vi "test_232_gnss.vi"() -> ()   [LabVIEW 2019]
uses:
  <vilib>/Instr/_visa.llb/VISA Configure Serial Port (Instr).vi
panel:
  out "latlong":cluster{"Lat":dbl, "Long":dbl}={"Lat"=127.14783036166666, "Long"=37.29147324166667} {"Lat" format="%.7f"; "Long" format="%.7f"}
  in  "tap":enum32{"config", "UI"}(tab)=enum."UI"
  in  "Port":refnum<visa-resource-name>="COM12"
  in  "baud rate":u32=115200 caption="rate"
  in  "data_w":string
  in  "write":bool
  in  "nmea sel":string="GNGGA"
  out "r buff":u32(graph)
  out "routh graph":cluster{"X":dbl, "Y":dbl}[](graph)=[{"X"=4629878.132195578, "Y"=6161955.791057685}, {"X"=4629878.449464146, "Y"=6161955.734831677}, {"X"=4629877.77406477, "Y"=6161955.64957599}, {"X"=-40080279.86596836, "Y"=-3607498.0192663614}, {"X"=4629879.260162596, "Y"=6161954.625048347}, {"X"=4629880.920363989, "Y"=6161953.906712205}, {"X"=4629882.6815418545, "Y"=6161954.279362187}, {"X"=4629885.113767498, "Y"=6161953.904911475}, {"X"=4629886.581793828, "Y"=6161953.689067744}, {"X"=4629888.648471416, "Y"=6161953.257648317}, {"X"=4629891.837990867, "Y"=6161952.403940227}, {"X"=4629892.308056162, "Y"=6161952.405785335}, {"X"=4629894.122102588, "Y"=6161951.952031529}, {"X"=4629897.047669123, "Y"=6161951.048930969}, {"X"=4629898.708113114, "Y"=6161950.608671173}, {"X"=4629900.550342631, "Y"=6161950.051971145}, {"X"=4629901.189738788, "Y"=6161949.965742772}, {"X"=4629902.101991517, "Y"=6161949.777960734}, {"X"=4629902.580381478, "Y"=6161949.687860983}, {"X"=4629904.337754514, "Y"=6161949.082264796}, {"X"=4629904.099145318, "Y"=6161949.2176907025}, {"X"=4629903.910121916, "Y"=6161949.322896625}, {"X"=4629904.728262869, "Y"=6161949.059576349}, {"X"=4629904.71638631, "Y"=6161949.095744023}, {"X"=4629903.057750786, "Y"=6161949.729303071}, {"X"=4629902.125000439, "Y"=6161950.056897599}, {"X"=4629901.877677887, "Y"=6161950.102282455}, {"X"=4629900.508252705, "Y"=6161950.654569676}, {"X"=4629899.9351718, "Y"=6161950.885176793}, {"X"=4629899.610600269, "Y"=6161951.011790283}, {"X"=4629898.414496481, "Y"=6161951.466995624}, {"X"=4629896.293106944, "Y"=6161952.299401729}, {"X"=4629894.940021647, "Y"=6161952.8599878205}, {"X"=4629893.374231298, "Y"=6161953.508735974}, {"X"=4629893.123720632, "Y"=6161953.679981945}, {"X"=4629891.816966376, "Y"=6161954.268541237}, {"X"=4629890.690365486, "Y"=6161954.77363618}, {"X"=4629889.518692982, "Y"=6161955.283432873}, {"X"=4629888.208123607, "Y"=6161955.87549565}, {"X"=4629886.6607548045, "Y"=6161956.478138071}, {"X"=4629884.424110745, "Y"=6161957.362093169}, {"X"=4629882.142841088, "Y"=6161958.178207771}, {"X"=4629880.10961531, "Y"=6161958.942958145}, {"X"=4629876.763268662, "Y"=6161960.222086402}, {"X"=4629875.049360155, "Y"=6161960.899303025}, {"X"=4629873.687762832, "Y"=6161961.454930634}, {"X"=4629871.788337784, "Y"=6161962.206068063}, {"X"=4629870.044529555, "Y"=6161962.864822832}, {"X"=4629867.847281659, "Y"=6161963.742002078}, {"X"=4629865.492343957, "Y"=6161964.648225941}, {"X"=4629863.853090226, "Y"=6161965.295558696}, {"X"=4629861.3459862, "Y"=6161966.254256366}, {"X"=4629859.936836349, "Y"=6161966.800689901}, {"X"=4629858.328618521, "Y"=6161967.411058061}, {"X"=4629857.052957142, "Y"=6161967.939720747}, {"X"=4629855.018113156, "Y"=6161968.737436315}, {"X"=4629853.567006, "Y"=6161969.314834981}, {"X"=4629852.811182082, "Y"=6161969.652750687}, {"X"=4629851.080375776, "Y"=6161970.33359649}, {"X"=4629849.302975364, "Y"=6161971.033939988}, {"X"=4629848.341258848, "Y"=6161971.414416122}, {"X"=4629847.05970336, "Y"=6161971.875314868}, {"X"=4629846.649667655, "Y"=6161972.050812745}, {"X"=4629845.742444542, "Y"=6161972.455482167}, {"X"=4629845.578141564, "Y"=6161972.556344009}, {"X"=4629845.343604999, "Y"=6161972.640616184}, {"X"=4629845.508885839, "Y"=6161972.50974696}, {"X"=4629845.933671053, "Y"=6161972.328983656}, {"X"=4629845.530368419, "Y"=6161972.485337485}, {"X"=4629845.479778372, "Y"=6161972.462731004}, {"X"=4629846.166837049, "Y"=6161972.1791017605}, {"X"=4629846.048558273, "Y"=6161972.174229832}, {"X"=4629846.390936594, "Y"=6161971.926570153}, {"X"=4629846.633775287, "Y"=6161971.801120852}, {"X"=4629846.453803427, "Y"=6161971.832019079}, {"X"=4629844.512919658, "Y"=6161972.565709774}, {"X"=4629843.713003393, "Y"=6161972.948996301}, {"X"=4629843.653811086, "Y"=6161972.91246725}, {"X"=4629843.375546568, "Y"=6161972.984217936}, {"X"=4629843.0636667805, "Y"=6161973.04240005}, {"X"=4629843.054895364, "Y"=6161973.014415348}, {"X"=4629842.666514361, "Y"=6161973.120696423}, {"X"=4629843.73905505, "Y"=6161972.628860625}, {"X"=4629844.410944811, "Y"=6161972.32521103}, {"X"=4629844.012114671, "Y"=6161972.416223608}, {"X"=4629845.253777034, "Y"=6161971.90422041}, {"X"=4629845.69336483, "Y"=6161971.703197987}, {"X"=4629846.419108165, "Y"=6161971.383700272}, {"X"=4629848.116545459, "Y"=6161970.716197785}, {"X"=4629848.289710002, "Y"=6161970.546360681}, {"X"=4629847.875889777, "Y"=6161970.564789061}, {"X"=4629848.5350280665, "Y"=6161970.175535598}, {"X"=4629848.471711944, "Y"=6161970.095168157}, {"X"=4629849.06439489, "Y"=6161969.810969084}, {"X"=4629849.841077642, "Y"=6161969.404897415}, {"X"=4629851.02643786, "Y"=6161968.89924651}, {"X"=4629851.683390104, "Y"=6161968.59438242}, {"X"=4629850.83990258, "Y"=6161968.794499699}, {"X"=4629851.007873055, "Y"=6161968.668487317}, {"X"=4629851.2084394125, "Y"=6161968.518731365}, {"X"=4629852.986614741, "Y"=6161967.769917846}, {"X"=4629854.014793199, "Y"=6161967.362993518}, {"X"=4629853.999855399, "Y"=6161967.318597856}, {"X"=4629855.717647278, "Y"=6161966.583931683}, {"X"=4629855.455590642, "Y"=6161966.634754253}, {"X"=4629854.855712144, "Y"=6161966.790501498}, {"X"=4629857.67515408, "Y"=6161965.669880756}, {"X"=4629857.107967277, "Y"=6161965.838523826}, {"X"=4629856.293048317, "Y"=6161966.090185709}]
  out "error out":errorcluster={"status"=FALSE, "code"=1073676294, "source"="test_232_gnss.vi 안에 VISA 읽기"} caption="에러 출력"
  out "버퍼 읽기":string
  out "val":bool
  in  "data-const":bool=TRUE
  out "문자열":string="$GNRMC,065633.00,A,3717.4853459,N,12708.8775848,E,1.804,110.01,190421,,,A,V*09\r\n$GNVTG,110.01,T,,M,1.804,N,3.340,K,A*2B\r\n$GNGGA,065633.00,3717.4853459,N,12708.8775848,E,1,05,3.98,176.567,M,18.960,M,,*47\r\n$GNGSA,A,3,14,28,30,07,,,,,,,,,8.28,3.98,7.26,1*09\r\n$GNGSA,A,3,88,,,,,,,,,,,,8.28,3.98,7.26,2*01\r\n$GNGSA,A,3,,,,,,,,,,,,,8.28,3.98,7.26,3*00\r\n$GNGSA,A,3,,,,,,,,,,,,,8.28,3.98,7.26,4*07\r\n$GPGSV,2,1,06,07,18,203,14,14,55,312,32,19,08,276,12,28,46,315,29,1*6B\r\n$GPGSV,2,2,06,30,33,243,36,41,27,238,30,1*6B\r\n$GPGSV,1,1,02,14,55,312,15,30,33,243,24,6*60\r\n$GPGSV,1,1,01,08,30,078,,0*50\r\n$GLGSV,1,1,04,78,65,279,31,81,26,262,35,88,61,326,33,,,,38,1*48\r\n$GLGSV,1,1,02,65,10,116,20,78,65,279,28,3*74\r\n$GLGSV,1,1,04,71,06,028,,72,16,073,,77,38,182,,87,40,030,,0*79\r\n$GAGSV,1,1,00,0*74\r\n$GBGSV,1,1,00,0*77\r\n$GNGLL,3717.4853459,N,12708.8775848,E,065633.00,A,A*77\r\n$GNRMC,065634.00,A,3717.4853546,N,12708.8776952,E,1.769,108.08,190421,,,A,V*0C\r\n$GNVTG,108.08,T,,M,1.769,N,3.276,K,A*2B\r\n$GNGGA,065634.00,3717.4853546,N,12708.8776952,E,1,05,3.98,176.044,M,18.960,M,,*42\r\n$GNGSA,A,3,14,28,30,07,,,,,,,,,8.28,3.98,7.26,1*09\r\n$GNGSA,A,3,88,,,,,,,,,,,,8.28,3.98,7.26,2*01\r\n$GNGSA,A,3,,,,,,,,,,,,,8.28,3.98,7.26,3*00\r\n$GNGSA,A,3,,,,,,,,,,,,,8.28,3.98,7.26,4*07\r\n$GPGSV,2,1,06,07,18,203,13,14,55,312,33,19,08,276,08,28,46,315,29,1*66\r\n$GPGSV,2,2,06,30,33,243,36,41,27,238,30,1*6B\r\n$GPGSV,1,1,02,14,55,312,15,30,33,243,24,6*60\r\n$GPGSV,1,1,01,08,30,078,,0*50\r\n$GLGSV,1,1,04,78,65,279,30,81,26,262,35,88,61,326,33,,,,36,1*47\r\n$GLGSV,1,1,02,65,10,116,18,78,65,279,27,3*70\r\n$GLGSV,1,1,04,71,06,028,,72,16,073,,77,38,182,,87,40,030,,0*79\r\n$GAGSV,1,1,00,0*74\r\n$GBGSV,1,1,00,0*77\r\n$GNGLL,3717.4853546,N,12708.8776952,E,065634.00,A,A*76\r\n$GNRMC,065635.00,A,3717.4852198,N,12708.8774654,E,1.118,,190421,,,A,V*1F\r\n$GNVTG,,T,,M,1.118,N,2.071,K,A*30\r\n$GNGGA,065635.00,3717.4852198,N,12708.8774654,E,1,06,3.35,177.168,M,18.960,M,,*44\r\n$GNGSA,A,3,14,28,30,07,,,,,,,,,6.98,3.35,6.12,1*0D\r\n$GNGSA,A,3,88,81,,,,,,,,,,,6.98,3.35,6.12,2*0C\r\n$GNGSA,A,3,,,,,,,,,,,,,6.98,3.35,6.12,3*04\r\n$GNGSA,A,3,,,,,,,,,,,,,6.98,3.35,6.12,4*03\r\n$GPGSV,2,1,06,07,18,203,11,14,55,312,32,19,08,276,10,28,46,315,29,1*6C\r\n$GPGSV,2,2,06,30,33,243,35,41,27,238,30,1*68\r\n$GPGSV,1,1,02,14,55,312,15,30,33,243,25,6*61\r\n$GPGSV,1,1,01,08,30,078,,0*50\r\n$GLGSV,1,1,04,78,65,279,29,81,26,262,33,88,61,326,32,,,,35,1*4B\r\n$GLGSV,1,1,02,65,10,116,18,78,65,279,27,3*70\r\n$GLGSV,1,1,04,71,06,028,,72,16,073,,77,38,182,,87,40,030,,0*79\r\n$GAGSV,1,1,00,0*74\r\n$GBGSV,1,1,00,0*77\r\n$GNGLL,3717.4852198,N,12708.8774654,E,065635.00,A,A*7A\r\n$GNRMC,065636.00,V,,,,,,,190421,,,N,V*16\r\n$GNVTG,,,,,,,,,N*2E\r\n$GNGGA,065636.00,,,,,0,05,15.13,,,,,,*7B\r\n$GNGSA,A,1,14,28,30,,,,,,,,,,25.70,15.13,20.78,1*34\r\n$GNGSA,A,1,88,81,,,,,,,,,,,25.70,15.13,20.78,2*32\r\n$GNGSA,A,1,,,,,,,,,,,,,25.70,15.13,20.78,3*3A\r\n$GNGSA,A,1,,,,,,,,,,,,,25.70,15.13,20.78,4*3D\r\n$GPGSV,2,1,06,07,18,203,09,14,55,312,33,19,08,276,13,28,46,315,30,1*6F\r\n$GPGSV,2,2,06,30,33,243,36,41,27,238,30,1*6B\r\n$GPGSV,1,1,02,14,55,312,14,30,33,243,25,6*60\r\n$GPGSV,1,1,01,08,30,078,,0*50\r\n$GLGSV,1,1,04,78,65,279,29,81,26,263,33,88,61,326,31,,,,35,1*49\r\n$GLGSV,1,1,02,65,10,116,18,78,65,279,28,3*7F\r\n$GLGSV,1,1,04,71,06,028,,72,16,073,,77,38,182,,87,40,030,,0*79\r\n$GAGSV,1,1,00,0*74\r\n$GBGSV,1,1,00,0*77\r\n$GNGLL,,,,,065636.00,V,N*54\r\n$GNRMC,065637.00,A,3717.4848287,N,12708.8780019,E,1.079,,190421,,,A,V*19\r\n$GNVTG,,T,,M,1.079,N,1.998,K,A*3B\r\n$GNGGA,065637.00,3717.4848287,N,12708.8780019,E,1,06,3.35,178.648,M,18.960,M,,*4E\r\n$GNGSA,A,3,14,28,30,07,,,,,,,,,6.98,3.35,6.13,1*0C\r\n$GNGSA,A,3,88,81,,,,,,,,,,,6.98,3.35,6.13,2*0D\r\n$GNGSA,A,3,,,,,,,,,,,,,6.98,3.35,6.13,3*05\r\n$GNGSA,A,3,,,,,,,,,,,,,6.98,3.35,6.13,4*02\r\n$GPGSV,2,1,06,07,18,203,10,14,55,312,33,19,08,276,12,28,46,315,30,1*66\r\n$GPGSV,2,2,06,30,33,243,35,41,27,238,30,1*68\r\n$GPGSV,1,1,02,14,55,312,14,30,33,243,25,6*60\r\n$GPGSV,1,1,01,08,30,078,,0*50\r\n$GLGSV,1,1,04,78,65,279,28,81,26,263,32,88,61,326,31,,,,34,1*48\r\n$GLGSV,1,1,02,65,10,116,19,78,65,279,28,3*7E\r\n$GLGSV,1,1,04,71,06,028,,72,16,073,,77,37,182,,87,40,030,,0*76\r\n$GAGSV,1,1,00,0*74\r\n$GBGSV,1,1,00,0*77\r\n$GNGLL,3717.4848287,N,12708.8780019,E,065637.00,A,A*7A\r\n$GNRMC,065638.00,A,3717.4846336,N,12708.8785904,E,1.071,,190421,,,A,V*1B\r\n$GNVTG,,T,,M,1.071,N,1.983,K,A*39\r\n$GNGGA,065638.00,3717.4846336,N,12708.8785904,E,1,05,3.45,179.021,M,18.960,M,,*48\r\n$GNGSA,A,3,14,28,30,07,,,,,,,,,7.40,3.45,6.55,1*0D\r\n$GNGSA,A,3,81,,,,,,,,,,,,7.40,3.45,6.55,2*0C\r\n$GNGSA,A,3,,,,,,,,,,,,,7.40,3.45,6.55,3*04\r\n$GNGSA,A,3,,,,,,,,,,,,,7.40,3.45,6.55,4*03\r\n$GPGSV,2,1,06,07,18,203,11,14,55,312,33,19,08,276,11,28,46,315,30,1*64\r\n$GPGSV,2,2,06,30,33,243,36,41,27,238,30,1*6B\r\n$GPGSV,1,1,02,14,55,312,16,30,33,243,24,6*63\r\n$GPGSV,1,1,01,08,30,078,,0*50\r\n$GLGSV,1,1,02,81,26,263,32,,,,34,1*46\r\n$GLGSV,1,1,03,65,10,116,19,78,65,278,28,88,61,326,19,3*46\r\n$GLGSV,1,1,04,71,06,028,,72,16,073,,77,37,182,,87,40,030,,0*76\r\n$GAGSV,1,1,00,0*74\r\n$GBGSV,1,1,00,0*77\r\n$GNGLL,3717.4846336,N,12708.8785904,E,065638.00,A,A*70\r\n$GNRMC,065639.00,A,3717.4850704,N,12708.8791858,E,1.002,100.47,190421,,,A,V*0D\r\n$GNVTG,100.47,T,,M,1.002,N,1.855,K,A*2B\r\n$GNGGA,065639.00,3717.4850704,N,12708.8791858,E,1,06,2.35,176.270,M,18.960,M,,*4A\r\n$GNGSA,A,3,14,28,30,07,,,,,,,,,3.41,2.35,2.46,1*08\r\n$GNGSA,A,3,79,81,,,,,,,,,,,3.41,2.35,2.46,2*07\r\n$GNGSA,A,3,,,,,,,,,,,,,3.41,2.35,2.46,3*01\r\n$GNGSA,A,3,,,,,,,,,,,,,3.41,2.35,2.46,4*06\r\n$GPGSV,2,1,06,07,18,203,12,14,55,312,33,19,08,276,10,28,46,315,29,1*6E\r\n$GPGSV,2,2,06,30,33,243,35,41,27,238,30,1*68\r\n$GPGSV,1,1,02,14,55,312,17,30,33,243,24,6*62\r\n$GPGSV,1,1,01,08,30,078,,0*50\r\n$GLGSV,1,1,02,79,,,34,81,26,263,33,1*49\r\n$GLGSV,1,1,03,65,10,116,19,78,65,278,28,88,61,326,18,3*47\r\n$GLGSV,1,1,04,71,06,028,,72,16,073,,77,37,182,,87,40,030,,0*76\r\n$GAGSV,1,1,00,0*74\r\n$GBGSV,1,1,00,0*77\r\n$GNGLL,3717.4850704,N,12708.8791858,E,065639.00,A,A*7E\r\n$GNRMC,065640.00,A,3717.4851692,N,12708.8800307,E,1.093,103.53,190421,,,A,V*04\r\n$GNVTG,103.53,T,,M,1.093,N,2.024,K,A*28\r\n$GNGGA,065640.00,3717.4851692,N,12708.8800307,E,1,06,2.35,175.043,M,18.960,M,,*4C\r\n$GNGSA,A,3,14,28,30,07,,,,,,,,,3.41,2.35,2.46,1*08\r\n$GNGSA,A,3,79,81,,,,,,,,,,,3.41,2.35,2.46,2*07\r\n$GNGSA,A,3,,,,,,,,,,,,,3.41,2.35,2.46,3*01\r\n$GNGSA,A,3,,,,,,,,,,,,,3.41,2.35,2.46,4*06\r\n$GPGSV,2,1,06,07,18,203,13,14,55,312,33,19,08,276,11,28,46,315,30,1*66\r\n$GPGSV,2,2,06,30,33,243,36,41,27,238,30,1*6B\r\n$GPGSV,1,1,02,14,55,312,17,30,33,243,24,6*62\r\n$GPGSV,1,1,01,08,30,078,,0*50\r\n$GLGSV,1,1,02,79,22,328,35,81,26,263,34,1*76\r\n$GLGSV,1,1,04,65,10,116,19,78,65,278,27,79,22,328,27,88,61,326,19,3*7C\r\n$GLGSV,1,1,04,71,06,028,,72,16,073,,77,37,182,,87,40,030,,0*76\r\n$GAGSV,1,1,00,0*74\r\n$GBGSV,1,1,00,0*77\r\n$GNGLL,3717.4851692,N,12708.8800307,E,065640.00,A,A*79\r\n$GNRMC,065641.00,A,3717.4852346,N,12708.8805404,E,0.968,104.12,190421,,,A,V*05\r\n$GNVTG,104.12,T,,M,0.968,N,1.792,K,A*2F\r\n$GNGGA,065641.00,3717.4852346,N,12708.8805404,E,1,07,2.17,174.523,M,18.960,M,,*40\r\n$GNGSA,A,3,14,28,30,07,,,,,,,,,3.08,2.17,2.19,1*0F\r\n$GNGSA,A,3,79,88,81,,,,,,,,,,3.08,2.17,2.19,2*00\r\n$GNGSA,A,3,,,,,,,,,,,,,3.08,2.17,2.19,3*06\r\n$GNGSA,A,3,,,,,,,,,,,,,3.08,2.17,2.19,4*01\r\n$GPGSV,2,1,06,07,18,203,15,14,55,312,34,19,08,276,11,28,46,315,31,1*66\r\n$GPGSV,2,2,06,30,33,243,36,41,27,238,31,1*6A\r\n$GPGSV,1,1,02,14,55,312,15,30,33,243,23,6*67\r\n$GPGSV,1,1,01,08,30,078,,0*50\r\n$GLGSV,1,1,02,79,22,328,35,81,26,263,34,1*76\r\n$GLGSV,1,1,04,65,10,116,18,78,65,278,28,79,22,328,27,88,61,326,20,3*78\r\n$GLGSV,1,1,04,71,06,028,,72,16,073,,77,37,182,,87,40,030,,0*76\r\n$GAGSV,1,1,00,0*74\r\n$GBGSV,1,1,00,0*77\r\n$GNGLL,3717.4852346,N,12708.8805404,E,065641.00,A,A*76\r\n$GNRMC,065642.00,A,3717.4852543,N,12708.8812612,E,0.932,106.63,190421,,,A,V*0D\r\n$GNVTG,106.63,T,,M,0.932,N,1.726,K,A*2B\r\n$GNGGA,065642.00,3717.4852543,N,12708.8812612,E,1,06,2.17,173.748,M,18.960,M,,*4A\r\n$GNGSA,A,3,14,28,30,07,,,,,,,,,3.08,2.17,2.19,1*0F\r\n$GNGSA,A,3,79,88,81,,,,,,,,,,3.08,2.17,2.19,2*00\r\n$GNGSA,A,3,,,,,,,,,,,,,3.08,2.17,2.19,3*06\r\n$GNGSA,A,3,,,,,,,,,,,,,3.08,2.17,2.19,4*01\r\n$GPGSV,2,1,06,07,18,203,15,14,55,312,33,19,08,276,17,28,46,315,31,1*67\r\n$GPGSV,2,2,06,30,33,243,36,41,27,238,31,1*6A\r\n$GPGSV,1,1,02,14,55,312,14,30,33,243,22,6*67\r\n$GPGSV,1,1,01,08,30,078,,0*50\r\n$GLGSV,1,1,02,79,22,328,35,81,26,263,34,1*76\r\n$GLGSV,1,1,04,65,10,116,17,78,65,278,28,79,22,328,28,88,61,326,20,3*78\r\n$GLGSV,1,1,04,71,06,028,,72,16,073,,77,37,182,,87,40,030,,0*76\r\n$GAGSV,1,1,00,0*74\r\n$GBGSV,1,1,00,0*77\r\n$GNGLL,3717.4852543,N,12708.8812612,E,065642.00,A,A*75\r\n$GNRMC,065643.00,A,3717.4851781,N,12708.8823784,E,1.067,109.96,190421,,,A,V*02\r\n$GNVTG,109.96,T,,M,1.067,N,1.977,K,A*2C\r\n$GNGGA,065643.00,3717.4851781,N,12708.8823784,E,1,06,2.17,172.534,M,18.960,M,,*40\r\n$GNGSA,A,3,14,28,30,07,,,,,,,,,3.08,2.17,2.19,1*0F\r\n$GNGSA,A,3,79,88,81,,,,,,,,,,3.08,2.17,2.19,2*00\r\n$GNGSA,A,3,,,,,,,,,,,,,3.08,2.17,2.19,3*06\r\n$GNGSA,A,3,,,,,,,,,,,,,3.08,2.17,2.19,4*01\r\n$GPGSV,2,1,06,07,18,203,16,14,55,312,33,19,08,276,14,28,46,315,31,1*67\r\n$GPGSV,2,2,06,30,33,243,36,41,27,238,30,1*6B\r\n$GPGSV,1,1,02,14,55,312,14,30,33,243,22,6*67\r\n$GPGSV,1,1,01,08,30,078,,0*50\r\n$GLGSV,1,1,02,79,22,328,35,81,26,263,33,1*71\r\n$GLGSV,1,1,04,65,10,116,18,78,65,278,27,79,22,328,27,88,61,326,21,3*76\r\n$GLGSV,1,1,04,71,06,028,,72,16,073,,77,37,182,,87,40,030,,0*76\r\n$GAGSV,1,1,00,0*74\r\n$GBGSV,1,1,00,0*77\r\n$GNGLL,3717.4851781,N,12708.8823784,E,065643.00,A,A*77\r\n$GNRMC,065644.00,A,3717.4852393,N,12708.8825398,E,0.808,106.82,190421,,,A,V*04\r\n$GNVTG,106.82,T,,M,0.808,N,1.497,K,A*25\r\n$GNGGA,065644.00,3717.4852393,N,12708.8825398,E,1,06,2.17,172.407,M,18.960,M,,*4D\r\n$GNGSA,A,3,14,28,30,07,,,,,,,,,3.08,2.17,2.19,1*0F\r\n$GNGSA,A,3,79,88,81,,,,,,,,,,3.08,2.17,2.19,2*00\r\n$GNGSA,A,3,,,,,,,,,,,,,3.08,2.17,2.19,3*06\r\n$GNGSA,A,3,,,,,,,,,,,,,3.08,2.17,2.19,4*01\r\n$GPGSV,2,1,06,07,18,203,15,14,55,312,33,19,08,276,13,28,46,315,31,1*63\r\n$GPGSV,2,2,06,30,33,243,36,41,27,238,30,1*6B\r\n$GPGSV,1,1,02,14,55,312,14,30,33,243,21,6*64\r\n$GPGSV,1,1,01,08,30,078,,0*50\r\n$GLGSV,1,1,02,79,22,328,35,81,26,263,34,1*76\r\n$GLGSV,1,1,04,65,10,116,18,78,65,278,27,79,22,328,28,88,61,326,20,3*78\r\n$GLGSV,1,1,04,71,06,028,,72,16,073,,77,37,182,,87,40,030,,0*76\r\n$GAGSV,1,1,00,0*74\r\n$GBGSV,1,1,00,0*77\r\n$GNGLL,3717.4852393,N,12708.8825398,E,065644.00,A,A*7B\r\n$GNRMC,065645.00,A,3717.4852140,N,12708.8831744,E,0.831,110.97,190421,,,A,V*00\r\n$GNVTG,110.97,T,,M,0.831,N,1.540,K,A*27\r\n$GNGGA,065645.00,3717.4852140,N,12708.8831744,E,1,06,2.17,171.708,M,18.960,M,,*4F\r\n$GNGSA,A,3,14,28,30,07,,,,,,,,,3.08,2.17,2.19,1*0F\r\n$GNGSA,A,3,79,88,81,,,,,,,,,,3.08,2.17,2.19,2*00\r\n$GNGSA,A,3,,,,,,,,,,,,,3.08,2.17,2.19,3*06\r\n$GNGSA,A,3,,,,,,,,,,,,,3.08,2.17,2.19,4*01\r\n$GPGSV,2,1,06,07,18,203,15,14,55,312,33,19,08,276,12,28,46,315,31,1*62\r\n$GPGSV,2,2,06,30,33,243,36,41,27,238,30,1*6B\r\n$GPGSV,1,1,02,14,55,312,15,30,33,243,21,6*65\r\n$GPGSV,1,1,01,08,30,078,,0*50\r\n$GLGSV,1,1,02,79,22,328,36,81,26,263,34,1*75\r\n$GLGSV,1,1,04,65,10,116,18,78,65,278,27,79,22,328,27,88,61,326,20,3*77\r\n$GLGSV,1,1,04,71,06,028,,72,16,073,,77,37,182,,87,40,030,,0*76\r\n$GAGSV,1,1,00,0*74\r\n$GBGSV,1,1,00,0*77\r\n$GNGLL,3717.4852140,N,12708.8831744,E,065645.00,A,A*76\r\n$GNRMC,065646.00,A,3717.4850760,N,12708.8842022,E,0.997,108.55,190421,,,A,V*0C\r\n$GNVTG,108.55,T,,M,0.997,N,1.846,K,A*26\r\n$GNGGA,065646.00,3717.4850760,N,12708.8842022,E,1,06,2.17,171.089,M,18.960,M,,*47\r\n$GNGSA,A,3,14,28,30,07,,,,,,,,,3.08,2.17,2.19,1*0F\r\n$GNGSA,A,3,79,88,81,,,,,,,,,,3.08,2.17,2.19,2*00\r\n$GNGSA,A,3,,,,,,,,,,,,,3.08,2.17,2.19,3*06\r\n$GNGSA,A,3,,,,,,,,,,,,,3.08,2.17,2.19,4*01\r\n$GPGSV,2,1,06,07,18,203,15,14,55,312,34,19,08,276,09,28,46,315,31,1*6F\r\n$GPGSV,2,2,06,30,33,243,36,41,27,238,31,1*6A\r\n$GPGSV,1,1,02,14,55,312,15,30,33,243,20,6*64\r\n$GPGSV,1,1,01,08,30,078,,0*50\r\n$GLGSV,1,1,02,79,22,328,36,81,26,263,34,1*75\r\n$GLGSV,1,1,04,65,10,116,18,78,65,278,27,79,22,328,27,88,61,326,21,3*76\r\n$GLGSV,1,1,04,71,06,028,,72,16,073,,77,37,182,,87,40,030,,0*76\r\n$GAGSV,1,1,00,0*74\r\n$GBGSV,1,1,00,0*77\r\n$GNGLL,3717.4850760,N,12708.8842022,E,065646.00,A,A*70\r\n$GNRMC,065647.00,A,3717.4850387,N,12708.8847837,E,0.979,109.12,190421,,,A,V*0B\r\n$GNVTG,109.12,T,,M,0.979,N,1.813,K,A*24\r\n$GNGGA,065647.00,3717.4850387,N,12708.8847837,E,1,06,2.17,170.569,M,18.960,M,,*48\r\n$GNGSA,A,3,14,28,30,07,,,,,,,,,3.08,2.17,2.19,1*0F\r\n$GNGSA,A,3,79,88,81,,,,,,,,,,3.08,2.17,2.19,2*00\r\n$GNGSA,A,3,,,,,,,,,,,,,3.08,2.17,2.19,3*06\r\n$GNGSA,A,3,,,,,,,,,,,,,3.08,2.17,2.19,4*01\r\n$GPGSV,2,1,06,07,18,203,16,14,55,312,33,19,08,276,12,28,46,315,30,1*60\r\n$GPGSV,2,2,06,30,33,243,36,41,27,238,31,1*6A\r\n$GPGSV,1,1,02,14,55,312,15,30,33,243,21,6*65\r\n$GPGSV,1,1,01,08,30,078,,0*50\r\n$GLGSV,1,1,02,79,22,328,37,81,26,263,34,1*74\r\n$GLGSV,1,1,04,65,10,116,18,78,65,278,28,79,22,328,27,88,61,327,20,3*79\r\n$GLGSV,1,1,04,71,06,028,,72,16,073,,77,37,182,,87,40,030,,0*76\r\n$GAGSV,1,1,00,0*74\r\n$GBGSV,1,1,00,0*77\r\n$GNGLL,3717.4850387,N,12708.8847837,E,065647.00,A,A*75\r\n$GNRMC,065648.00,A,3717.4849586,N,12708.8854306,E,0.899,106.80,190421,,,A,V*0B\r\n$GNVTG,106.80,T,,M,0.899,N,1.665,K,A*20\r\n$GNGGA,065648.00,3717.4849586,N,12708.8854306,E,1,07,2.17,170.188,M,18.960,M,,*49\r\n$GNGSA,A,3,14,28,30,07,,,,,,,,,3.08,2.17,2.19,1*0F\r\n$GNGSA,A,3,79,88,81,,,,,,,,,,3.08,2.17,2.19,2*00\r\n$GNGSA,A,3,,,,,,,,,,,,,3.08,2.17,2.19,3*06\r\n$GNGSA,A,3,,,,,,,,,,,,,3.08,2.17,2.19,4*01\r\n$GPGSV,2,1,06,07,18,203,16,14,55,312,33,19,08,276,15,28,46,315,30,1*67\r\n$GPGSV,2,2,06,30,33,243,35,41,27,238,30,1*68\r\n$GPGSV,1,1,02,14,55,312,16,30,33,243,22,6*65\r\n$GPGSV,1,1,01,08,30,078,,0*50\r\n$GLGSV,1,1,02,79,22,328,36,81,26,263,34,1*75\r\n$GLGSV,1,1,03,78,65,278,28,79,22,328,26,88,61,327,21,3*43\r\n$GLGSV,2,1,05,65,10,116,,71,06,028,,72,16,073,,77,37,182,,0*78\r\n$GLGSV,2,2,05,77,37,182,,0*43\r\n$GAGSV,1,1,00,0*74\r\n$GBGSV,1,1,00,0*77\r\n$GNGLL,3717.4849586,N,12708.8854306,E,065648.00,A,A*7E\r\n$GNRMC,065649.00,A,3717.4849915,N,12708.8856524,E,0.825,103.07,190421,,,A,V*05\r\n$GNVTG,103.07,T,,M,0.825,N,1.527,K,A*28\r\n$GNGGA,065649.00,3717.4849915,N,12708.8856524,E,1,06,2.17,169.994,M,18.960,M,,*46\r\n$GNGSA,A,3,14,28,30,07,,,,,,,,,3.08,2.17,2.19,1*0F\r\n$GNGSA,A,3,79,88,81,,,,,,,,,,3.08,2.17,2.19,2*00\r\n$GNGSA,A,3,,,,,,,,,,,,,3.08,2.17,2.19,3*06\r\n$GNGSA,A,3,,,,,,,,,,,,,3.08,2.17,2.19,4*01\r\n$GPGSV,2,1,06,07,18,203,15,14,55,312,33,19,08,276,11,28,46,315,29,1*68\r\n$GPGSV,2,2,06,30,33,243,35,41,27,238,31,1*69\r\n$GPGSV,1,1,02,14,55,312,17,30,33,243,22,6*64\r\n$GPGSV,1,1,01,08,30,078,,0*50\r\n$GLGSV,1,1,02,79,22,328,36,81,26,263,33,1*72\r\n$GLGSV,1,1,04,78,65,278,27,79,22,328,26,81,26,263,19,88,61,327,21,3*79\r\n$GLGSV,2,1,05,65,10,116,,71,06,028,,72,16,073,,77,37,182,,0*78\r\n$GLGSV,2,2,05,77,37,182,,0*43\r\n$GAGSV,1,1,00,0*74\r\n$GBGSV,1,1,00,0*77\r\n$GNGLL,3717.4849915,N,12708.8856524,E,065649.00,A,A*7D\r\n$GNRMC,065650.00,A,3717.4850017,N,12708.8859705,E,0.780,,190421,,,A,V*1B\r\n$GNVTG,,T,,M,0.780,N,1.444,K,A*37\r\n$GNGGA,065650.00,3717.4850017,N,12708.8859705,E,1,06,2.17,169.716,M,18.960,M,,*47\r\n$GNGSA,A,3,14,28,30,07,,,,,,,,,3.08,2.17,2.19,1*0F\r\n$GNGSA,A,3,79,88,81,,,,,,,,,,3.08,2.17,2.19,2*00\r\n$GNGSA,A,3,,,,,,,,,,,,,3.08,2.17,2.19,3*06\r\n$GNGSA,A,3,,,,,,,,,,,,,3.08,2.17,2.19,4*01\r\n$GPGSV,2,1,06,07,18,203,14,14,55,312,33,19,08,276,14,28,46,315,28,1*6D\r\n$GPGSV,2,2,06,30,33,243,35,41,27,238,31,1*69\r\n$GPGSV,1,1,02,14,55,312,18,30,33,243,22,6*6B\r\n$GPGSV,1,1,01,08,30,078,,0*50\r\n$GLGSV,1,1,02,79,22,328,36,81,26,263,33,1*72\r\n$GLGSV,1,1,04,78,65,278,27,79,22,328,26,81,26,263,19,88,61,327,20,3*78\r\n$GLGSV,2,1,05,65,10,116,,71,06,028,,72,16,073,,77,37,182,,0*78\r\n$GLGSV,2,2,05,77,37,182,,0*43\r\n$GAGSV,1,1,00,0*74\r\n$GBGSV,1,1,00,0*77\r\n$GNGLL,3717.4850017,N,12708.8859705,E,065650.00,A,A*78\r\n$GNRMC,065651.00,A,3717.4850118,N,12708.8861371,E,0.670,,190421,,,A,V*16\r\n$GNVTG,,T,,M,0.670,N,1.240,K,A*3B\r\n$GNGGA,065651.00,3717.4850118,N,12708.8861371,E,1,07,2.17,169.601,M,18.960,M,,*42\r\n$GNGSA,A,3,14,28,30,07,,,,,,,,,3.08,2.17,2.19,1*0F\r\n$GNGSA,A,3,79,88,81,,,,,,,,,,3.08,2.17,2.19,2*00\r\n$GNGSA,A,3,,,,,,,,,,,,,3.08,2.17,2.19,3*06\r\n$GNGSA,A,3,,,,,,,,,,,,,3.08,2.17,2.19,4*01\r\n$GPGSV,2,1,06,07,18,203,14,14,55,312,33,19,08,276,08,28,46,315,28,1*60\r\n$GPGSV,2,2,06,30,33,243,35,41,27,238,30,1*68\r\n$GPGSV,1,1,02,14,55,312,17,30,33,243,23,6*65\r\n$GPGSV,1,1,01,08,30,078,,0*50\r\n$GLGSV,1,1,02,79,22,328,35,81,26,263,33,1*71\r\n$GLGSV,2,1,05,65,10,116,20,78,65,278,27,79,22,328,26,81,26,263,19,3*7F\r\n$GLGSV,2,2,05,88,61,327,21,3*4D\r\n$GLGSV,1,1,04,71,06,028,,72,16,073,,77,37,182,,87,40,030,,0*76\r\n$GAGSV,1,1,00,0*74\r\n$GBGSV,1,1,00,0*77\r\n$GNGLL,3717.4850118,N,12708.8861371,E,065651.00,A,A*7B\r\n$GNRMC,065652.00,A,3717.4848931,N,12708.8867561,E,0.731,,190421,,,A,V*1A\r\n$GNVTG,,T,,M,0.731,N,1.354,K,A*3B\r\n$GNGGA,065652.00,3717.4848931,N,12708.8867561,E,1,07,2.17,169.223,M,18.960,M,,*4E\r\n$GNGSA,A,3,14,28,30,07,,,,,,,,,3.08,2.17,2.19,1*0F\r\n$GNGSA,A,3,79,88,81,,,,,,,,,,3.08,2.17,2.19,2*00\r\n$GNGSA,A,3,,,,,,,,,,,,,3.08,2.17,2.19,3*06\r\n$GNGSA,A,3,,,,,,,,,,,,,3.08,2.17,2.19,4*01\r\n$GPGSV,2,1,06,07,18,202,16,14,55,312,33,19,08,276,10,28,46,315,28,1*6A\r\n$GPGSV,2,2,06,30,33,243,35,41,27,238,31,1*69\r\n$GPGSV,1,1,02,14,55,312,16,30,33,243,23,6*64\r\n$GPGSV,1,1,01,08,30,078,,0*50\r\n$GLGSV,1,1,03,79,22,328,34,81,26,263,33,88,61,327,33,1*40\r\n$GLGSV,2,1,05,65,10,116,18,78,65,278,27,79,22,328,25,81,26,263,19,3*77\r\n$GLGSV,2,2,05,88,61,327,21,3*4D\r\n$GLGSV,1,1,04,71,06,028,,72,16,073,,77,37,182,,87,40,030,,0*76\r\n$GAGSV,1,1,00,0*74\r\n$GBGSV,1,1,00,0*77\r\n$GNGLL,3717.4848931,N,12708.8867561,E,065652.00,A,A*73\r\n$GNRMC,065653.00,A,3717.4849394,N,12708.8866707,E,0.597,,190421,,,A,V*12\r\n$GNVTG,,T,,M,0.597,N,1.105,K,A*33\r\n$GNGGA,065653.00,3717.4849394,N,12708.8866707,E,1,07,2.17,169.235,M,18.960,M,,*4F\r\n$GNGSA,A,3,14,28,30,07,,,,,,,,,3.08,2.17,2.19,1*0F\r\n$GNGSA,A,3,79,88,81,,,,,,,,,,3.08,2.17,2.19,2*00\r\n$GNGSA,A,3,,,,,,,,,,,,,3.08,2.17,2.19,3*06\r\n$GNGSA,A,3,,,,,,,,,,,,,3.08,2.17,2.19,4*01\r\n$GPGSV,2,1,06,07,18,202,17,14,55,312,33,19,08,276,10,28,46,315,29,1*6A\r\n$GPGSV,2,2,06,30,33,243,35,41,27,238,31,1*69\r\n$GPGSV,1,1,02,14,55,312,16,30,33,243,22,6*65\r\n$GPGSV,1,1,01,08,29,078,,0*58\r\n$GLGSV,1,1,03,79,22,328,34,81,26,263,33,88,61,327,32,1*41\r\n$GLGSV,2,1,05,65,10,116,17,78,65,278,26,79,22,328,25,81,26,263,18,3*78\r\n$GLGSV,2,2,05,88,61,327,20,3*4C\r\n$GLGSV,1,1,04,71,06,028,,72,16,073,,77,37,182,,87,40,030,,0*76\r\n$GAGSV,1,1,00,0*74\r\n$GBGSV,1,1,00,0*77\r\n$GNGLL,3717.4849394,N,12708.8866707,E,065653.00,A,A*75\r\n$GNRMC,065654.00,A,3717.4849749,N,12708.8866031,E,0.514,,190421,,,A,V*18\r\n$GNVTG,,T,,M,0.514,N,0.953,K,A*32\r\n$GNGGA,065654.00,3717.4849749,N,12708.8866031,E,1,07,2.17,169.195,M,18.960,M,,*47\r\n$GNGSA,A,3,14,28,30,07,,,,,,,,,3.08,2.17,2.19,1*0F\r\n$GNGSA,A,3,79,88,81,,,,,,,,,,3.08,2.17,2.19,2*00\r\n$GNGSA,A,3,,,,,,,,,,,,,3.08,2.17,2.19,3*06\r\n$GNGSA,A,3,,,,,,,,,,,,,3.08,2.17,2.19,4*01\r\n$GPGSV,2,1,06,07,18,202,18,14,55,312,33,19,08,276,14,28,46,315,29,1*61\r\n$GPGSV,2,2,06,30,33,243,34,41,27,238,31,1*68\r\n$GPGSV,1,1,02,14,55,312,16,30,33,243,22,6*65\r\n$GPGSV,1,1,01,08,29,078,,0*58\r\n$GLGSV,1,1,03,79,22,328,34,81,26,263,33,88,61,327,32,1*41\r\n$GLGSV,2,1,05,65,10,116,15,78,65,278,26,79,22,328,25,81,26,263,19,3*7B\r\n$GLGSV,2,2,05,88,61,327,20,3*4C\r\n$GLGSV,1,1,04,71,06,028,,72,16,073,,77,37,182,,87,40,030,,0*76\r\n$GAGSV,1,1,00,0*74\r\n$GBGSV,1,1,00,0*77\r\n$GNGLL,3717.4849749,N,12708.8866031,E,065654.00,A,A*74\r\n$GNRMC,065655.00,A,3717.4849302,N,12708.8868908,E,0.661,,190421,,,A,V*1E\r\n$GNVTG,,T,,M,0.661,N,1.224,K,A*39\r\n$GNGGA,065655.00,3717.4849302,N,12708.8868908,E,1,07,2.17,169.152,M,18.960,M,,*4B\r\n$GNGSA,A,3,14,28,30,07,,,,,,,,,3.08,2.17,2.19,1*0F\r\n$GNGSA,A,3,79,88,81,,,,,,,,,,3.08,2.17,2.19,2*00\r\n$GNGSA,A,3,,,,,,,,,,,,,3.08,2.17,2.19,3*06\r\n$GNGSA,A,3,,,,,,,,,,,,,3.08,2.17,2.19,4*01\r\n$GPGSV,2,1,06,07,18,202,18,14,55,312,32,19,08,276,06,28,46,315,28,1*62\r\n$GPGSV,2,2,06,30,33,243,34,41,27,238,31,1*68\r\n$GPGSV,1,1,02,14,55,312,17,30,33,243,23,6*65\r\n$GPGSV,1,1,01,08,29,078,,0*58\r\n$GLGSV,1,1,03,79,22,328,34,81,26,263,33,88,61,327,32,1*41\r\n$GLGSV,2,1,05,65,10,116,13,78,65,278,26,79,22,328,24,81,26,263,19,3*7C\r\n$GLGSV,2,2,05,88,61,327,18,3*47\r\n$GLGSV,1,1,04,71,06,028,,72,16,073,,77,37,182,,87,40,030,,0*76\r\n$GAGSV,1,1,00,0*74\r\n$GBGSV,1,1,00,0*77\r\n$GNGLL,3717.4849302,N,12708.8868908,E,065655.00,A,A*73\r\n$GNRMC,065656.00,A,3717.4849492,N,12708.8868858,E,0.462,,190421,,,A,V*16\r\n$GNVTG,,T,,M,0.462,N,0.855,K,A*35\r\n$GNGGA,065656.00,3717.4849492,N,12708.8868858,E,1,07,2.17,169.187,M,18.960,M,,*4A\r\n$GNGSA,A,3,14,28,30,07,,,,,,,,,3.08,2.17,2.19,1*0F\r\n$GNGSA,A,3,79,88,81,,,,,,,,,,3.08,2.17,2.19,2*00\r\n$GNGSA,A,3,,,,,,,,,,,,,3.08,2.17,2.19,3*06\r\n$GNGSA,A,3,,,,,,,,,,,,,3.08,2.17,2.19,4*01\r\n$GPGSV,2,1,06,07,18,202,19,14,55,312,33,19,08,276,08,28,46,315,28,1*6C\r\n$GPGSV,2,2,06,30,33,243,35,41,27,238,30,1*68\r\n$GPGSV,1,1,02,14,55,312,17,30,33,243,22,6*64\r\n$GPGSV,1,1,01,08,29,078,,0*58\r\n$GLGSV,1,1,03,79,22,328,34,81,26,263,33,88,61,327,32,1*41\r\n$GLGSV,2,1,05,65,10,116,12,78,65,278,26,79,22,328,24,81,26,263,18,3*7C\r\n$GLGSV,2,2,05,88,61,327,18,3*47\r\n$GLGSV,1,1,04,71,06,028,,72,16,073,,77,37,182,,87,40,030,,0*76\r\n$GAGSV,1,1,00,0*74\r\n$GBGSV,1,1,00,0*77\r\n$GNGLL,3717.4849492,N,12708.8868858,E,065656.00,A,A*7A\r\n$GNRMC,065657.00,A,3717.4850964,N,12708.8863000,E,0.600,,190421,,,A,V*13\r\n$GNVTG,,T,,M,0.600,N,1.111,K,A*3B\r\n$GNGGA,065657.00,3717.4850964,N,12708.8863000,E,1,07,2.17,169.080,M,18.960,M,,*4F\r\n$GNGSA,A,3,14,28,30,07,,,,,,,,,3.08,2.17,2.19,1*0F\r\n$GNGSA,A,3,79,88,81,,,,,,,,,,3.08,2.17,2.19,2*00\r\n$GNGSA,A,3,,,,,,,,,,,,,3.08,2.17,2.19,3*06\r\n$GNGSA,A,3,,,,,,,,,,,,,3.08,2.17,2.19,4*01\r\n$GPGSV,2,1,06,07,18,202,19,14,55,312,33,19,08,276,09,28,46,315,28,1*6D\r\n$GPGSV,2,2,06,30,33,243,34,41,27,238,31,1*68\r\n$GPGSV,1,1,02,14,55,312,18,30,33,243,22,6*6B\r\n$GPGSV,1,1,01,08,29,078,,0*58\r\n$GLGSV,1,1,03,79,22,328,34,81,26,263,33,88,61,327,32,1*41\r\n$GLGSV,2,1,05,65,10,116,14,78,65,278,26,79,22,328,24,81,26,263,17,3*75\r\n$GLGSV,2,2,05,88,61,327,18,3*47\r\n$GLGSV,1,1,04,71,06,028,,72,16,073,,77,37,182,,87,40,030,,0*76\r\n$GAGSV,1,1,00,0*74\r\n$GBGSV,1,1,00,0*77\r\n$GNGLL,3717.4850964,N,12708.8863000,E,065657.00,A,A*79\r\n$GNRMC,065658.00,A,3717.4851629,N,12708.8859713,E,0.578,,190421,,,A,V*1B\r\n$GNVTG,,T,,M,0.578,N,1.070,K,A*31\r\n$GNGGA,065658.00,3717.4851629,N,12708.8859713,E,1,07,2.17,168.743,M,18.960,M,,*42\r\n$GNGSA,A,3,14,28,30,07,,,,,,,,,3.08,2.17,2.19,1*0F\r\n$GNGSA,A,3,79,88,81,,,,,,,,,,3.08,2.17,2.19,2*00\r\n$GNGSA,A,3,,,,,,,,,,,,,3.08,2.17,2.19,3*06\r\n$GNGSA,A,3,,,,,,,,,,,,,3.08,2.17,2.19,4*01\r\n$GPGSV,2,1,06,07,18,202,19,14,56,312,33,19,08,276,07,28,46,315,28,1*60\r\n$GPGSV,2,2,06,30,33,243,34,41,27,238,31,1*68\r\n$GPGSV,1,1,02,14,56,312,18,30,33,243,22,6*68\r\n$GPGSV,1,1,01,08,29,078,,0*58\r\n$GLGSV,1,1,03,79,22,328,33,81,26,263,33,88,61,327,32,1*46\r\n$GLGSV,2,1,05,65,10,116,15,78,65,278,26,79,22,328,24,81,26,263,18,3*7B\r\n$GLGSV,2,2,05,88,61,327,19,3*46\r\n$GLGSV,1,1,04,71,06,028,,72,16,073,,77,37,182,,87,40,030,,0*76\r\n$GAGSV,1,1,00,0*74\r\n$GBGSV,1,1,00,0*77\r\n$GNGLL,3717.4851629,N,12708.8859713,E,065658.00,A,A*7D\r\n$GNRMC,065659.00,A,3717.4851570,N,12708.8858852,E,0.638,,190421,,,A,V*19\r\n$GNVTG,,T,,M,0.638,N,1.182,K,A*3A\r\n$GNGGA,065659.00,3717.4851570,N,12708.8858852,E,1,07,2.17,168.385,M,18.960,M,,*49\r\n$GNGSA,A,3,14,28,30,07,,,,,,,,,3.08,2.17,2.19,1*0F\r\n$GNGSA,A,3,79,88,81,,,,,,,,,,3.08,2.17,2.19,2*00\r\n$GNGSA,A,3,,,,,,,,,,,,,3.08,2.17,2.19,3*06\r\n$GNGSA,A,3,,,,,,,,,,,,,3.08,2.17,2.19,4*01\r\n$GPGSV,2,1,06,07,18,202,19,14,56,312,33,19,08,276,07,28,46,315,28,1*60\r\n$GPGSV,2,2,06,30,33,243,34,41,27,238,31,1*68\r\n$GPGSV,1,1,02,14,56,312,17,30,33,243,22,6*67\r\n$GPGSV,1,1,01,08,29,078,,0*58\r\n$GLGSV,1,1,03,79,22,328,32,81,26,263,32,88,61,327,31,1*45\r\n$GLGSV,2,1,05,65,10,116,15,78,65,278,26,79,22,328,25,81,26,263,19,3*7B\r\n$GLGSV,2,2,05,88,61,327,19,3*46\r\n$GLGSV,1,1,04,71,06,028,,72,16,073,,77,37,182,,87,40,030,,0*76\r\n$GAGSV,1,1,00,0*74\r\n$GBGSV,1,1,00,0*77\r\n$GNGLL,3717.4851570,N,12708.8858852,E,065659.00,A,A*78\r\n$GNRMC,065700.00,A,3717.4852951,N,12708.8854008,E,0.452,,190421,,,A,V*1D\r\n$GNVTG,,T,,M,0.452,N,0.837,K,A*32\r\n$GNGGA,065700.00,3717.4852951,N,12708.8854008,E,1,06,2.17,168.776,M,18.960,M,,*4A\r\n$GNGSA,A,3,14,28,30,07,,,,,,,,,3.08,2.17,2.19,1*0F\r\n$GNGSA,A,3,79,88,81,,,,,,,,,,3.08,2.17,2.19,2*00\r\n$GNGSA,A,3,,,,,,,,,,,,,3.08,2.17,2.19,3*06\r\n$GNGSA,A,3,,,,,,,,,,,,,3.08,2.17,2.19,4*01\r\n$GPGSV,2,1,06,07,18,202,20,14,56,312,33,19,08,276,10,28,46,315,28,1*6C\r\n$GPGSV,2,2,06,30,33,243,34,41,27,238,31,1*68\r\n$GPGSV,1,1,02,14,56,312,18,30,33,243,23,6*69\r\n$GPGSV,1,1,01,08,29,078,,0*58\r\n$GLGSV,1,1,02,79,22,328,32,81,26,263,32,1*77\r\n$GLGSV,2,1,05,65,10,116,14,78,65,278,27,79,22,328,24,81,26,263,19,3*7A\r\n$GLGSV,2,2,05,88,61,327,19,3*46\r\n$GLGSV,1,1,04,71,06,028,,72,16,073,,77,37,182,,87,40,030,,0*76\r\n$GAGSV,1,1,00,0*74\r\n$GBGSV,1,1,00,0*77\r\n$GNGLL,3717.4852951,N,12708.8854008,E,065700.00,A,A*72\r\n$GNRMC,065701.00,A,3717.4853526,N,12708.8851981,E,0.524,,190421,,,A,V*1C\r\n$GNVTG,,T,,M,0.524,N,0.971,K,A*31\r\n$GNGGA,065701.00,3717.4853526,N,12708.8851981,E,1,06,2.17,169.007,M,18.960,M,,*4B\r\n$GNGSA,A,3,14,28,30,07,,,,,,,,,3.08,2.17,2.19,1*0F\r\n$GNGSA,A,3,79,88,81,,,,,,,,,,3.08,2.17,2.19,2*00\r\n$GNGSA,A,3,,,,,,,,,,,,,3.08,2.17,2.19,3*06\r\n$GNGSA,A,3,,,,,,,,,,,,,3.08,2.17,2.19,4*01\r\n$GPGSV,2,1,06,07,18,202,21,14,56,312,33,19,08,276,07,28,46,315,27,1*64\r\n$GPGSV,2,2,06,30,33,243,34,41,27,238,31,1*68\r\n$GPGSV,1,1,02,14,56,312,18,30,33,243,24,6*6E\r\n$GPGSV,1,1,01,08,29,078,,0*58\r\n$GLGSV,1,1,02,79,22,328,32,81,26,263,32,1*77\r\n$GLGSV,2,1,05,65,10,116,13,78,65,278,26,79,22,328,24,81,26,263,20,3*76\r\n$GLGSV,2,2,05,88,61,327,19,3*46\r\n$GLGSV,1,1,04,71,06,028,,72,16,073,,77,37,182,,87,40,030,,0*76\r\n$GAGSV,1,1,00,0*74\r\n$GBGSV,1,1,00,0*77\r\n$GNGLL,3717.4853526,N,12708.8851981,E,065701.00,A,A*73\r\n$GNRMC,065702.00,A,3717.4853829,N,12708.8850834,E,0.558,,190421,,,A,V*18\r\n$GNVTG,,T,,M,0.558,N,1.034,K,A*33\r\n$GNGGA,065702.00,3717.4853829,N,12708.8850834,E,1,06,2.17,169.144,M,18.960,M,,*42\r\n$GNGSA,A,3,14,28,30,07,,,,,,,,,3.08,2.17,2.19,1*0F\r\n$GNGSA,A,3,79,88,81,,,,,,,,,,3.08,2.17,2.19,2*00\r\n$GNGSA,A,3,,,,,,,,,,,,,3.08,2.17,2.19,3*06\r\n$GNGSA,A,3,,,,,,,,,,,,,3.08,2.17,2.19,4*01\r\n$GPGSV,2,1,06,07,18,202,22,14,56,312,32,19,08,276,10,28,46,315,27,1*60\r\n$GPGSV,2,2,06,30,33,243,34,41,27,238,31,1*68\r\n$GPGSV,1,1,02,14,56,312,19,30,33,243,24,6*6F\r\n$GPGSV,1,1,01,08,29,078,,0*58\r\n$GLGSV,1,1,02,79,22,328,32,81,26,263,32,1*77\r\n$GLGSV,2,1,05,65,10,116,14,78,65,278,26,79,22,328,25,81,26,263,20,3*70\r\n$GLGSV,2,2,05,88,61,327,20,3*4C\r\n$GLGSV,1,1,04,71,06,028,,72,16,073,,77,37,182,,87,40,030,,0*76\r\n$GAGSV,1,1,00,0*74\r\n$GBGSV,1,1,00,0*77\r\n$GNGLL,3717.4853829,N,12708.8850834,E,065702.00,A,A*7C\r\n$GNRMC,065703.00,A,3717.4854881,N,12708.8846610,E,0.505,,190421,,,A,V*1B\r\n$GNVTG,,T,,M,0.505,N,0.934,K,A*33\r\n$GNGGA,065703.00,3717.4854881,N,12708.8846610,E,1,07,2.17,169.484,M,18.960,M,,*41\r\n$GNGSA,A,3,14,28,30,07,,,,,,,,,3.08,2.17,2.19,1*0F\r\n$GNGSA,A,3,79,88,81,,,,,,,,,,3.08,2.17,2.19,2*00\r\n$GNGSA,A,3,,,,,,,,,,,,,3.08,2.17,2.19,3*06\r\n$GNGSA,A,3,,,,,,,,,,,,,3.08,2.17,2.19,4*01\r\n$GPGSV,2,1,06,07,18,202,22,14,56,312,32,19,08,276,12,28,47,315,26,1*62\r\n$GPGSV,2,2,06,30,33,243,34,41,27,238,31,1*68\r\n$GPGSV,1,1,02,14,56,312,17,30,33,243,24,6*61\r\n$GPGSV,1,1,01,08,29,078,,0*58\r\n$GLGSV,1,1,02,79,22,328,32,81,26,263,32,1*77\r\n$GLGSV,1,1,04,65,10,116,15,78,65,278,26,81,26,263,20,88,61,327,20,3*70\r\n$GLGSV,1,1,04,71,06,028,,72,16,073,,77,37,182,,87,40,030,,0*76\r\n$GAGSV,1,1,00,0*74\r\n$GBGSV,1,1,00,0*77\r\n$GNGLL,3717.4854881,N,12708.8846610,E,065703.00,A,A*77\r\n$GNRMC,065704.00,A,3717.4856889,N,12708.8839112,E,0.400,,190421,,,A,V*1F\r\n$GNVTG,,T,,M,0.400,N,0.741,K,A*3B\r\n$GNGGA,065704.00,3717.4856889,N,12708.8839112,E,1,06,2.17,170.032,M,18.960,M,,*41\r\n$GNGSA,A,3,14,28,30,07,,,,,,,,,3.08,2.17,2.19,1*0F\r\n$GNGSA,A,3,79,88,81,,,,,,,,,,3.08,2.17,2.19,2*00\r\n$GNGSA,A,3,,,,,,,,,,,,,3.08,2.17,2.19,3*06\r\n$GNGSA,A,3,,,,,,,,,,,,,3.08,2.17,2.19,4*01\r\n$GPGSV,2,1,06,07,18,202,21,14,56,312,32,19,08,276,07,28,47,315,26,1*65\r\n$GPGSV,2,2,06,30,33,243,34,41,27,238,30,1*69\r\n$GPGSV,1,1,02,14,56,312,17,30,33,243,23,6*66\r\n$GPGSV,1,1,01,08,29,078,,0*58\r\n$GLGSV,1,1,02,79,22,328,32,81,26,263,32,1*77\r\n$GLGSV,2,1,05,65,10,116,15,78,65,278,26,79,22,328,25,81,26,263,20,3*71\r\n$GLGSV,2,2,05,88,61,327,20,3*4C\r\n$GLGSV,1,1,04,71,06,028,,72,16,073,,77,37,182,,87,40,030,,0*76\r\n$GAGSV,1,1,00,0*74\r\n$GBGSV,1,1,00,0*77\r\n$GNGLL,3717.4856889,N,12708.8839112,E,065704.00,A,A*77\r\n$GNRMC,065705.00,A,3717.4858338,N,12708.8834322,E,0.317,,190421,,,A,V*1C\r\n$GNVTG,,T,,M,0.317,N,0.588,K,A*3D\r\n$GNGGA,065705.00,3717.4858338,N,12708.8834322,E,1,06,2.17,170.264,M,18.960,M,,*42\r\n$GNGSA,A,3,14,28,30,07,,,,,,,,,3.08,2.17,2.20,1*05\r\n$GNGSA,A,3,79,88,81,,,,,,,,,,3.08,2.17,2.20,2*0A\r\n$GNGSA,A,3,,,,,,,,,,,,,3.08,2.17,2.20,3*0C\r\n$GNGSA,A,3,,,,,,,,,,,,,3.08,2.17,2.20,4*0B\r\n$GPGSV,2,1,06,07,18,202,21,14,56,312,33,19,08,276,10,28,47,315,26,1*62\r\n$GPGSV,2,2,06,30,33,243,34,41,27,238,31,1*68\r\n$GPGSV,1,1,02,14,56,312,17,30,33,243,23,6*66\r\n$GPGSV,1,1,01,08,29,078,,0*58\r\n$GLGSV,1,1,02,79,22,328,33,81,26,263,32,1*76\r\n$GLGSV,2,1,05,65,10,116,16,78,65,278,27,79,22,328,25,81,26,263,20,3*73\r\n$GLGSV,2,2,05,88,61,327,20,3*4C\r\n$GLGSV,1,1,04,71,06,028,,72,16,073,,77,37,182,,87,40,030,,0*76\r\n$GAGSV,1,1,00,0*74\r\n$GBGSV,1,1,00,0*77\r\n$GNGLL,3717.4858338,N,12708.8834322,E,065705.00,A,A*75\r\n$GNRMC,065706.00,A,3717.4860015,N,12708.8828779,E,0.275,,190421,,,A,V*1A\r\n$GNVTG,,T,,M,0.275,N,0.510,K,A*39\r\n$GNGGA,065706.00,3717.4860015,N,12708.8828779,E,1,06,2.17,170.758,M,18.960,M,,*4B\r\n$GNGSA,A,3,14,28,30,07,,,,,,,,,3.08,2.17,2.20,1*05\r\n$GNGSA,A,3,79,88,81,,,,,,,,,,3.08,2.17,2.20,2*0A\r\n$GNGSA,A,3,,,,,,,,,,,,,3.08,2.17,2.20,3*0C\r\n$GNGSA,A,3,,,,,,,,,,,,,3.08,2.17,2.20,4*0B\r\n$GPGSV,2,1,06,07,18,202,22,14,56,312,33,19,08,276,14,28,47,315,26,1*65\r\n$GPGSV,2,2,06,30,33,243,34,41,27,238,31,1*68\r\n$GPGSV,1,1,02,14,56,312,17,30,33,243,23,6*66\r\n$GPGSV,1,1,01,08,29,078,,0*58\r\n$GLGSV,1,1,02,79,22,328,33,81,26,263,33,1*77\r\n$GLGSV,2,1,05,65,10,116,16,78,65,278,27,79,22,328,25,81,26,263,20,3*73\r\n$GLGSV,2,2,05,88,61,327,20,3*4C\r\n$GLGSV,1,1,04,71,06,028,,72,16,073,,77,37,182,,87,40,030,,0*76\r\n$GAGSV,1,1,00,0*74\r\n$GBGSV,1,1,00,0*77\r\n$GNGLL,3717.4860015,N,12708.8828779,E,065706.00,A,A*76\r\n$GNRMC,065707.00,A,3717.4860666,N,12708.8827875,E,0.349,,190421,,,A,V*1B\r\n$GNVTG,,T,,M,0.349,N,0.647,K,A*36\r\n$GNGGA,065707.00,3717.4860666,N,12708.8827875,E,1,06,2.17,171.108,M,18.960,M,,*46\r\n$GNGSA,A,3,14,28,30,07,,,,,,,,,3.08,2.17,2.20,1*05\r\n$GNGSA,A,3,79,88,81,,,,,,,,,,3.08,2.17,2.20,2*0A\r\n$GNGSA,A,3,,,,,,,,,,,,,3.08,2.17,2.20,3*0C\r\n$GNGSA,A,3,,,,,,,,,,,,,3.08,2.17,2.20,4*0B\r\n$GPGSV,2,1,06,07,18,202,22,14,56,312,32,19,08,276,10,28,47,315,26,1*60\r\n$GPGSV,2,2,06,30,33,243,34,41,27,238,30,1*69\r\n$GPGSV,1,1,02,14,56,312,17,30,33,243,23,6*66\r\n$GPGSV,1,1,01,08,29,078,,0*58\r\n$GLGSV,1,1,02,79,22,328,34,81,26,263,34,1*77\r\n$GLGSV,2,1,05,65,10,116,17,78,65,278,27,79,22,328,26,81,26,263,20,3*71\r\n$GLGSV,2,2,05,88,61,327,19,3*46\r\n$GLGSV,1,1,04,71,06,028,,72,16,073,,77,37,182,,87,40,030,,0*76\r\n$GAGSV,1,1,00,0*74\r\n$GBGSV,1,1,00,0*77\r\n$GNGLL,3717.4860666,N,12708.8827875,E,065707.00,A,A*79\r\n$GNRMC,065708.00,A,3717.4862333,N,12708.8823237,E,0.268,,190421,,,A,V*19\r\n$GNVTG,,T,,M,0.268,N,0.496,K,A*3A\r\n$GNGGA,065708.00,3717.4862333,N,12708.8823237,E,1,06,2.17,171.619,M,18.960,M,,*41\r\n$GNGSA,A,3,14,28,30,07,,,,,,,,,3.08,2.17,2.20,1*05\r\n$GNGSA,A,3,79,88,81,,,,,,,,,,3.08,2.17,2.20,2*0A\r\n$GNGSA,A,3,,,,,,,,,,,,,3.08,2.17,2.20,3*0C\r\n$GNGSA,A,3,,,,,,,,,,,,,3.08,2.17,2.20,4*0B\r\n$GPGSV,2,1,06,07,18,202,22,14,56,312,33,19,08,276,09,28,47,315,25,1*6A\r\n$GPGSV,2,2,06,30,33,243,33,41,27,238,30,1*6E\r\n$GPGSV,1,1,02,14,56,312,18,30,33,243,24,6*6E\r\n$GPGSV,1,1,01,08,29,078,,0*58\r\n$GLGSV,1,1,02,79,22,328,34,81,26,263,34,1*77\r\n$GLGSV,2,1,05,65,10,116,15,78,65,278,27,79,22,328,25,81,26,263,20,3*70\r\n$GLGSV,2,2,05,88,61,327,19,3*46\r\n$GLGSV,1,1,04,71,06,028,,72,16,073,,77,37,182,,87,40,030,,0*76\r\n$GAGSV,1,1,00,0*74\r\n$GBGSV,1,1,00,0*77\r\n$GNGLL,3717.4862333,N,12708.8823237,E,065708.00,A,A*79\r\n$GNRMC,065709.00,A,3717.4863757,N,12708.8819239,E,0.329,,190421,,,A,V*1C\r\n$GNVTG,,T,,M,0.329,N,0.610,K,A*32\r\n$GNGGA,065709.00,3717.4863757,N,12708.8819239,E,1,06,2.17,172.107,M,18.960,M,,*4B\r\n$GNGSA,A,3,14,28,30,07,,,,,,,,,3.08,2.17,2.20,1*05\r\n$GNGSA,A,3,79,88,81,,,,,,,,,,3.08,2.17,2.20,2*0A\r\n$GNGSA,A,3,,,,,,,,,,,,,3.08,2.17,2.20,3*0C\r\n$GNGSA,A,3,,,,,,,,,,,,,3.08,2.17,2.20,4*0B\r\n$GPGSV,2,1,06,07,18,202,22,14,56,312,33,19,08,276,09,28,47,315,25,1*6A\r\n$GPGSV,2,2,06,30,33,243,33,41,27,238,30,1*6E\r\n$GPGSV,1,1,02,14,56,312,18,30,33,243,24,6*6E\r\n$GPGSV,1,1,01,08,29,078,,0*58\r\n$GLGSV,1,1,02,79,22,328,34,81,26,263,33,1*70\r\n$GLGSV,2,1,05,65,10,116,14,78,65,278,27,79,22,328,24,81,26,263,20,3*70\r\n$GLGSV,2,2,05,88,61,327,19,3*46\r\n$GLGSV,1,1,04,71,06,028,,72,16,073,,77,37,182,,87,40,030,,0*76\r\n$GAGSV,1,1,00,0*74\r\n$GBGSV,1,1,00,0*77\r\n$GNGLL,3717.4863757,N,12708.8819239,E,065709.00,A,A*78\r\n$GNRMC,065710.00,A,3717.4865150,N,12708.8815085,E,0.407,,190421,,,A,V*11\r\n$GNVTG,,T,,M,0.407,N,0.754,K,A*38\r\n$GNGGA,065710.00,3717.4865150,N,12708.8815085,E,1,06,2.17,172.508,M,18.960,M,,*46\r\n$GNGSA,A,3,14,28,30,07,,,,,,,,,3.08,2.17,2.20,1*05\r\n$GNGSA,A,3,79,88,81,,,,,,,,,,3.08,2.17,2.20,2*0A\r\n$GNGSA,A,3,,,,,,,,,,,,,3.08,2.17,2.20,3*0C\r\n$GNGSA,A,3,,,,,,,,,,,,,3.08,2.17,2.20,4*0B\r\n$GPGSV,2,1,06,07,18,202,23,14,56,312,33,19,08,276,09,28,47,315,25,1*6B\r\n$GPGSV,2,2,06,30,33,243,33,41,27,238,30,1*6E\r\n$GPGSV,1,1,02,14,56,312,18,30,33,243,25,6*6F\r\n$GPGSV,1,1,01,08,29,078,,0*58\r\n$GLGSV,1,1,02,79,22,328,35,81,26,263,33,1*71\r\n$GLGSV,2,1,05,65,10,116,14,78,65,278,27,79,22,328,24,81,26,263,20,3*70\r\n$GLGSV,2,2,05,88,61,327,20,3*4C\r\n$GLGSV,1,1,04,71,06,028,,72,16,073,,77,37,182,,87,40,030,,0*76\r\n$GAGSV,1,1,00,0*74\r\n$GBGSV,1,1,00,0*77\r\n$GNGLL,3717.4865150,N,12708.8815085,E,065710.00,A,A*7E\r\n$GNRMC,065711.00,A,3717.4866832,N,12708.8810433,E,0.275,,190421,,,A,V*11\r\n$GNVTG,,T,,M,0.275,N,0.510,K,A*39\r\n$GNGGA,065711.00,3717.4866832,N,12708.8810433,E,1,07,2.17,172.904,M,18.960,M,,*44\r\n$GNGSA,A,3,14,28,30,07,,,,,,,,,3.08,2.17,2.20,1*05\r\n$GNGSA,A,3,79,88,81,,,,,,,,,,3.08,2.17,2.20,2*0A\r\n$GNGSA,A,3,,,,,,,,,,,,,3.08,2.17,2.20,3*0C\r\n$GNGSA,A,3,,,,,,,,,,,,,3.08,2.17,2.20,4*0B\r\n$GPGSV,2,1,06,07,18,202,23,14,56,312,33,19,08,276,09,28,47,315,26,1*68\r\n$GPGSV,2,2,06,30,33,243,34,41,27,238,30,1*69\r\n$GPGSV,1,1,02,14,56,312,18,30,33,243,24,6*6E\r\n$GPGSV,1,1,01,08,29,078,,0*58\r\n$GLGSV,1,1,02,79,22,328,35,81,26,263,33,1*71\r\n$GLGSV,2,1,05,65,10,116,14,78,65,278,27,79,22,328,23,81,26,263,21,3*76\r\n$GLGSV,2,2,05,88,61,327,20,3*4C\r\n$GLGSV,1,1,04,71,06,028,,72,16,073,,77,37,182,,87,40,030,,0*76\r\n$GAGSV,1,1,00,0*74\r\n$GBGSV,1,1,00,0*77\r\n$GNGLL,3717.4866832,N,12708.8810433,E,065711.00,A,A*7D\r\n$GNRMC,065712.00,A,3717.4868271,N,12708.8804965,E,0.267,,190421,,,A,V*19\r\n$GNVTG,,T,,M,0.267,N,0.494,K,A*37\r\n$GNGGA,065712.00,3717.4868271,N,12708.8804965,E,1,07,2.17,173.458,M,18.960,M,,*4A\r\n$GNGSA,A,3,14,28,30,07,,,,,,,,,3.08,2.17,2.20,1*05\r\n$GNGSA,A,3,79,88,81,,,,,,,,,,3.08,2.17,2.20,2*0A\r\n$GNGSA,A,3,,,,,,,,,,,,,3.08,2.17,2.20,3*0C\r\n$GNGSA,A,3,,,,,,,,,,,,,3.08,2.17,2.20,4*0B\r\n$GPGSV,2,1,06,07,18,202,23,14,56,312,33,19,08,276,06,28,47,315,26,1*67\r\n$GPGSV,2,2,06,30,33,243,34,41,27,238,30,1*69\r\n$GPGSV,1,1,02,14,56,312,19,30,33,243,24,6*6F\r\n$GPGSV,1,1,01,08,29,078,,0*58\r\n$GLGSV,1,1,02,79,22,328,35,81,26,263,33,1*71\r\n$GLGSV,2,1,05,65,10,116,15,78,65,278,27,79,22,328,24,81,26,263,21,3*70\r\n$GLGSV,2,2,05,88,61,327,20,3*4C\r\n$GLGSV,1,1,04,71,06,028,,72,16,073,,77,37,182,,87,40,030,,0*76\r\n$GAGSV,1,1,00,0*74\r\n$GBGSV,1,1,00,0*77\r\n$GNGLL,3717.4868271,N,12708.8804965,E,065712.00,A,A*76\r\n$GNRMC,065713.00,A,3717.4870424,N,12708.8797058,E,0.178,,190421,,,A,V*18\r\n$GNVTG,,T,,M,0.178,N,0.329,K,A*3B\r\n$GNGGA,065713.00,3717.4870424,N,12708.8797058,E,1,06,2.17,174.045,M,18.960,M,,*48\r\n$GNGSA,A,3,14,28,30,07,,,,,,,,,3.09,2.17,2.20,1*04\r\n$GNGSA,A,3,79,88,81,,,,,,,,,,3.09,2.17,2.20,2*0B\r\n$GNGSA,A,3,,,,,,,,,,,,,3.09,2.17,2.20,3*0D\r\n$GNGSA,A,3,,,,,,,,,,,,,3.09,2.17,2.20,4*0A\r\n$GPGSV,2,1,06,07,18,202,23,14,56,312,33,19,08,276,07,28,47,315,26,1*66\r\n$GPGSV,2,2,06,30,33,243,33,41,27,238,30,1*6E\r\n$GPGSV,1,1,02,14,56,312,19,30,33,243,24,6*6F\r\n$GPGSV,1,1,01,08,29,078,,0*58\r\n$GLGSV,1,1,02,79,22,328,35,81,26,263,32,1*70\r\n$GLGSV,2,1,05,65,10,116,13,78,65,278,27,79,22,328,24,81,26,263,20,3*77\r\n$GLGSV,2,2,05,88,61,327,20,3*4C\r\n$GLGSV,1,1,04,71,06,028,,72,16,073,,77,37,182,,87,40,030,,0*76\r\n$GAGSV,1,1,00,0*74\r\n$GBGSV,1,1,00,0*77\r\n$GNGLL,3717.4870424,N,12708.8797058,E,065713.00,A,A*7A\r\n$GNRMC,065714.00,A,3717.4872135,N,12708.8789015,E,0.201,,190421,,,A,V*13\r\n$GNVTG,,T,,M,0.201,N,0.373,K,A*39\r\n$GNGGA,065714.00,3717.4872135,N,12708.8789015,E,1,07,2.17,174.597,M,18.960,M,,*45\r\n$GNGSA,A,3,14,28,30,07,,,,,,,,,3.09,2.17,2.20,1*04\r\n$GNGSA,A,3,79,88,81,,,,,,,,,,3.09,2.17,2.20,2*0B\r\n$GNGSA,A,3,,,,,,,,,,,,,3.09,2.17,2.20,3*0D\r\n$GNGSA,A,3,,,,,,,,,,,,,3.09,2.17,2.20,4*0A\r\n$GPGSV,2,1,06,07,18,202,23,14,56,312,33,19,08,276,09,28,47,315,26,1*68\r\n$GPGSV,2,2,06,30,33,243,33,41,27,238,31,1*6F\r\n$GPGSV,1,1,02,14,56,312,19,30,33,243,24,6*6F\r\n$GPGSV,1,1,01,08,29,078,,0*58\r\n$GLGSV,1,1,02,79,22,328,35,81,26,263,33,1*71\r\n$GLGSV,2,1,05,65,10,116,14,78,65,278,27,79,22,328,23,81,26,263,20,3*77\r\n$GLGSV,2,2,05,88,61,327,19,3*46\r\n$GLGSV,1,1,04,71,06,028,,72,16,073,,77,37,182,,87,40,030,,0*76\r\n$GAGSV,1,1,00,0*74\r\n$GBGSV,1,1,00,0*77\r\n$GNGLL,3717.4872135,N,12708.8789015,E,065714.00,A,A*7C\r\n$GNRMC,065715.00,A,3717.4873872,N,12708.8781837,E,0.108,,190421,,,A,V*13\r\n$GNVTG,,T,,M,0.108,N,0.201,K,A*37\r\n$GNGGA,065715.00,3717.4873872,N,12708.8781837,E,1,06,2.17,175.002,M,18.960,M,,*46\r\n$GNGSA,A,3,14,28,30,07,,,,,,,,,3.09,2.17,2.20,1*04\r\n$GNGSA,A,3,79,88,81,,,,,,,,,,3.09,2.17,2.20,2*0B\r\n$GNGSA,A,3,,,,,,,,,,,,,3.09,2.17,2.20,3*0D\r\n$GNGSA,A,3,,,,,,,,,,,,,3.09,2.17,2.20,4*0A\r\n$GPGSV,2,1,06,07,18,202,23,14,56,312,33,19,08,276,09,28,47,315,26,1*68\r\n$GPGSV,2,2,06,30,33,243,33,41,27,238,30,1*6E\r\n$GPGSV,1,1,02,14,56,312,18,30,33,243,25,6*6F\r\n$GPGSV,1,1,01,08,29,078,,0*58\r\n$GLGSV,1,1,02,79,22,328,35,81,26,263,32,1*70\r\n$GLGSV,2,1,05,65,10,116,13,78,65,278,28,79,22,328,23,81,26,263,20,3*7F\r\n$GLGSV,2,2,05,88,61,327,20,3*4C\r\n$GLGSV,1,1,04,71,06,028,,72,16,073,,77,37,182,,87,40,030,,0*76\r\n$GAGSV,1,1,00,0*74\r\n$GBGSV,1,1,00,0*77\r\n$GNGLL,3717.4873872,N,12708.8781837,E,065715.00,A,A*76\r\n$GNRMC,065716.00,A,3717.4876847,N,12708.8770018,E,0.192,,190421,,,A,V*1B\r\n$GNVTG,,T,,M,0.192,N,0.356,K,A*37\r\n$GNGGA,065716.00,3717.4876847,N,12708.8770018,E,1,06,2.16,175.683,M,18.960,M,,*43\r\n$GNGSA,A,3,14,28,30,07,,,,,,,,,3.09,2.16,2.20,1*05\r\n$GNGSA,A,3,79,88,81,,,,,,,,,,3.09,2.16,2.20,2*0A\r\n$GNGSA,A,3,,,,,,,,,,,,,3.09,2.16,2.20,3*0C\r\n$GNGSA,A,3,,,,,,,,,,,,,3.09,2.16,2.20,4*0B\r\n$GPGSV,2,1,06,07,18,202,22,14,56,312,32,19,08,276,09,28,47,315,26,1*68\r\n$GPGSV,2,2,06,30,33,243,32,41,27,238,30,1*6F\r\n$GPGSV,1,1,02,14,56,312,18,30,33,243,24,6*6E\r\n$GPGSV,1,1,01,08,29,078,,0*58\r\n$GLGSV,1,1,02,79,22,328,35,81,26,263,31,1*73\r\n$GLGSV,2,1,05,65,10,116,14,78,65,278,27,79,22,328,23,81,26,263,18,3*7C\r\n$GLGSV,2,2,05,88,61,327,19,3*46\r\n$GLGSV,1,1,04,71,06,028,,72,16,073,,77,37,182,,87,40,030,,0*76\r\n$GAGSV,1,1,00,0*74\r\n$GBGSV,1,1,00,0*77\r\n$GNGLL,3717.4876847,N,12708.8770018,E,065716.00,A,A*7D\r\n$GNRMC,065717.00,A,3717.4878496,N,12708.8763959,E,0.070,,190421,,,A,V*17\r\n$GNVTG,,T,,M,0.070,N,0.130,K,A*38\r\n$GNGGA,065717.00,3717.4878496,N,12708.8763959,E,1,06,2.16,176.159,M,18.960,M,,*41\r\n$GNGSA,A,3,14,28,30,07,,,,,,,,,3.09,2.16,2.20,1*05\r\n$GNGSA,A,3,79,88,81,,,,,,,,,,3.09,2.16,2.20,2*0A\r\n$GNGSA,A,3,,,,,,,,,,,,,3.09,2.16,2.20,3*0C\r\n$GNGSA,A,3,,,,,,,,,,,,,3.09,2.16,2.20,4*0B\r\n$GPGSV,2,1,06,07,18,202,23,14,56,312,32,19,08,276,08,28,47,315,26,1*68\r\n$GPGSV,2,2,06,30,33,243,32,41,27,238,30,1*6F\r\n$GPGSV,1,1,02,14,56,312,18,30,33,243,24,6*6E\r\n$GPGSV,1,1,01,08,29,078,,0*58\r\n$GLGSV,1,1,02,79,22,328,34,81,26,263,31,1*72\r\n$GLGSV,2,1,06,65,10,116,15,77,37,182,17,78,65,278,27,79,22,328,24,3*73\r\n$GLGSV,2,2,06,81,26,263,18,88,61,327,19,3*76\r\n$GLGSV,1,1,03,71,06,028,,72,16,073,,87,40,030,,0*4E\r\n$GAGSV,1,1,00,0*74\r\n$GBGSV,1,1,00,0*77\r\n$GNGLL,3717.4878496,N,12708.8763959,E,065717.00,A,A*7C\r\n$GNRMC,065718.00,A,3717.4879906,N,12708.8759141,E,0.129,,190421,,,A,V*18\r\n$GNVTG,,T,,M,0.129,N,0.238,K,A*3E\r\n$GNGGA,065718.00,3717.4879906,N,12708.8759141,E,1,06,2.16,176.529,M,18.960,M,,*40\r\n$GNGSA,A,3,14,28,30,07,,,,,,,,,3.09,2.16,2.20,1*05\r\n$GNGSA,A,3,79,88,81,,,,,,,,,,3.09,2.16,2.20,2*0A\r\n$GNGSA,A,3,,,,,,,,,,,,,3.09,2.16,2.20,3*0C\r\n$GNGSA,A,3,,,,,,,,,,,,,3.09,2.16,2.20,4*0B\r\n$GPGSV,2,1,06,07,18,202,23,14,56,312,32,19,08,276,08,28,47,315,26,1*68\r\n$GPGSV,2,2,06,30,33,243,32,41,27,238,30,1*6F\r\n$GPGSV,1,1,02,14,56,312,18,30,33,243,24,6*6E\r\n$GPGSV,1,1,01,08,29,078,,0*58\r\n$GLGSV,1,1,02,79,22,328,34,81,26,263,31,1*72\r\n$GLGSV,2,1,06,65,10,116,15,77,37,182,17,78,65,278,27,79,22,328,24,3*73\r\n$GLGSV,2,2,06,81,26,263,17,88,61,327,18,3*78\r\n$GLGSV,1,1,03,71,06,028,,72,16,073,,87,40,030,,0*4E\r\n$GAGSV,1,1,00,0*74\r\n$GBGSV,1,1,00,0*77\r\n$GNGLL,3717.4879906,N,12708.8759141,E,065718.00,A,A*7E\r\n$GNRMC,065719.00,A,3717.4881737,N,12708.8752426,E,0.096,,190421,,,A,V*18\r\n$GNVTG,,T,,M,0.096,N,0.177,K,A*33\r\n$GNGGA,065719.00,3717.4881737,N,12708.8752426,E,1,06,2.16,177.068,M,18.960,M,,*44\r\n$GNGSA,A,3,14,28,30,07,,,,,,,,,3.09,2.16,2.20,1*05\r\n$GNGSA,A,3,79,88,81,,,,,,,,,,3.09,2.16,2.20,2*0A\r\n$GNGSA,A,3,,,,,,,,,,,,,3.09,2.16,2.20,3*0C\r\n$GNGSA,A,3,,,,,,,,,,,,,3.09,2.16,2.20,4*0B\r\n$GPGSV,2,1,06,07,18,202,24,14,56,312,32,19,08,276,09,28,47,315,26,1*6E\r\n$GPGSV,2,2,06,30,33,243,32,41,27,238,30,1*6F\r\n$GPGSV,1,1,02,14,56,312,18,30,33,243,25,6*6F\r\n$GPGSV,1,1,01,08,29,078,,0*58\r\n$GLGSV,1,1,02,79,22,328,34,81,26,263,30,1*73\r\n$GLGSV,2,1,06,65,10,116,15,77,37,182,18,78,65,278,27,79,22,328,23,3*7B\r\n$GLGSV,2,2,06,81,26,263,17,88,61,327,18,3*78\r\n$GLGSV,1,1,03,71,06,028,,72,16,073,,87,40,030,,0*4E\r\n$GAGSV,1,1,00,0*74\r\n$GBGSV,1,1,00,0*77\r\n$GNGLL,3717.4881737,N,12708.8752426,E,065719.00,A,A*7B\r\n$GNRMC,065720.00,A,3717.4883243,N,12708.8746269,E,0.129,,190421,,,A,V*1B\r\n$GNVTG,,T,,M,0.129,N,0.239,K,A*3F\r\n$GNGGA,065720.00,3717.4883243,N,12708.8746269,E,1,06,2.16,177.577,M,18.960,M,,*49\r\n$GNGSA,A,3,14,28,30,07,,,,,,,,,3.09,2.16,2.20,1*05\r\n$GNGSA,A,3,79,88,81,,,,,,,,,,3.09,2.16,2.20,2*0A\r\n$GNGSA,A,3,,,,,,,,,,,,,3.09,2.16,2.20,3*0C\r\n$GNGSA,A,3,,,,,,,,,,,,,3.09,2.16,2.20,4*0B\r\n$GPGSV,2,1,06,07,18,202,24,14,56,312,32,19,08,276,09,28,47,315,26,1*6E\r\n$GPGSV,2,2,06,30,33,243,32,41,27,238,30,1*6F\r\n$GPGSV,1,1,02,14,56,312,18,30,33,243,24,6*6E\r\n$GPGSV,1,1,01,08,29,078,,0*58\r\n$GLGSV,1,1,02,79,22,328,33,81,26,263,31,1*75\r\n$GLGSV,2,1,06,65,10,116,15,77,37,182,17,78,65,278,27,79,22,328,23,3*74\r\n$GLGSV,2,2,06,81,26,263,17,88,61,327,19,3*79\r\n$GLGSV,1,1,03,71,06,028,,72,16,073,,87,40,030,,0*4E\r\n$GAGSV,1,1,00,0*74\r\n$GBGSV,1,1,00,0*77\r\n$GNGLL,3717.4883243,N,12708.8746269,E,065720.00,A,A*7D\r\n$GNRMC,065721.00,A,3717.4885408,N,12708.8738499,E,0.160,,190421,,,A,V*18\r\n$GNVTG,,T,,M,0.160,N,0.297,K,A*36\r\n$GNGGA,065721.00,3717.4885408,N,12708.8738499,E,1,06,2.16,178.246,M,18.960,M,,*4D\r\n$GNGSA,A,3,14,28,30,07,,,,,,,,,3.09,2.16,2.20,1*05\r\n$GNGSA,A,3,79,88,81,,,,,,,,,,3.09,2.16,2.20,2*0A\r\n$GNGSA,A,3,,,,,,,,,,,,,3.09,2.16,2.20,3*0C\r\n$GNGSA,A,3,,,,,,,,,,,,,3.09,2.16,2.20,4*0B\r\n$GPGSV,2,1,06,07,18,202,24,14,56,312,32,19,08,276,10,28,47,315,26,1*66\r\n$GPGSV,2,2,06,30,33,243,32,41,27,238,30,1*6F\r\n$GPGSV,1,1,02,14,56,312,16,30,33,243,24,6*60\r\n$GPGSV,1,1,01,08,29,078,,0*58\r\n$GLGSV,1,1,02,79,22,328,33,81,26,263,31,1*75\r\n$GLGSV,2,1,06,65,10,116,14,77,37,182,18,78,65,278,27,79,22,328,23,3*7A\r\n$GLGSV,2,2,06,81,26,263,18,88,61,327,19,3*76\r\n$GLGSV,1,1,03,71,06,028,,72,16,073,,87,40,030,,0*4E\r\n$GAGSV,1,1,00,0*74\r\n$GBGSV,1,1,00,0*77\r\n$GNGLL,3717.4885408,N,12708.8738499,E,065721.00,A,A*73\r\n$GNRMC,065722.00,A,3717.4887536,N,12708.8730180,E,0.230,,190421,,,A,V*16\r\n$GNVTG,,T,,M,0.230,N,0.426,K,A*3C\r\n$GNGGA,065722.00,3717.4887536,N,12708.8730180,E,1,06,2.16,178.781,M,18.960,M,,*4B\r\n$GNGSA,A,3,14,28,30,07,,,,,,,,,3.09,2.16,2.20,1*05\r\n$GNGSA,A,3,79,88,81,,,,,,,,,,3.09,2.16,2.20,2*0A\r\n$GNGSA,A,3,,,,,,,,,,,,,3.09,2.16,2.20,3*0C\r\n$GNGSA,A,3,,,,,,,,,,,,,3.09,2.16,2.20,4*0B\r\n$GPGSV,2,1,06,07,18,202,24,14,56,312,32,19,08,276,07,28,47,315,26,1*60\r\n$GPGSV,2,2,06,30,33,243,32,41,27,238,30,1*6F\r\n$GPGSV,1,1,02,14,56,312,17,30,33,243,24,6*61\r\n$GPGSV,1,1,01,08,29,078,,0*58\r\n$GLGSV,1,1,03,78,65,278,26,79,22,328,33,81,26,263,30,1*40\r\n$GLGSV,2,1,06,65,10,116,14,77,37,182,18,78,65,278,27,79,22,328,23,3*7A\r\n$GLGSV,2,2,06,81,26,263,19,88,61,327,19,3*77\r\n$GLGSV,1,1,03,71,06,028,,72,16,073,,87,40,030,,0*4E\r\n$GAGSV,1,1,00,0*74\r\n$GBGSV,1,1,00,0*77\r\n$GNGLL,3717.4887536,N,12708.8730180,E,065722.00,A,A*7B\r\n$GNRMC,065723.00,A,3717.4889111,N,12708.8724385,E,0.109,,190421,,,A,V*13\r\n$GNVTG,,T,,M,0.109,N,0.201,K,A*36\r\n$GNGGA,065723.00,3717.4889111,N,12708.8724385,E,1,06,2.16,179.308,M,18.960,M,,*43\r\n$GNGSA,A,3,14,28,30,07,,,,,,,,,3.09,2.16,2.20,1*05\r\n$GNGSA,A,3,79,88,81,,,,,,,,,,3.09,2.16,2.20,2*0A\r\n$GNGSA,A,3,,,,,,,,,,,,,3.09,2.16,2.20,3*0C\r\n$GNGSA,A,3,,,,,,,,,,,,,3.09,2.16,2.20,4*0B\r\n$GPGSV,2,1,06,07,18,202,24,14,56,312,32,19,08,276,08,28,47,315,26,1*6F\r\n$GPGSV,2,2,06,30,33,243,32,41,27,238,29,1*67\r\n$GPGSV,1,1,02,14,56,312,17,30,33,243,24,6*61\r\n$GPGSV,1,1,01,08,29,078,,0*58\r\n$GLGSV,1,1,03,78,65,278,26,79,22,328,33,81,26,263,30,1*40\r\n$GLGSV,2,1,06,65,11,116,14,77,37,182,18,78,65,278,27,79,22,328,23,3*7B\r\n$GLGSV,2,2,06,81,26,263,19,88,61,327,18,3*76\r\n$GLGSV,1,1,03,71,06,028,,72,16,073,,87,40,030,,0*4E\r\n$GAGSV,1,1,00,0*74\r\n$GBGSV,1,1,00,0*77\r\n$GNGLL,3717.4889111,N,12708.8724385,E,065723.00,A,A*77\r\n$GNRMC,065724.00,A,3717.4891342,N,12708.8715530,E,0.229,,190421,,,A,V*12\r\n$GNVTG,,T,,M,0.229,N,0.425,K,A*37\r\n$GNGGA,065724.00,3717.4891342,N,12708.8715530,E,1,06,2.16,179.973,M,18.960,M,,*45\r\n$GNGSA,A,3,14,28,30,07,,,,,,,,,3.09,2.16,2.20,1*05\r\n$GNGSA,A,3,79,88,81,,,,,,,,,,3.09,2.16,2.20,2*0A\r\n$GNGSA,A,3,,,,,,,,,,,,,3.09,2.16,2.20,3*0C\r\n$GNGSA,A,3,,,,,,,,,,,,,3.09,2.16,2.20,4*0B\r\n$GPGSV,2,1,06,07,18,202,24,14,56,312,31,19,08,276,08,28,47,315,26,1*6C\r\n$GPGSV,2,2,06,30,33,243,32,41,27,238,30,1*6F\r\n$GPGSV,1,1,02,14,56,312,17,30,33,243,24,6*61\r\n$GPGSV,1,1,01,08,29,078,,0*58\r\n$GLGSV,1,1,03,78,65,278,26,79,22,328,33,81,26,263,30,1*40\r\n$GLGSV,2,1,06,65,11,116,14,77,37,182,18,78,65,278,27,79,22,328,24,3*7C\r\n$GLGSV,2,2,06,81,26,263,19,88,61,327,19,3*77\r\n$GLGSV,1,1,03,71,06,028,,72,16,073,,87,40,030,,0*4E\r\n$GAGSV,1,1,00,0*74\r\n$GBGSV,1,1,00,0*77\r\n$GNGLL,3717.4891342,N,12708.8715530,E,065724.00,A,A*77\r\n$GNRMC,065725.00,A,3717.4892639,N,12708.8710551,E,0.159,,190421,,,A,V*1F\r\n$GNVTG,,T,,M,0.159,N,0.294,K,A*3F\r\n$GNGGA,065725.00,3717.4892639,N,12708.8710551,E,1,06,2.16,180.439,M,18.960,M,,*49\r\n$GNGSA,A,3,14,28,30,07,,,,,,,,,3.09,2.16,2.20,1*05\r\n$GNGSA,A,3,79,88,81,,,,,,,,,,3.09,2.16,2.20,2*0A\r\n$GNGSA,A,3,,,,,,,,,,,,,3.09,2.16,2.20,3*0C\r\n$GNGSA,A,3,,,,,,,,,,,,,3.09,2.16,2.20,4*0B\r\n$GPGSV,2,1,06,07,18,202,25,14,56,312,31,19,08,276,07,28,47,315,26,1*62\r\n$GPGSV,2,2,06,30,33,243,32,41,27,238,29,1*67\r\n$GPGSV,1,1,02,14,56,312,18,30,33,243,24,6*6E\r\n$GPGSV,1,1,01,08,29,078,,0*58\r\n$GLGSV,1,1,03,78,65,278,27,79,22,328,33,81,26,263,31,1*40\r\n$GLGSV,2,1,06,65,11,116,13,77,37,182,19,78,65,278,27,79,22,328,24,3*7A\r\n$GLGSV,2,2,06,81,26,263,18,88,61,327,20,3*7C\r\n$GLGSV,1,1,03,71,06,028,,72,16,073,,87,40,030,,0*4E\r\n$GAGSV,1,1,00,0*74\r\n$GBGSV,1,1,00,0*77\r\n$GNGLL,3717.4892639,N,12708.8710551,E,065725.00,A,A*7E\r\n$GNRMC,065726.00,A,3717.4894044,N,12708.8704872,E,0.160,,190421,,,A,V*15\r\n$GNVTG,,T,,M,0.160,N,0.297,K,A*36\r\n$GNGGA,065726.00,3717.4894044,N,12708.8704872,E,1,06,2.16,180.972,M,18.960,M,,*4B\r\n$GNGSA,A,3,14,28,30,07,,,,,,,,,3.09,2.16,2.20,1*05\r\n$GNGSA,A,3,79,88,81,,,,,,,,,,3.09,2.16,2.20,2*0A\r\n$GNGSA,A,3,,,,,,,,,,,,,3.09,2.16,2.20,3*0C\r\n$GNGSA,A,3,,,,,,,,,,,,,3.09,2.16,2.20,4*0B\r\n$GPGSV,2,1,06,07,18,202,24,14,56,312,31,19,08,276,08,28,47,315,26,1*6C\r\n$GPGSV,2,2,06,30,33,243,31,41,27,238,29,1*64\r\n$GPGSV,1,1,02,14,56,312,18,30,33,243,25,6*6F\r\n$GPGSV,1,1,01,08,29,078,,0*58\r\n$GLGSV,1,1,03,78,65,278,28,79,22,328,33,81,26,263,30,1*4E\r\n$GLGSV,2,1,06,65,11,116,14,77,37,182,18,78,65,278,27,79,22,328,23,3*7B\r\n$GLGSV,2,2,06,81,26,263,18,88,61,327,20,3*7C\r\n$GLGSV,1,1,03,71,06,028,,72,16,073,,87,40,030,,0*4E\r\n$GAGSV,1,1,00,0*74\r\n$GBGSV,1,1,00,0*77\r\n$GNGLL,3717.4894044,N,12708.8704872,E,065726.00,A,A*7E\r\n$GNRMC,065727.00,A,3717.4895411,N,12708.8700356,E,0.231,,190421,,,A,V*1F\r\n$GNVTG,,T,,M,0.231,N,0.428,K,A*33\r\n$GNGGA,065727.00,3717.4895411,N,12708.8700356,E,1,07,2.16,181.425,M,18.960,M,,*49\r\n$GNGSA,A,3,14,28,30,07,,,,,,,,,3.09,2.16,2.20,1*05\r\n$GNGSA,A,3,79,88,81,,,,,,,,,,3.09,2.16,2.20,2*0A\r\n$GNGSA,A,3,,,,,,,,,,,,,3.09,2.16,2.20,3*0C\r\n$GNGSA,A,3,,,,,,,,,,,,,3.09,2.16,2.20,4*0B\r\n$GPGSV,2,1,06,07,18,202,23,14,56,312,31,19,08,276,10,28,47,315,26,1*62\r\n$GPGSV,2,2,06,30,33,243,31,41,27,238,29,1*64\r\n$GPGSV,1,1,02,14,56,312,17,30,33,243,25,6*60\r\n$GPGSV,1,1,01,08,29,078,,0*58\r\n$GLGSV,1,1,03,78,65,278,28,79,22,328,33,81,26,263,31,1*4F\r\n$GLGSV,2,1,06,65,11,116,12,77,37,182,17,78,65,278,26,79,22,328,24,3*74\r\n$GLGSV,2,2,06,81,26,263,19,88,61,327,20,3*7D\r\n$GLGSV,1,1,03,71,06,028,,72,16,073,,87,40,030,,0*4E\r\n$GAGSV,1,1,00,0*74\r\n$GBGSV,1,1,00,0*77\r\n$GNGLL,3717.4895411,N,12708.8700356,E,065727.00,A,A*73\r\n$GNRMC,065728.00,A,3717.4897333,N,12708.8693164,E,0.304,,190421,,,A,V*1A\r\n$GNVTG,,T,,M,0.304,N,0.563,K,A*3A\r\n$GNGGA,065728.00,3717.4897333,N,12708.8693164,E,1,06,2.16,182.007,M,18.960,M,,*4D\r\n$GNGSA,A,3,14,28,30,07,,,,,,,,,3.09,2.16,2.20,1*05\r\n$GNGSA,A,3,79,88,81,,,,,,,,,,3.09,2.16,2.20,2*0A\r\n$GNGSA,A,3,,,,,,,,,,,,,3.09,2.16,2.20,3*0C\r\n$GNGSA,A,3,,,,,,,,,,,,,3.09,2.16,2.20,4*0B\r\n$GPGSV,2,1,06,07,18,202,22,14,56,312,31,19,08,276,08,28,47,315,26,1*6A\r\n$GPGSV,2,2,06,30,33,243,31,41,27,238,29,1*64\r\n$GPGSV,1,1,02,14,56,312,16,30,33,243,25,6*61\r\n$GPGSV,1,1,01,08,29,078,,0*58\r\n$GLGSV,1,1,03,78,65,278,28,79,22,328,33,81,26,263,30,1*4E\r\n$GLGSV,2,1,06,65,11,116,10,77,37,182,17,78,65,278,26,79,22,328,24,3*76\r\n$GLGSV,2,2,06,81,26,263,19,88,61,327,19,3*77\r\n$GLGSV,1,1,03,71,06,028,,72,16,073,,87,40,030,,0*4E\r\n$GAGSV,1,1,00,0*74\r\n$GBGSV,1,1,00,0*77\r\n$GNGLL,3717.4897333,N,12708.8693164,E,065728.00,A,A*71\r\n$GNRMC,065729.00,A,3717.4898752,N,12708.8688033,E,0.268,,190421,,,A,V*15\r\n$GNVTG,,T,,M,0.268,N,0.496,K,A*3A\r\n$GNGGA,065729.00,3717.4898752,N,12708.8688033,E,1,06,2.16,182.489,M,18.960,M,,*4B\r\n$GNGSA,A,3,14,28,30,07,,,,,,,,,3.09,2.16,2.20,1*05\r\n$GNGSA,A,3,79,88,81,,,,,,,,,,3.09,2.16,2.20,2*0A\r\n$GNGSA,A,3,,,,,,,,,,,,,3.09,2.16,2.20,3*0C\r\n$GNGSA,A,3,,,,,,,,,,,,,3.09,2.16,2.20,4*0B\r\n$GPGSV,2,1,06,07,18,202,22,14,56,312,31,19,08,276,09,28,47,315,25,1*68\r\n$GPGSV,2,2,06,30,33,243,30,41,27,238,29,1*65\r\n$GPGSV,1,1,02,14,56,312,16,30,33,243,25,6*61\r\n$GPGSV,1,1,01,08,29,078,,0*58\r\n$GLGSV,1,1,03,78,65,278,28,79,22,328,33,81,26,263,30,1*4E\r\n$GLGSV,2,1,06,65,11,116,09,77,37,182,16,78,65,278,26,79,22,328,23,3*78\r\n$GLGSV,2,2,06,81,26,263,19,88,61,327,19,3*77\r\n$GLGSV,1,1,03,71,06,027,,72,16,073,,87,40,030,,0*41\r\n$GAGSV,1,1,00,0*74\r\n$GBGSV,1,1,00,0*77\r\n$GNGLL,3717.4898752,N,12708.8688033,E,065729.00,A,A*75\r\n$GNRMC,065730.00,A,3717.4899702,N,12708.8685351,E,0.264,,190421,,,A,V*1F\r\n$GNVTG,,T,,M,0.264,N,0.489,K,A*38\r\n$GNGGA,065730.00,3717.4899702,N,12708.8685351,E,1,06,2.16,182.872,M,18.960,M,,*45\r\n$GNGSA,A,3,14,28,30,07,,,,,,,,,3.09,2.16,2.20,1*05\r\n$GNGSA,A,3,79,88,81,,,,,,,,,,3.09,2.16,2.20,2*0A\r\n$GNGSA,A,3,,,,,,,,,,,,,3.09,2.16,2.20,3*0C\r\n$GNGSA,A,3,,,,,,,,,,,,,3.09,2.16,2.20,4*0B\r\n$GPGSV,2,1,06,07,18,202,22,14,56,312,31,19,08,276,11,28,47,315,26,1*62\r\n$GPGSV,2,2,06,30,33,243,31,41,27,238,29,1*64\r\n$GPGSV,1,1,02,14,56,312,17,30,33,243,25,6*60\r\n$GPGSV,1,1,01,08,29,078,,0*58\r\n$GLGSV,1,1,03,78,65,278,28,79,22,328,33,81,26,263,30,1*4E\r\n$GLGSV,2,1,05,77,37,182,16,78,65,278,27,79,22,328,24,81,26,263,17,3*7D\r\n$GLGSV,2,2,05,88,61,327,19,3*46\r\n$GLGSV,1,1,04,65,11,116,,71,06,027,,72,16,073,,87,40,030,,0*73\r\n$GAGSV,1,1,00,0*74\r\n$GBGSV,1,1,00,0*77\r\n$GNGLL,3717.4899702,N,12708.8685351,E,065730.00,A,A*73\r\n$GNRMC,065731.00,A,3717.4901350,N,12708.8679233,E,0.287,,190421,,,A,V*16\r\n$GNVTG,,T,,M,0.287,N,0.531,K,A*37\r\n$GNGGA,065731.00,3717.4901350,N,12708.8679233,E,1,06,2.16,183.371,M,18.960,M,,*48\r\n$GNGSA,A,3,14,28,30,07,,,,,,,,,3.09,2.16,2.20,1*05\r\n$GNGSA,A,3,79,88,81,,,,,,,,,,3.09,2.16,2.20,2*0A\r\n$GNGSA,A,3,,,,,,,,,,,,,3.09,2.16,2.20,3*0C\r\n$GNGSA,A,3,,,,,,,,,,,,,3.09,2.16,2.20,4*0B\r\n$GPGSV,2,1,06,07,18,202,22,14,56,312,31,19,08,276,09,28,47,315,26,1*6B\r\n$GPGSV,2,2,06,30,33,243,31,41,27,238,30,1*6C\r\n$GPGSV,1,1,02,14,56,312,16,30,33,243,25,6*61\r\n$GPGSV,1,1,01,08,29,078,,0*58\r\n$GLGSV,1,1,03,78,65,278,27,79,22,328,33,81,26,263,30,1*41\r\n$GLGSV,2,1,05,77,37,182,17,78,65,278,27,79,22,328,25,81,26,263,18,3*72\r\n$GLGSV,2,2,05,88,61,327,19,3*46\r\n$GLGSV,1,1,04,65,11,116,,71,06,027,,72,16,073,,87,40,030,,0*73\r\n$GAGSV,1,1,00,0*74\r\n$GBGSV,1,1,00,0*77\r\n$GNGLL,3717.4901350,N,12708.8679233,E,065731.00,A,A*77\r\n$GNRMC,065732.00,A,3717.4903049,N,12708.8672950,E,0.366,,190421,,,A,V*17\r\n$GNVTG,,T,,M,0.366,N,0.677,K,A*38\r\n$GNGGA,065732.00,3717.4903049,N,12708.8672950,E,1,06,2.16,183.940,M,18.960,M,,*4F\r\n$GNGSA,A,3,14,28,30,07,,,,,,,,,3.09,2.16,2.20,1*05\r\n$GNGSA,A,3,79,88,81,,,,,,,,,,3.09,2.16,2.20,2*0A\r\n$GNGSA,A,3,,,,,,,,,,,,,3.09,2.16,2.20,3*0C\r\n$GNGSA,A,3,,,,,,,,,,,,,3.09,2.16,2.20,4*0B\r\n$GPGSV,2,1,06,07,18,202,22,14,56,312,31,19,08,276,08,28,47,315,26,1*6A\r\n$GPGSV,2,2,06,30,33,243,31,41,27,238,30,1*6C\r\n$GPGSV,1,1,02,14,56,312,16,30,33,243,26,6*62\r\n$GPGSV,1,1,01,08,29,078,,0*58\r\n$GLGSV,1,1,03,78,65,278,28,79,22,328,33,81,26,263,29,1*46\r\n$GLGSV,2,1,05,77,37,182,17,78,65,278,26,79,22,328,24,81,26,263,18,3*72\r\n$GLGSV,2,2,05,88,61,327,19,3*46\r\n$GLGSV,1,1,04,65,11,116,,71,06,027,,72,16,073,,87,40,030,,0*73\r\n$GAGSV,1,1,00,0*74\r\n$GBGSV,1,1,00,0*77\r\n$GNGLL,3717.4903049,N,12708.8672950,E,065732.00,A,A*78\r\n$GNRMC,065733.00,A,3717.4903977,N,12708.8669550,E,0.253,,190421,,,A,V*13\r\n$GNVTG,,T,,M,0.253,N,0.469,K,A*32\r\n$GNGGA,065733.00,3717.4903977,N,12708.8669550,E,1,06,2.16,184.217,M,18.960,M,,*42\r\n$GNGSA,A,3,14,28,30,07,,,,,,,,,3.09,2.16,2.20,1*05\r\n$GNGSA,A,3,79,88,81,,,,,,,,,,3.09,2.16,2.20,2*0A\r\n$GNGSA,A,3,,,,,,,,,,,,,3.09,2.16,2.20,3*0C\r\n$GNGSA,A,3,,,,,,,,,,,,,3.09,2.16,2.20,4*0B\r\n$GPGSV,2,1,06,07,18,202,22,14,56,312,31,19,08,276,12,28,47,315,25,1*62\r\n$GPGSV,2,2,06,30,33,243,31,41,27,238,30,1*6C\r\n$GPGSV,1,1,02,14,56,312,15,30,33,243,26,6*61\r\n$GPGSV,1,1,01,08,29,078,,0*58\r\n$GLGSV,1,1,03,78,65,278,28,79,22,328,33,81,26,263,30,1*4E\r\n$GLGSV,2,1,05,77,37,182,17,78,65,278,26,79,22,328,24,81,26,263,17,3*7D\r\n$GLGSV,2,2,05,88,61,327,19,3*46\r\n$GLGSV,1,1,04,65,11,116,,71,06,027,,72,16,073,,87,40,030,,0*73\r\n$GAGSV,1,1,00,0*74\r\n$GBGSV,1,1,00,0*77\r\n$GNGLL,3717.4903977,N,12708.8669550,E,065733.00,A,A*7B\r\n$GNRMC,065734.00,A,3717.4904952,N,12708.8665031,E,0.326,,190421,,,A,V*19\r\n$GNVTG,,T,,M,0.326,N,0.604,K,A*38\r\n$GNGGA,065734.00,3717.4904952,N,12708.8665031,E,1,06,2.16,184.634,M,18.960,M,,*4E\r\n$GNGSA,A,3,14,28,30,07,,,,,,,,,3.09,2.16,2.20,1*05\r\n$GNGSA,A,3,79,88,81,,,,,,,,,,3.09,2.16,2.20,2*0A\r\n$GNGSA,A,3,,,,,,,,,,,,,3.09,2.16,2.20,3*0C\r\n$GNGSA,A,3,,,,,,,,,,,,,3.09,2.16,2.20,4*0B\r\n$GPGSV,2,1,06,07,18,202,20,14,56,312,31,19,08,276,09,28,47,315,25,1*6A\r\n$GPGSV,2,2,06,30,33,243,31,41,27,238,29,1*64\r\n$GPGSV,1,1,02,14,56,312,15,30,33,243,26,6*61\r\n$GPGSV,1,1,01,08,29,078,,0*58\r\n$GLGSV,1,1,03,78,65,278,28,79,22,328,33,81,26,263,30,1*4E\r\n$GLGSV,2,1,05,77,37,182,17,78,65,278,26,79,22,328,25,81,26,263,17,3*7C\r\n$GLGSV,2,2,05,88,61,327,19,3*46\r\n$GLGSV,1,1,04,65,11,116,,71,06,027,,72,16,073,,87,40,030,,0*73\r\n$GAGSV,1,1,00,0*74\r\n$GBGSV,1,1,00,0*77\r\n$GNGLL,3717.4904952,N,12708.8665031,E,065734.00,A,A*72\r\n$GNRMC,065735.00,A,3717.4905423,N,12708.8663578,E,0.235,,190421,,,A,V*1F\r\n$GNVTG,,T,,M,0.235,N,0.435,K,A*3B\r\n$GNGGA,065735.00,3717.4905423,N,12708.8663578,E,1,06,2.16,185.052,M,18.960,M,,*4C\r\n$GNGSA,A,3,14,28,30,07,,,,,,,,,3.09,2.16,2.20,1*05\r\n$GNGSA,A,3,79,88,81,,,,,,,,,,3.09,2.16,2.20,2*0A\r\n$GNGSA,A,3,,,,,,,,,,,,,3.09,2.16,2.20,3*0C\r\n$GNGSA,A,3,,,,,,,,,,,,,3.09,2.16,2.20,4*0B\r\n$GPGSV,2,1,06,07,18,202,20,14,56,312,31,19,08,276,08,28,47,315,25,1*6B\r\n$GPGSV,2,2,06,30,33,243,31,41,27,238,30,1*6C\r\n$GPGSV,1,1,02,14,56,312,16,30,33,243,25,6*61\r\n$GPGSV,1,1,01,08,29,078,,0*58\r\n$GLGSV,1,1,03,78,65,278,27,79,22,328,33,81,26,263,30,1*41\r\n$GLGSV,2,1,05,77,37,182,16,78,65,278,26,79,22,328,25,81,26,263,17,3*7D\r\n$GLGSV,2,2,05,88,61,327,19,3*46\r\n$GLGSV,1,1,04,65,11,116,,71,06,027,,72,16,073,,87,40,030,,0*73\r\n$GAGSV,1,1,00,0*74\r\n$GBGSV,1,1,00,0*77\r\n$GNGLL,3717.4905423,N,12708.8663578,E,065735.00,A,A*77\r\n$GNRMC,065736.00,A,3717.4906558,N,12708.8660359,E,0.261,,190421,,,A,V*15\r\n$GNVTG,,T,,M,0.261,N,0.483,K,A*37\r\n$GNGGA,065736.00,3717.4906558,N,12708.8660359,E,1,06,2.16,185.536,M,18.960,M,,*40\r\n$GNGSA,A,3,14,28,30,07,,,,,,,,,3.09,2.16,2.20,1*05\r\n$GNGSA,A,3,79,88,81,,,,,,,,,,3.09,2.16,2.20,2*0A\r\n$GNGSA,A,3,,,,,,,,,,,,,3.09,2.16,2.20,3*0C\r\n$GNGSA,A,3,,,,,,,,,,,,,3.09,2.16,2.20,4*0B\r\n$GPGSV,2,1,06,07,18,202,20,14,56,312,31,19,08,276,12,28,47,315,25,1*60\r\n$GPGSV,2,2,06,30,33,243,31,41,27,238,30,1*6C\r\n$GPGSV,1,1,02,14,56,312,16,30,33,243,25,6*61\r\n$GPGSV,1,1,01,08,29,078,,0*58\r\n$GLGSV,1,1,02,79,22,328,33,81,26,263,30,1*74\r\n$GLGSV,2,1,05,77,37,182,17,78,65,276,26,79,22,328,25,81,26,263,18,3*7D\r\n$GLGSV,2,2,05,88,61,327,19,3*46\r\n$GLGSV,1,1,04,65,11,116,,71,06,027,,72,16,073,,87,40,030,,0*73\r\n$GAGSV,1,1,00,0*74\r\n$GBGSV,1,1,00,0*77\r\n$GNGLL,3717.4906558,N,12708.8660359,E,065736.00,A,A*7C\r\n$GNRMC,065737.00,A,3717.4906920,N,12708.8659769,E,0.102,,190421,,,A,V*1C\r\n$GNVTG,,T,,M,0.102,N,0.189,K,A*3E\r\n$GNGGA,065737.00,3717.4906920,N,12708.8659769,E,1,06,2.16,185.904,M,18.960,M,,*42\r\n$GNGSA,A,3,14,28,30,07,,,,,,,,,3.09,2.16,2.20,1*05\r\n$GNGSA,A,3,79,88,81,,,,,,,,,,3.09,2.16,2.20,2*0A\r\n$GNGSA,A,3,,,,,,,,,,,,,3.09,2.16,2.20,3*0C\r\n$GNGSA,A,3,,,,,,,,,,,,,3.09,2.16,2.20,4*0B\r\n$GPGSV,2,1,06,07,18,202,19,14,56,312,31,19,08,276,08,28,47,315,24,1*60\r\n$GPGSV,2,2,06,30,33,243,31,41,27,238,30,1*6C\r\n$GPGSV,1,1,02,14,56,312,16,30,33,243,25,6*61\r\n$GPGSV,1,1,01,08,29,078,,0*58\r\n$GLGSV,1,1,03,78,65,276,25,79,22,328,33,81,26,263,29,1*45\r\n$GLGSV,2,1,05,77,37,182,17,78,65,276,27,79,22,328,25,81,26,263,17,3*73\r\n$GLGSV,2,2,05,88,61,327,19,3*46\r\n$GLGSV,1,1,04,65,11,116,,71,06,027,,72,16,073,,87,40,030,,0*73\r\n$GAGSV,1,1,00,0*74\r\n$GBGSV,1,1,00,0*77\r\n$GNGLL,3717.4906920,N,12708.8659769,E,065737.00,A,A*73\r\n$GNRMC,065738.00,A,3717.4907098,N,12708.8658942,E,0.012,,190421,,,A,V*1E\r\n$GNVTG,,T,,M,0.012,N,0.022,K,A*3E\r\n$GNGGA,065738.00,3717.4907098,N,12708.8658942,E,1,06,2.16,186.185,M,18.960,M,,*42\r\n$GNGSA,A,3,14,28,30,07,,,,,,,,,3.09,2.16,2.20,1*05\r\n$GNGSA,A,3,79,88,81,,,,,,,,,,3.09,2.16,2.20,2*0A\r\n$GNGSA,A,3,,,,,,,,,,,,,3.09,2.16,2.20,3*0C\r\n$GNGSA,A,3,,,,,,,,,,,,,3.09,2.16,2.20,4*0B\r\n$GPGSV,2,1,06,07,18,202,17,14,56,312,31,19,08,276,09,28,47,315,24,1*6F\r\n$GPGSV,2,2,06,30,33,243,32,41,27,238,30,1*6F\r\n$GPGSV,1,1,02,14,56,312,15,30,33,243,26,6*61\r\n$GPGSV,1,1,01,08,29,078,,0*58\r\n$GLGSV,1,1,03,78,65,276,25,79,22,328,33,81,26,263,29,1*45\r\n$GLGSV,2,1,05,77,37,182,16,78,65,276,27,79,22,328,25,81,26,263,17,3*72\r\n$GLGSV,2,2,05,88,61,327,19,3*46\r\n$GLGSV,1,1,04,65,11,116,,71,06,027,,72,16,073,,87,40,030,,0*73\r\n$GAGSV,1,1,00,0*74\r\n$GBGSV,1,1,00,0*77\r\n$GNGLL,3717.4907098,N,12708.8658942,E,065738.00,A,A*71\r\n$GNRMC,065739.00,A,3717.4906567,N,12708.8659543,E,0.188,,190421,,,A,V*15\r\n$GNVTG,,T,,M,0.188,N,0.349,K,A*32\r\n$GNGGA,065739.00,3717.4906567,N,12708.8659543,E,1,06,2.16,186.337,M,18.960,M,,*40\r\n$GNGSA,A,3,14,28,30,07,,,,,,,,,3.09,2.16,2.20,1*05\r\n$GNGSA,A,3,79,88,81,,,,,,,,,,3.09,2.16,2.20,2*0A\r\n$GNGSA,A,3,,,,,,,,,,,,,3.09,2.16,2.20,3*0C\r\n$GNGSA,A,3,,,,,,,,,,,,,3.09,2.16,2.20,4*0B\r\n$GPGSV,2,1,06,07,18,202,16,14,56,312,31,19,08,276,09,28,47,315,22,1*68\r\n$GPGSV,2,2,06,30,33,243,31,41,27,238,29,1*64\r\n$GPGSV,1,1,02,14,56,312,16,30,33,243,25,6*61\r\n$GPGSV,1,1,01,08,29,078,,0*58\r\n$GLGSV,1,1,02,79,22,328,33,81,27,263,29,1*7D\r\n$GLGSV,2,1,05,77,37,182,16,78,65,276,27,79,22,328,24,81,27,263,16,3*73\r\n$GLGSV,2,2,05,88,61,327,19,3*46\r\n$GLGSV,1,1,04,65,11,116,,71,06,027,,72,16,073,,87,40,030,,0*73\r\n$GAGSV,1,1,00,0*74\r\n$GBGSV,1,1,00,0*77\r\n$GNGLL,3717.4906567,N,12708.8659543,E,065739.00,A,A*78\r\n$GNRMC,065740.00,A,3717.4906085,N,12708.8661048,E,0.148,,190421,,,A,V*1B\r\n$GNVTG,,T,,M,0.148,N,0.275,K,A*30\r\n$GNGGA,065740.00,3717.4906085,N,12708.8661048,E,1,06,2.16,186.486,M,18.960,M,,*4F\r\n$GNGSA,A,3,14,28,30,07,,,,,,,,,3.09,2.16,2.20,1*05\r\n$GNGSA,A,3,79,88,81,,,,,,,,,,3.09,2.16,2.20,2*0A\r\n$GNGSA,A,3,,,,,,,,,,,,,3.09,2.16,2.20,3*0C\r\n$GNGSA,A,3,,,,,,,,,,,,,3.09,2.16,2.20,4*0B\r\n$GPGSV,2,1,06,07,18,202,15,14,56,312,30,19,08,276,12,28,47,315,21,1*63\r\n$GPGSV,2,2,06,30,33,243,31,41,27,238,29,1*64\r\n$GPGSV,1,1,02,14,56,312,15,30,33,243,25,6*62\r\n$GPGSV,1,1,01,08,29,078,,0*58\r\n$GLGSV,1,1,02,79,22,328,33,81,27,263,29,1*7D\r\n$GLGSV,2,1,05,77,37,182,17,78,65,276,27,79,22,328,24,81,27,263,15,3*71\r\n$GLGSV,2,2,05,88,61,327,19,3*46\r\n$GLGSV,1,1,04,65,11,116,,71,06,027,,72,16,073,,87,40,030,,0*73\r\n$GAGSV,1,1,00,0*74\r\n$GBGSV,1,1,00,0*77\r\n$GNGLL,3717.4906085,N,12708.8661048,E,065740.00,A,A*7A\r\n$GNRMC,065741.00,A,3717.4906456,N,12708.8659623,E,0.116,,190421,,,A,V*1B\r\n$GNVTG,,T,,M,0.116,N,0.215,K,A*3D\r\n$GNGGA,065741.00,3717.4906456,N,12708.8659623,E,1,06,2.16,186.678,M,18.960,M,,*47\r\n$GNGSA,A,3,14,28,30,07,,,,,,,,,3.09,2.16,2.20,1*05\r\n$GNGSA,A,3,79,88,81,,,,,,,,,,3.09,2.16,2.20,2*0A\r\n$GNGSA,A,3,,,,,,,,,,,,,3.09,2.16,2.20,3*0C\r\n$GNGSA,A,3,,,,,,,,,,,,,3.09,2.16,2.20,4*0B\r\n$GPGSV,2,1,06,07,18,202,15,14,56,312,31,19,08,276,12,28,47,315,21,1*62\r\n$GPGSV,2,2,06,30,33,243,31,41,27,238,29,1*64\r\n$GPGSV,1,1,02,14,56,312,15,30,33,243,25,6*62\r\n$GPGSV,1,1,01,08,29,078,,0*58\r\n$GLGSV,1,1,02,79,22,328,33,81,27,263,29,1*7D\r\n$GLGSV,2,1,05,77,37,182,17,78,65,276,27,79,22,328,23,81,27,263,14,3*77\r\n$GLGSV,2,2,05,88,61,327,19,3*46\r\n$GLGSV,1,1,04,65,11,116,,71,06,027,,72,16,073,,87,40,030,,0*73\r\n$GAGSV,1,1,00,0*74\r\n$GBGSV,1,1,00,0*77\r\n$GNGLL,3717.4906456,N,12708.8659623,E,065741.00,A,A*71\r\n$GNRMC,065742.00,A,3717.4906263,N,12708.8659455,E,0.132,,190421,,,A,V*1D\r\n$GNVTG,,T,,M,0.132,N,0.245,K,A*3E\r\n$GNGGA,065742.00,3717.4906263,N,12708.8659455,E,1,06,2.16,186.792,M,18.960,M,,*42\r\n$GNGSA,A,3,14,28,30,07,,,,,,,,,3.09,2.16,2.20,1*05\r\n$GNGSA,A,3,79,88,81,,,,,,,,,,3.09,2.16,2.20,2*0A\r\n$GNGSA,A,3,,,,,,,,,,,,,3.09,2.16,2.20,3*0C\r\n$GNGSA,A,3,,,,,,,,,,,,,3.09,2.16,2.20,4*0B\r\n$GPGSV,2,1,06,07,18,202,14,14,56,312,30,19,08,276,10,28,47,315,19,1*6B\r\n$GPGSV,2,2,06,30,33,243,31,41,27,238,28,1*65\r\n$GPGSV,1,1,02,14,56,312,15,30,33,243,25,6*62\r\n$GPGSV,1,1,01,08,29,078,,0*58\r\n$GLGSV,1,1,02,79,22,328,33,81,27,263,28,1*7C\r\n$GLGSV,1,1,04,77,37,182,17,78,65,276,27,79,22,328,23,88,61,327,19,3*72\r\n$GLGSV,1,1,04,65,11,116,,71,06,027,,72,16,073,,87,40,030,,0*73\r\n$GAGSV,1,1,00,0*74\r\n$GBGSV,1,1,00,0*77\r\n$GNGLL,3717.4906263,N,12708.8659455,E,065742.00,A,A*71\r\n$GNRMC,065743.00,A,3717.4905533,N,12708.8661887,E,0.240,,190421,,,A,V*13\r\n$GNVTG,,T,,M,0.240,N,0.444,K,A*3F\r\n$GNGGA,065743.00,3717.4905533,N,12708.8661887,E,1,06,2.16,186.776,M,18.960,M,,*40\r\n$GNGSA,A,3,14,28,30,07,,,,,,,,,3.09,2.16,2.21,1*04\r\n$GNGSA,A,3,79,88,81,,,,,,,,,,3.09,2.16,2.21,2*0B\r\n$GNGSA,A,3,,,,,,,,,,,,,3.09,2.16,2.21,3*0D\r\n$GNGSA,A,3,,,,,,,,,,,,,3.09,2.16,2.21,4*0A\r\n$GPGSV,2,1,06,07,18,202,12,14,56,312,30,19,08,276,11,28,47,315,19,1*6C\r\n$GPGSV,2,2,06,30,33,243,31,41,27,238,29,1*64\r\n$GPGSV,1,1,02,14,56,312,14,30,33,243,25,6*63\r\n$GPGSV,1,1,01,08,29,078,,0*58\r\n$GLGSV,1,1,02,79,22,328,33,81,27,263,29,1*7D\r\n$GLGSV,1,1,04,77,37,182,16,78,65,276,27,79,22,328,22,88,61,327,18,3*73\r\n$GLGSV,1,1,04,65,11,116,,71,06,027,,72,16,073,,87,40,030,,0*73\r\n$GAGSV,1,1,00,0*74\r\n$GBGSV,1,1,00,0*77\r\n$GNGLL,3717.4905533,N,12708.8661887,E,065743.00,A,A*79\r\n$GNRMC,065744.00,A,3717.4905354,N,12708.8661482,E,0.139,,190421,,,A,V*17\r\n$GNVTG,,T,,M,0.139,N,0.257,K,A*36\r\n$GNGGA,065744.00,3717.4905354,N,12708.8661482,E,1,06,6.02,186.753,M,18.960,M,,*4F\r\n$GNGSA,A,3,14,28,30,,,,,,,,,,7.45,6.02,4.39,1*01\r\n$GNGSA,A,3,79,88,81,,,,,,,,,,7.45,6.02,4.39,2*09\r\n$GNGSA,A,3,,,,,,,,,,,,,7.45,6.02,4.39,3*0F\r\n$GNGSA,A,3,,,,,,,,,,,,,7.45,6.02,4.39,4*08\r\n$GPGSV,2,1,06,07,18,202,10,14,56,312,30,19,08,276,13,28,47,315,17,1*62\r\n$GPGSV,2,2,06,30,33,243,31,41,27,238,29,1*64\r\n$GPGSV,1,1,02,14,56,312,14,30,33,243,25,6*63\r\n$GPGSV,1,1,01,08,29,078,,0*58\r\n$GLGSV,1,1,03,79,22,328,33,81,27,263,28,88,61,327,31,1*4E\r\n$GLGSV,1,1,04,77,37,182,15,78,65,276,26,79,22,328,22,88,61,327,18,3*71\r\n$GLGSV,1,1,04,65,11,116,,71,06,027,,72,16,073,,87,40,030,,0*73\r\n$GAGSV,1,1,00,0*74\r\n$GBGSV,1,1,00,0*77\r\n$GNGLL,3717.4905354,N,12708.8661482,E,065744.00,A,A*70\r\n$GNRMC,065745.00,A,3717.4904387,N,12708.8662721,E,0.233,,190421,,,A,V*19\r\n$GNVTG,,T,,M,0.233,N,0.431,K,A*39\r\n$GNGGA,065745.00,3717.4904387,N,12708.8662721,E,1,06,6.02,186.776,M,18.960,M,,*4F\r\n$GNGSA,A,3,14,28,30,,,,,,,,,,7.45,6.02,4.39,1*01\r\n$GNGSA,A,3,79,88,81,,,,,,,,,,7.45,6.02,4.39,2*09\r\n$GNGSA,A,3,,,,,,,,,,,,,7.45,6.02,4.39,3*0F\r\n$GNGSA,A,3,,,,,,,,,,,,,7.45,6.02,4.39,4*08\r\n$GPGSV,2,1,06,07,18,202,09,14,56,312,30,19,08,276,07,28,47,315,17,1*6F\r\n$GPGSV,2,2,06,30,33,243,31,41,27,238,29,1*64\r\n$GPGSV,1,1,02,14,56,312,16,30,33,243,25,6*61\r\n$GPGSV,1,1,01,08,29,078,,0*58\r\n$GLGSV,1,1,02,79,22,328,33,81,27,263,28,1*7C\r\n$GLGSV,1,1,04,77,37,182,14,78,65,276,26,79,22,328,22,88,61,327,17,3*7F\r\n$GLGSV,1,1,04,65,11,116,,71,06,027,,72,16,073,,87,39,031,,0*7C\r\n$GAGSV,1,1,00,0*74\r\n$GBGSV,1,1,00,0*77\r\n$GNGLL,3717.4904387,N,12708.8662721,E,065745.00,A,A*77\r\n$GNRMC,065746.00,A,3717.4903986,N,12708.8663587,E,0.102,,190421,,,A,V*18\r\n$GNVTG,,T,,M,0.102,N,0.189,K,A*3E\r\n$GNGGA,065746.00,3717.4903986,N,12708.8663587,E,1,05,6.02,186.736,M,18.960,M,,*48\r\n$GNGSA,A,3,14,28,30,,,,,,,,,,7.45,6.02,4.39,1*01\r\n$GNGSA,A,3,79,88,81,,,,,,,,,,7.45,6.02,4.39,2*09\r\n$GNGSA,A,3,,,,,,,,,,,,,7.45,6.02,4.39,3*0F\r\n$GNGSA,A,3,,,,,,,,,,,,,7.45,6.02,4.39,4*08\r\n$GPGSV,2,1,06,07,18,202,10,14,56,312,30,19,08,276,09,28,47,315,18,1*66\r\n$GPGSV,2,2,06,30,33,243,31,41,27,238,29,1*64\r\n$GPGSV,1,1,02,14,56,312,17,30,33,243,25,6*60\r\n$GPGSV,1,1,01,08,29,078,,0*58\r\n$GLGSV,1,1,02,79,22,328,32,81,27,263,27,1*72\r\n$GLGSV,1,1,04,77,37,182,14,78,65,276,26,79,22,328,22,88,61,328,18,3*7F\r\n$GLGSV,1,1,04,65,11,116,,71,06,027,,72,16,073,,87,39,031,,0*7C\r\n$GAGSV,1,1,00,0*74\r\n$GBGSV,1,1,00,0*77\r\n$GNGLL,3717.4903986,N,12708.8663587,E,065746.00,A,A*77\r\n$GNRMC,065747.00,A,3717.4903931,N,12708.8662961,E,0.142,,190421,,,A,V*14\r\n$GNVTG,,T,,M,0.142,N,0.263,K,A*3D\r\n$GNGGA,065747.00,3717.4903931,N,12708.8662961,E,1,05,6.02,186.767,M,18.960,M,,*44\r\n$GNGSA,A,3,14,28,30,,,,,,,,,,7.44,6.02,4.39,1*00\r\n$GNGSA,A,3,79,88,81,,,,,,,,,,7.44,6.02,4.39,2*08\r\n$GNGSA,A,3,,,,,,,,,,,,,7.44,6.02,4.39,3*0E\r\n$GNGSA,A,3,,,,,,,,,,,,,7.44,6.02,4.39,4*09\r\n$GPGSV,2,1,06,07,18,202,10,14,56,312,30,19,08,276,08,28,47,315,19,1*66\r\n$GPGSV,2,2,06,30,33,243,31,41,27,238,29,1*64\r\n$GPGSV,1,1,02,14,56,312,17,30,33,243,25,6*60\r\n$GPGSV,1,1,01,08,29,078,,0*58\r\n$GLGSV,1,1,02,79,22,328,32,81,27,263,28,1*7D\r\n$GLGSV,1,1,04,77,37,182,15,78,65,276,26,79,22,328,22,88,61,328,18,3*7E\r\n$GLGSV,1,1,04,65,11,116,,71,06,027,,72,16,073,,87,39,031,,0*7C\r\n$GAGSV,1,1,00,0*74\r\n$GBGSV,1,1,00,0*77\r\n$GNGLL,3717.4903931,N,12708.8662961,E,065747.00,A,A*7F\r\n$GNRMC,065748.00,A,3717.4905610,N,12708.8656108,E,0.068,,190421,,,A,V*18\r\n$GNVTG,,T,,M,0.068,N,0.127,K,A*37\r\n$GNGGA,065748.00,3717.4905610,N,12708.8656108,E,1,06,2.16,187.182,M,18.960,M,,*4F\r\n$GNGSA,A,3,14,28,30,07,,,,,,,,,3.09,2.16,2.21,1*04\r\n$GNGSA,A,3,79,88,81,,,,,,,,,,3.09,2.16,2.21,2*0B\r\n$GNGSA,A,3,,,,,,,,,,,,,3.09,2.16,2.21,3*0D\r\n$GNGSA,A,3,,,,,,,,,,,,,3.09,2.16,2.21,4*0A\r\n$GPGSV,2,1,06,07,18,202,10,14,56,312,30,19,08,276,09,28,47,315,20,1*6D\r\n$GPGSV,2,2,06,30,33,243,32,41,27,238,29,1*67\r\n$GPGSV,1,1,02,14,56,312,17,30,33,243,25,6*60\r\n$GPGSV,1,1,01,08,29,078,,0*58\r\n$GLGSV,1,1,02,79,22,328,32,81,27,263,28,1*7D\r\n$GLGSV,1,1,04,77,37,182,16,78,65,276,26,79,22,328,22,88,61,328,18,3*7D\r\n$GLGSV,1,1,04,65,11,116,,71,06,027,,72,16,073,,87,39,031,,0*7C\r\n$GAGSV,1,1,00,0*74\r\n$GBGSV,1,1,00,0*77\r\n$GNGLL,3717.4905610,N,12708.8656108,E,065748.00,A,A*7A\r\n$GNRMC,065749.00,A,3717.4906761,N,12708.8653263,E,0.233,,190421,,,A,V*1A\r\n$GNVTG,,T,,M,0.233,N,0.431,K,A*39\r\n$GNGGA,065749.00,3717.4906761,N,12708.8653263,E,1,06,2.16,187.552,M,18.960,M,,*48\r\n$GNGSA,A,3,14,28,30,07,,,,,,,,,3.09,2.16,2.21,1*04\r\n$GNGSA,A,3,79,88,81,,,,,,,,,,3.09,2.16,2.21,2*0B\r\n$GNGSA,A,3,,,,,,,,,,,,,3.09,2.16,2.21,3*0D\r\n$GNGSA,A,3,,,,,,,,,,,,,3.09,2.16,2.21,4*0A\r\n$GPGSV,2,1,06,07,18,202,08,14,56,312,30,19,08,276,10,28,47,315,21,1*6D\r\n$GPGSV,2,2,06,30,33,243,31,41,27,238,29,1*64\r\n$GPGSV,1,1,02,14,56,312,18,30,33,243,24,6*6E\r\n$GPGSV,1,1,01,08,29,078,,0*58\r\n$GLGSV,1,1,02,79,22,328,32,81,27,263,28,1*7D\r\n$GLGSV,2,1,05,77,37,182,16,78,65,276,26,79,22,328,22,81,27,263,26,3*77\r\n$GLGSV,2,2,05,88,61,328,18,3*48\r\n$GLGSV,1,1,04,65,11,116,,71,06,027,,72,16,073,,87,39,031,,0*7C\r\n$GAGSV,1,1,00,0*74\r\n$GBGSV,1,1,00,0*77\r\n$GNGLL,3717.4906761,N,12708.8653263,E,065749.00,A,A*74\r\n$GNRMC,065750.00,A,3717.4906478,N,12708.8653069,E,0.157,,190421,,,A,V*10\r\n$GNVTG,,T,,M,0.157,N,0.290,K,A*35\r\n$GNGGA,065750.00,3717.4906478,N,12708.8653069,E,1,06,2.16,187.568,M,18.960,M,,*4A\r\n$GNGSA,A,3,14,28,30,07,,,,,,,,,3.09,2.16,2.21,1*04\r\n$GNGSA,A,3,79,88,81,,,,,,,,,,3.09,2.16,2.21,2*0B\r\n$GNGSA,A,3,,,,,,,,,,,,,3.09,2.16,2.21,3*0D\r\n$GNGSA,A,3,,,,,,,,,,,,,3.09,2.16,2.21,4*0A\r\n$GPGSV,2,1,06,07,18,202,08,14,56,312,31,19,08,276,09,28,47,315,20,1*65\r\n$GPGSV,2,2,06,30,33,243,31,41,27,238,29,1*64\r\n$GPGSV,1,1,02,14,56,312,17,30,33,243,25,6*60\r\n$GPGSV,1,1,01,08,29,078,,0*58\r\n$GLGSV,1,1,02,79,22,328,32,81,27,263,28,1*7D\r\n$GLGSV,2,1,05,77,37,182,16,78,65,276,26,79,22,328,23,81,27,263,10,3*73\r\n$GLGSV,2,2,05,88,61,328,18,3*48\r\n$GLGSV,1,1,04,65,11,116,,71,06,027,,72,16,073,,87,39,031,,0*7C\r\n$GAGSV,1,1,00,0*74\r\n$GBGSV,1,1,00,0*77\r\n$GNGLL,3717.4906478,N,12708.8653069,E,065750.00,A,A*7F\r\n$GNRMC,065751.00,A,3717.4906529,N,12708.8652095,E,0.157,,190421,,,A,V*16\r\n$GNVTG,,T,,M,0.157,N,0.290,K,A*35\r\n$GNGGA,065751.00,3717.4906529,N,12708.8652095,E,1,06,2.16,187.581,M,18.960,M,,*4B\r\n$GNGSA,A,3,14,28,30,07,,,,,,,,,3.09,2.16,2.21,1*04\r\n$GNGSA,A,3,79,88,81,,,,,,,,,,3.09,2.16,2.21,2*0B\r\n$GNGSA,A,3,,,,,,,,,,,,,3.09,2.16,2.21,3*0D\r\n$GNGSA,A,3,,,,,,,,,,,,,3.09,2.16,2.21,4*0A\r\n$GPGSV,2,1,06,07,17,202,09,14,56,312,30,19,08,276,10,28,47,315,22,1*60\r\n$GPGSV,2,2,06,30,33,243,32,41,27,238,29,1*67\r\n$GPGSV,1,1,02,14,56,312,17,30,33,243,25,6*60\r\n$GPGSV,1,1,01,08,29,078,,0*58\r\n$GLGSV,1,1,02,79,22,328,32,81,27,263,28,1*7D\r\n$GLGSV,2,1,05,77,37,182,16,78,65,276,26,79,22,328,23,81,27,263,25,3*75\r\n$GLGSV,2,2,05,88,61,328,19,3*49\r\n$GLGSV,1,1,04,65,11,116,,71,06,027,,72,16,073,,87,39,031,,0*7C\r\n$GAGSV,1,1,00,0*74\r\n$GBGSV,1,1,00,0*77\r\n$GNGLL,3717.4906529,N,12708.8652095,E,065751.00,A,A*79\r\n$GNRMC,065752.00,A,3717.4906460,N,12708.8651009,E,0.212,,190421,,,A,V*1D\r\n$GNVTG,,T,,M,0.212,N,0.392,K,A*34\r\n$GNGGA,065752.00,3717.4906460,N,12708.8651009,E,1,06,2.16,187.543,M,18.960,M,,*4C\r\n$GNGSA,A,3,14,28,30,07,,,,,,,,,3.09,2.16,2.21,1*04\r\n$GNGSA,A,3,79,88,81,,,,,,,,,,3.09,2.16,2.21,2*0B\r\n$GNGSA,A,3,,,,,,,,,,,,,3.09,2.16,2.21,3*0D\r\n$GNGSA,A,3,,,,,,,,,,,,,3.09,2.16,2.21,4*0A\r\n$GPGSV,2,1,06,07,17,202,10,14,56,312,30,19,08,276,09,28,47,315,23,1*61\r\n$GPGSV,2,2,06,30,33,243,33,41,27,238,28,1*67\r\n$GPGSV,1,1,02,14,56,312,17,30,33,243,25,6*60\r\n$GPGSV,1,1,01,08,29,078,,0*58\r\n$GLGSV,1,1,02,79,22,328,32,81,27,263,28,1*7D\r\n$GLGSV,2,1,05,77,37,182,16,78,65,276,26,79,22,328,24,81,27,263,12,3*76\r\n$GLGSV,2,2,05,88,61,328,20,3*43\r\n$GLGSV,1,1,04,65,11,116,,71,06,027,,72,16,073,,87,39,031,,0*7C\r\n$GAGSV,1,1,00,0*74\r\n$GBGSV,1,1,00,0*77\r\n$GNGLL,3717.4906460,N,12708.8651009,E,065752.00,A,A*70\r\n$GNRMC,065753.00,A,3717.4906290,N,12708.8650986,E,0.230,,190421,,,A,V*1A\r\n$GNVTG,,T,,M,0.230,N,0.426,K,A*3C\r\n$GNGGA,065753.00,3717.4906290,N,12708.8650986,E,1,06,2.16,187.530,M,18.960,M,,*4F\r\n$GNGSA,A,3,14,28,30,07,,,,,,,,,3.09,2.16,2.21,1*04\r\n$GNGSA,A,3,79,88,81,,,,,,,,,,3.09,2.16,2.21,2*0B\r\n$GNGSA,A,3,,,,,,,,,,,,,3.09,2.16,2.21,3*0D\r\n$GNGSA,A,3,,,,,,,,,,,,,3.09,2.16,2.21,4*0A\r\n$GPGSV,2,1,06,07,17,202,11,14,56,312,30,19,08,276,08,28,47,315,24,1*66\r\n$GPGSV,2,2,06,30,33,243,33,41,27,238,27,1*68\r\n$GPGSV,1,1,02,14,56,312,17,30,33,243,25,6*60\r\n$GPGSV,1,1,01,08,29,078,,0*58\r\n$GLGSV,1,1,02,79,22,328,33,81,27,263,29,1*7D\r\n$GLGSV,2,1,05,77,37,182,16,78,65,276,26,79,22,328,25,81,27,263,13,3*76\r\n$GLGSV,2,2,05,88,61,328,20,3*43\r\n$GLGSV,1,1,04,65,11,116,,71,06,027,,72,16,073,,87,39,031,,0*7C\r\n$GAGSV,1,1,00,0*74\r\n$GBGSV,1,1,00,0*77\r\n$GNGLL,3717.4906290,N,12708.8650986,E,065753.00,A,A*77\r\n$GNRMC,065754.00,A,3717.4906396,N,12708.8649625,E,0.293,,190421,,,A,V*1D\r\n$GNVTG,,T,,M,0.293,N,0.542,K,A*36\r\n$GNGGA,065754.00,3717.4906396,N,12708.8649625,E,1,06,2.16,187.547,M,18.960,M,,*41\r\n$GNGSA,A,3,14,28,30,07,,,,,,,,,3.09,2.16,2.21,1*04\r\n$GNGSA,A,3,79,88,81,,,,,,,,,,3.09,2.16,2.21,2*0B\r\n$GNGSA,A,3,,,,,,,,,,,,,3.09,2.16,2.21,3*0D\r\n$GNGSA,A,3,,,,,,,,,,,,,3.09,2.16,2.21,4*0A\r\n$GPGSV,2,1,06,07,17,202,10,14,56,312,30,19,08,276,12,28,47,315,23,1*6B\r\n$GPGSV,2,2,06,30,33,243,33,41,27,238,27,1*68\r\n$GPGSV,1,1,02,14,56,312,17,30,33,243,25,6*60\r\n$GPGSV,1,1,01,08,29,078,,0*58\r\n$GLGSV,1,1,02,79,22,328,33,81,27,263,29,1*7D\r\n$GLGSV,2,1,05,77,37,182,16,78,65,276,27,79,22,328,25,81,27,263,13,3*77\r\n$GLGSV,2,2,05,88,61,328,20,3*43\r\n$GLGSV,1,1,04,65,11,116,,71,06,027,,72,16,073,,87,39,031,,0*7C\r\n$GAGSV,1,1,00,0*74\r\n$GBGSV,1,1,00,0*77\r\n$GNGLL,3717.4906396,N,12708.8649625,E,065754.00,A,A*79\r\n$GNRMC,065755.00,A,3717.4904978,N,12708.8653434,E,0.210,,190421,,,A,V*16\r\n$GNVTG,,T,,M,0.210,N,0.388,K,A*3D\r\n$GNGGA,065755.00,3717.4904978,N,12708.8653434,E,1,07,2.16,187.220,M,18.960,M,,*46\r\n$GNGSA,A,3,14,28,30,07,,,,,,,,,3.09,2.16,2.21,1*04\r\n$GNGSA,A,3,79,88,81,,,,,,,,,,3.09,2.16,2.21,2*0B\r\n$GNGSA,A,3,,,,,,,,,,,,,3.09,2.16,2.21,3*0D\r\n$GNGSA,A,3,,,,,,,,,,,,,3.09,2.16,2.21,4*0A\r\n$GPGSV,2,1,06,07,17,202,12,14,56,312,29,19,08,276,12,28,47,315,24,1*66\r\n$GPGSV,2,2,06,30,33,243,32,41,27,238,27,1*69\r\n$GPGSV,1,1,02,14,56,312,17,30,33,243,24,6*61\r\n$GPGSV,1,1,01,08,29,078,,0*58\r\n$GLGSV,1,1,02,79,22,328,32,81,27,263,29,1*7C\r\n$GLGSV,2,1,05,77,37,182,14,78,65,276,27,79,22,328,26,81,27,263,16,3*73\r\n$GLGSV,2,2,05,88,61,328,19,3*49\r\n$GLGSV,1,1,04,65,11,116,,71,06,027,,72,16,073,,87,39,031,,0*7C\r\n$GAGSV,1,1,00,0*74\r\n$GBGSV,1,1,00,0*77\r\n$GNGLL,3717.4904978,N,12708.8653434,E,065755.00,A,A*79\r\n$GNRMC,065756.00,A,3717.4904115,N,12708.8655819,E,0.098,,190421,,,A,V*11\r\n$GNVTG,,T,,M,0.098,N,0.182,K,A*37\r\n$GNGGA,065756.00,3717.4904115,N,12708.8655819,E,1,06,2.16,187.202,M,18.960,M,,*42\r\n$GNGSA,A,3,14,28,30,07,,,,,,,,,3.09,2.16,2.21,1*04\r\n$GNGSA,A,3,79,88,81,,,,,,,,,,3.09,2.16,2.21,2*0B\r\n$GNGSA,A,3,,,,,,,,,,,,,3.09,2.16,2.21,3*0D\r\n$GNGSA,A,3,,,,,,,,,,,,,3.09,2.16,2.21,4*0A\r\n$GPGSV,2,1,06,07,17,202,14,14,56,312,29,19,08,276,11,28,47,315,25,1*62\r\n$GPGSV,2,2,06,30,33,243,33,41,27,238,27,1*68\r\n$GPGSV,1,1,02,14,56,312,16,30,33,243,24,6*60\r\n$GPGSV,1,1,01,08,29,078,,0*58\r\n$GLGSV,1,1,02,79,22,328,32,81,27,263,29,1*7C\r\n$GLGSV,2,1,05,77,37,182,15,78,65,276,27,79,22,328,25,81,27,263,17,3*70\r\n$GLGSV,2,2,05,88,61,328,18,3*48\r\n$GLGSV,1,1,04,65,11,116,,71,06,027,,72,16,073,,87,39,031,,0*7C\r\n$GAGSV,1,1,00,0*74\r\n$GBGSV,1,1,00,0*77\r\n$GNGLL,3717.4904115,N,12708.8655819,E,065756.00,A,A*7C\r\n$GNRMC,065757.00,A,3717.4904121,N,12708.8654426,E,0.149,,190421,,,A,V*1B\r\n$GNVTG,,T,,M,0.149,N,0.276,K,A*32\r\n$GNGGA,065757.00,3717.4904121,N,12708.8654426,E,1,06,2.16,187.147,M,18.960,M,,*47\r\n$GNGSA,A,3,14,28,30,07,,,,,,,,,3.09,2.16,2.21,1*04\r\n$GNGSA,A,3,79,88,81,,,,,,,,,,3.09,2.16,2.21,2*0B\r\n$GNGSA,A,3,,,,,,,,,,,,,3.09,2.16,2.21,3*0D\r\n$GNGSA,A,3,,,,,,,,,,,,,3.09,2.16,2.21,4*0A\r\n$GPGSV,2,1,06,07,17,202,13,14,56,311,29,19,08,276,11,28,47,315,25,1*66\r\n$GPGSV,2,2,06,30,33,243,32,41,27,238,28,1*66\r\n$GPGSV,1,1,02,14,56,311,16,30,33,243,24,6*63\r\n$GPGSV,1,1,01,08,29,078,,0*58\r\n$GLGSV,1,1,02,79,22,328,32,81,27,263,28,1*7D\r\n$GLGSV,2,1,05,77,37,182,15,78,65,276,27,79,22,328,26,81,27,263,17,3*73\r\n$GLGSV,2,2,05,88,61,328,17,3*47\r\n$GLGSV,1,1,04,65,11,116,,71,06,027,,72,16,073,,87,39,031,,0*7C\r\n$GAGSV,1,1,00,0*74\r\n$GBGSV,1,1,00,0*77\r\n$GNGLL,3717.4904121,N,12708.8654426,E,065757.00,A,A*7B\r\n$GNRMC,065758.00,A,3717.4902805,N,12708.8658821,E,0.076,,190421,,,A,V*17\r\n$GNVTG,,T,,M,0.076,N,0.142,K,A*3B\r\n$GNGGA,065758.00,3717.4902805,N,12708.8658821,E,1,07,2.16,186.917,M,18.960,M,,*4B\r\n$GNGSA,A,3,14,28,30,07,,,,,,,,,3.09,2.16,2.21,1*04\r\n$GNGSA,A,3,79,88,81,,,,,,,,,,3.09,2.16,2.21,2*0B\r\n$GNGSA,A,3,,,,,,,,,,,,,3.09,2.16,2.21,3*0D\r\n$GNGSA,A,3,,,,,,,,,,,,,3.09,2.16,2.21,4*0A\r\n$GPGSV,2,1,06,07,17,202,09,14,56,311,29,19,08,276,09,28,47,315,25,1*64\r\n$GPGSV,2,2,06,30,33,243,32,41,27,238,27,1*69\r\n$GPGSV,1,1,02,14,56,311,16,30,33,243,24,6*63\r\n$GPGSV,1,1,01,08,29,078,,0*58\r\n$GLGSV,1,1,02,79,22,328,32,81,27,263,28,1*7D\r\n$GLGSV,2,1,05,77,37,182,14,78,65,276,27,79,22,328,26,81,27,263,18,3*7D\r\n$GLGSV,2,2,05,88,61,328,18,3*48\r\n$GLGSV,1,1,04,65,11,116,,71,06,027,,72,16,073,,87,39,031,,0*7C\r\n$GAGSV,1,1,00,0*74\r\n$GBGSV,1,1,00,0*77\r\n$GNGLL,3717.4902805,N,12708.8658821,E,065758.00,A,A*7A\r\n$GNRMC,065759.00,A,3717.4902227,N,12708.8660382,E,0.057,,190421,,,A,V*16\r\n$GNVTG,,T,,M,0.057,N,0.105,K,A*3B\r\n$GNGGA,065759.00,3717.4902227,N,12708.8660382,E,1,06,2.16,186.835,M,18.960,M,,*49\r\n$GNGSA,A,3,14,28,30,07,,,,,,,,,3.09,2.16,2.21,1*04\r\n$GNGSA,A,3,79,88,81,,,,,,,,,,3.09,2.16,2.21,2*0B\r\n$GNGSA,A,3,,,,,,,,,,,,,3.09,2.16,2.21,3*0D\r\n$GNGSA,A,3,,,,,,,,,,,,,3.09,2.16,2.21,4*0A\r\n$GPGSV,2,1,06,07,17,202,12,14,56,311,29,19,08,276,08,28,47,315,25,1*6F\r\n$GPGSV,2,2,06,30,33,243,33,41,27,238,27,1*68\r\n$GPGSV,1,1,02,14,56,311,14,30,33,243,24,6*61\r\n$GPGSV,1,1,01,08,29,078,,0*58\r\n$GLGSV,1,1,02,79,22,328,32,81,27,263,28,1*7D\r\n$GLGSV,2,1,05,77,37,182,13,78,65,276,27,79,22,328,26,81,27,263,17,3*75\r\n$GLGSV,2,2,05,88,61,328,18,3*48\r\n$GLGSV,1,1,04,65,11,116,,71,06,027,,72,16,073,,87,39,031,,0*7C\r\n$GAGSV,1,1,00,0*74\r\n$GBGSV,1,1,00,0*77\r\n$GNGLL,3717.4902227,N,12708.8660382,E,065759.00,A,A*78\r\n$GNRMC,065800.00,A,3717.4901343,N,12708.8662956,E,0.032,,190421,,,A,V*17\r\n$GNVTG,,T,,M,0.032,N,0.059,K,A*30\r\n$GNGGA,065800.00,3717.4901343,N,12708.8662956,E,1,06,2.16,186.736,M,18.960,M,,*47\r\n$GNGSA,A,3,14,28,30,07,,,,,,,,,3.09,2.16,2.21,1*04\r\n$GNGSA,A,3,79,88,81,,,,,,,,,,3.09,2.16,2.21,2*0B\r\n$GNGSA,A,3,,,,,,,,,,,,,3.09,2.16,2.21,3*0D\r\n$GNGSA,A,3,,,,,,,,,,,,,3.09,2.16,2.21,4*0A\r\n$GPGSV,2,1,06,07,17,202,11,14,56,311,29,19,08,277,10,28,47,315,25,1*64\r\n$GPGSV,2,2,06,30,33,243,33,41,27,238,27,1*68\r\n$GPGSV,1,1,02,14,56,311,14,30,33,243,24,6*61\r\n$GPGSV,1,1,01,08,29,078,,0*58\r\n$GLGSV,1,1,03,78,65,276,27,79,22,328,32,81,27,263,29,1*47\r\n$GLGSV,2,1,05,77,37,182,12,78,65,276,27,79,22,328,27,81,27,263,15,3*77\r\n$GLGSV,2,2,05,88,61,328,18,3*48\r\n$GLGSV,1,1,04,65,11,116,,71,06,027,,72,16,073,,87,39,031,,0*7C\r\n$GAGSV,1,1,00,0*74\r\n$GBGSV,1,1,00,0*77\r\n$GNGLL,3717.4901343,N,12708.8662956,E,065800.00,A,A*7A\r\n$GNRMC,065801.00,A,3717.4899728,N,12708.8668956,E,0.091,,190421,,,A,V*1C\r\n$GNVTG,,T,,M,0.091,N,0.168,K,A*3A\r\n$GNGGA,065801.00,3717.4899728,N,12708.8668956,E,1,06,2.16,186.427,M,18.960,M,,*46\r\n$GNGSA,A,3,14,28,30,07,,,,,,,,,3.09,2.16,2.21,1*04\r\n$GNGSA,A,3,79,88,81,,,,,,,,,,3.09,2.16,2.21,2*0B\r\n$GNGSA,A,3,,,,,,,,,,,,,3.09,2.16,2.21,3*0D\r\n$GNGSA,A,3,,,,,,,,,,,,,3.09,2.16,2.21,4*0A\r\n$GPGSV,2,1,06,07,17,202,10,14,56,311,29,19,08,277,09,28,47,315,25,1*6D\r\n$GPGSV,2,2,06,30,33,243,33,41,27,238,27,1*68\r\n$GPGSV,1,1,02,14,56,311,15,30,33,243,24,6*60\r\n$GPGSV,1,1,01,08,29,078,,0*58\r\n$GLGSV,1,1,03,78,65,276,27,79,22,328,32,81,27,263,29,1*47\r\n$GLGSV,1,1,04,77,37,182,13,78,65,276,27,79,22,328,26,88,61,328,17,3*72\r\n$GLGSV,1,1,04,65,11,116,,71,06,027,,72,16,073,,87,39,031,,0*7C\r\n$GAGSV,1,1,00,0*74\r\n$GBGSV,1,1,00,0*77\r\n$GNGLL,3717.4899728,N,12708.8668956,E,065801.00,A,A*78\r\n$GNRMC,065802.00,A,3717.4898986,N,12708.8669594,E,0.109,,190421,,,A,V*17\r\n$GNVTG,,T,,M,0.109,N,0.201,K,A*36\r\n$GNGGA,065802.00,3717.4898986,N,12708.8669594,E,1,07,2.16,186.352,M,18.960,M,,*49\r\n$GNGSA,A,3,14,28,30,07,,,,,,,,,3.09,2.16,2.21,1*04\r\n$GNGSA,A,3,79,88,81,,,,,,,,,,3.09,2.16,2.21,2*0B\r\n$GNGSA,A,3,,,,,,,,,,,,,3.09,2.16,2.21,3*0D\r\n$GNGSA,A,3,,,,,,,,,,,,,3.09,2.16,2.21,4*0A\r\n$GPGSV,2,1,06,07,17,202,11,14,56,311,29,19,08,277,08,28,47,315,24,1*6C\r\n$GPGSV,2,2,06,30,33,243,33,41,27,238,27,1*68\r\n$GPGSV,1,1,02,14,56,311,15,30,33,243,25,6*61\r\n$GPGSV,1,1,01,08,29,078,,0*58\r\n$GLGSV,1,1,04,78,65,276,27,79,22,328,32,81,27,263,29,88,61,328,31,1*7C\r\n$GLGSV,1,1,04,77,37,182,12,78,65,276,27,79,22,328,27,88,61,328,16,3*73\r\n$GLGSV,1,1,04,65,11,116,,71,06,027,,72,16,073,,87,39,031,,0*7C\r\n$GAGSV,1,1,00,0*74\r\n$GBGSV,1,1,00,0*77\r\n$GNGLL,3717.4898986,N,12708.8669594,E,065802.00,A,A*73\r\n$GNRMC,065803.00,A,3717.4898561,N,12708.8668168,E,0.117,,190421,,,A,V*1A\r\n$GNVTG,,T,,M,0.117,N,0.217,K,A*3E\r\n$GNGGA,065803.00,3717.4898561,N,12708.8668168,E,1,06,2.93,186.280,M,18.960,M,,*49\r\n$GNGSA,A,3,14,28,30,07,,,,,,,,,3.67,2.93,2.21,1*01\r\n$GNGSA,A,3,79,88,,,,,,,,,,,3.67,2.93,2.21,2*07\r\n$GNGSA,A,3,,,,,,,,,,,,,3.67,2.93,2.21,3*08\r\n$GNGSA,A,3,,,,,,,,,,,,,3.67,2.93,2.21,4*0F\r\n$GPGSV,2,1,06,07,17,202,12,14,56,311,29,19,08,277,13,28,47,315,24,1*65\r\n$GPGSV,2,2,06,30,33,243,33,41,27,238,27,1*68\r\n$GPGSV,1,1,02,14,56,311,15,30,33,243,25,6*61\r\n$GPGSV,1,1,01,08,29,078,,0*58\r\n$GLGSV,1,1,03,78,65,276,27,79,22,328,32,88,61,328,31,1*4B\r\n$GLGSV,1,1,04,77,37,182,11,78,65,276,27,79,22,328,27,88,61,328,16,3*70\r\n$GLGSV,2,1,05,65,11,116,,71,06,027,,72,16,073,,81,27,263,,0*72\r\n$GLGSV,2,2,05,81,27,263,,0*47\r\n$GAGSV,1,1,00,0*74\r\n$GBGSV,1,1,00,0*77\r\n$GNGLL,3717.4898561,N,12708.8668168,E,065803.00,A,A*71\r\n$GNRMC,065804.00,A,3717.4897196,N,12708.8670531,E,0.050,,190421,,,A,V*1D\r\n$GNVTG,,T,,M,0.050,N,0.093,K,A*32\r\n$GNGGA,065804.00,3717.4897196,N,12708.8670531,E,1,06,2.93,185.906,M,18.960,M,,*4A\r\n$GNGSA,A,3,14,28,30,07,,,,,,,,,3.67,2.93,2.21,1*01\r\n$GNGSA,A,3,79,88,,,,,,,,,,,3.67,2.93,2.21,2*07\r\n$GNGSA,A,3,,,,,,,,,,,,,3.67,2.93,2.21,3*08\r\n$GNGSA,A,3,,,,,,,,,,,,,3.67,2.93,2.21,4*0F\r\n$GPGSV,2,1,06,07,17,202,09,14,56,311,29,19,08,277,08,28,47,315,24,1*65\r\n$GPGSV,2,2,06,30,33,242,33,41,27,238,27,1*69\r\n$GPGSV,1,1,02,14,56,311,16,30,33,242,25,6*63\r\n$GPGSV,1,1,01,08,29,078,,0*58\r\n$GLGSV,1,1,03,78,65,276,28,79,22,328,32,88,61,328,30,1*45\r\n$GLGSV,1,1,04,77,37,182,09,78,65,276,27,79,22,328,27,88,61,328,16,3*79\r\n$GLGSV,2,1,05,65,11,116,,71,06,027,,72,16,073,,81,27,263,,0*72\r\n$GLGSV,2,2,05,81,27,263,,0*47\r\n$GAGSV,1,1,00,0*74\r\n$GBGSV,1,1,00,0*77\r\n$GNGLL,3717.4897196,N,12708.8670531,E,065804.00,A,A*74\r\n$GNRMC,065805.00,A,3717.4896659,N,12708.8670334,E,0.078,,190421,,,A,V*10\r\n$GNVTG,,T,,M,0.078,N,0.144,K,A*33\r\n$GNGGA,065805.00,3717.4896659,N,12708.8670334,E,1,06,2.93,185.791,M,18.960,M,,*4D\r\n$GNGSA,A,3,14,28,30,07,,,,,,,,,3.67,2.93,2.21,1*01\r\n$GNGSA,A,3,79,88,,,,,,,,,,,3.67,2.93,2.21,2*07\r\n$GNGSA,A,3,,,,,,,,,,,,,3.67,2.93,2.21,3*08\r\n$GNGSA,A,3,,,,,,,,,,,,,3.67,2.93,2.21,4*0F\r\n$GPGSV,2,1,06,07,17,202,10,14,56,311,29,19,08,277,11,28,47,315,24,1*65\r\n$GPGSV,2,2,06,30,33,242,33,41,27,238,27,1*69\r\n$GPGSV,1,1,02,14,56,311,16,30,33,242,25,6*63\r\n$GPGSV,1,1,01,08,29,078,,0*58\r\n$GLGSV,1,1,03,78,65,276,28,79,22,328,32,88,61,328,30,1*45\r\n$GLGSV,1,1,04,77,37,182,08,78,65,276,27,79,22,328,27,88,61,328,17,3*79\r\n$GLGSV,2,1,05,65,11,116,,71,06,027,,72,16,073,,81,27,263,,0*72\r\n$GLGSV,2,2,05,81,27,263,,0*47\r\n$GAGSV,1,1,00,0*74\r\n$GBGSV,1,1,00,0*77\r\n$GNGLL,3717.4896659,N,12708.8670334,E,065805.00,A,A*73\r\n$GNRMC,065806.00,A,3717.4895805,N,12708.8672442,E,0.234,,190421,,,A,V*19\r\n$GNVTG,,T,,M,0.234,N,0.434,K,A*3B\r\n$GNGGA,065806.00,3717.4895805,N,12708.8672442,E,1,06,2.93,185.635,M,18.960,M,,*41\r\n$GNGSA,A,3,14,28,30,07,,,,,,,,,3.67,2.93,2.21,1*01\r\n$GNGSA,A,3,79,88,,,,,,,,,,,3.67,2.93,2.21,2*07\r\n$GNGSA,A,3,,,,,,,,,,,,,3.67,2.93,2.21,3*08\r\n$GNGSA,A,3,,,,,,,,,,,,,3.67,2.93,2.21,4*0F\r\n$GPGSV,2,1,06,07,17,202,10,14,56,311,29,19,08,277,07,28,47,315,24,1*62\r\n$GPGSV,2,2,06,30,33,242,33,41,27,238,27,1*69\r\n$GPGSV,1,1,02,14,56,311,16,30,33,242,25,6*63\r\n$GPGSV,1,1,01,08,29,078,,0*58\r\n$GLGSV,1,1,03,78,65,276,28,79,22,328,32,88,61,328,30,1*45\r\n$GLGSV,1,1,03,78,65,276,27,79,22,328,27,88,61,328,17,3*49\r\n$GLGSV,2,1,06,65,11,116,,71,06,027,,72,16,073,,77,37,182,,0*75\r\n$GLGSV,2,2,06,77,37,182,,81,27,263,,0*7B\r\n$GAGSV,1,1,00,0*74\r\n$GBGSV,1,1,00,0*77\r\n$GNGLL,3717.4895805,N,12708.8672442,E,065806.00,A,A*70\r\n$GNRMC,065807.00,A,3717.4894495,N,12708.8675213,E,0.183,,190421,,,A,V*16\r\n$GNVTG,,T,,M,0.183,N,0.339,K,A*3E\r\n$GNGGA,065807.00,3717.4894495,N,12708.8675213,E,1,06,2.93,185.167,M,18.960,M,,*41\r\n$GNGSA,A,3,14,28,30,07,,,,,,,,,3.67,2.93,2.21,1*01\r\n$GNGSA,A,3,79,88,,,,,,,,,,,3.67,2.93,2.21,2*07\r\n$GNGSA,A,3,,,,,,,,,,,,,3.67,2.93,2.21,3*08\r\n$GNGSA,A,3,,,,,,,,,,,,,3.67,2.93,2.21,4*0F\r\n$GPGSV,2,1,06,07,17,202,10,14,56,311,29,19,08,277,11,28,47,315,24,1*65\r\n$GPGSV,2,2,06,30,33,242,33,41,27,238,27,1*69\r\n$GPGSV,1,1,02,14,56,311,16,30,33,242,25,6*63\r\n$GPGSV,1,1,01,08,29,078,,0*58\r\n$GLGSV,1,1,03,78,65,276,27,79,22,328,32,88,61,328,30,1*4A\r\n$GLGSV,1,1,03,78,65,276,27,79,22,328,27,88,61,328,17,3*49\r\n$GLGSV,2,1,06,65,11,116,,71,06,027,,72,16,073,,77,37,182,,0*75\r\n$GLGSV,2,2,06,77,37,182,,81,27,263,,0*7B\r\n$GAGSV,1,1,00,0*74\r\n$GBGSV,1,1,00,0*77\r\n$GNGLL,3717.4894495,N,12708.8675213,E,065807.00,A,A*70\r\n$GNRMC,065808.00,A,3717.4893143,N,12708.8679413,E,0.330,,190421,,,A,V*10\r\n$GNVTG,,T,,M,0.330,N,0.610,K,A*3A\r\n$GNGGA,065808.00,3717.4893143,N,12708.8679413,E,1,06,2.16,184.948,M,18.960,M,,*44\r\n$GNGSA,A,3,14,28,30,07,,,,,,,,,3.09,2.16,2.21,1*04\r\n$GNGSA,A,3,79,88,81,,,,,,,,,,3.09,2.16,2.21,2*0B\r\n$GNGSA,A,3,,,,,,,,,,,,,3.09,2.16,2.21,3*0D\r\n$GNGSA,A,3,,,,,,,,,,,,,3.09,2.16,2.21,4*0A\r\n$GPGSV,2,1,05,07,17,202,10,14,56,311,29,19,08,277,11,28,47,315,24,1*66\r\n$GPGSV,2,2,05,30,33,242,33,1*56\r\n$GPGSV,1,1,02,14,56,311,15,30,33,242,25,6*60\r\n$GPGSV,1,1,01,08,29,078,,0*58\r\n$GLGSV,1,1,04,78,65,276,28,79,22,328,33,81,27,263,29,88,61,328,30,1*73\r\n$GLGSV,1,1,03,78,65,276,27,79,22,328,27,88,61,328,16,3*48\r\n$GLGSV,2,1,05,65,11,116,,71,06,027,,72,16,073,,77,37,182,,0*76\r\n$GLGSV,2,2,05,77,37,182,,0*43\r\n$GAGSV,1,1,00,0*74\r\n$GBGSV,1,1,00,0*77\r\n$GNGLL,3717.4893143,N,12708.8679413,E,065808.00,A,A*7C\r\n$GNRMC,065809.00,A,3717.4892254,N,12708.8681747,E,0.266,,190421,,,A,V*12\r\n$GNVTG,,T,,M,0.266,N,0.492,K,A*30\r\n$GNGGA,065809.00,3717.4892254,N,12708.8681747,E,1,06,2.15,184.837,M,18.960,M,,*4E\r\n$GNGSA,A,3,14,28,30,07,,,,,,,,,3.09,2.15,2.21,1*07\r\n$GNGSA,A,3,79,88,81,,,,,,,,,,3.09,2.15,2.21,2*08\r\n$GNGSA,A,3,,,,,,,,,,,,,3.09,2.15,2.21,3*0E\r\n$GNGSA,A,3,,,,,,,,,,,,,3.09,2.15,2.21,4*09\r\n$GPGSV,2,1,05,07,17,202,10,14,56,311,29,19,08,277,11,28,47,315,23,1*61\r\n$GPGSV,2,2,05,30,33,242,33,1*56\r\n$GPGSV,1,1,02,14,56,311,15,30,33,242,25,6*60\r\n$GPGSV,1,1,01,08,29,078,,0*58\r\n$GLGSV,1,1,04,78,65,276,28,79,22,328,33,81,27,263,29,88,61,328,30,1*73\r\n$GLGSV,1,1,03,78,65,276,27,79,22,328,27,88,61,328,16,3*48\r\n$GLGSV,2,1,05,65,11,116,,71,06,027,,72,16,073,,77,37,182,,0*76\r\n$GLGSV,2,2,05,77,37,182,,0*43\r\n$GAGSV,1,1,00,0*74\r\n$GBGSV,1,1,00,0*77\r\n$GNGLL,3717.4892254,N,12708.8681747,E,065809.00,A,A*7C\r\n$GNRMC,065810.00,A,3717.4892310,N,12708.8678799,E,0.081,,190421,,,A,V*15\r\n$GNVTG,,T,,M,0.081,N,0.150,K,A*30\r\n$GNGGA,065810.00,3717.4892310,N,12708.8678799,E,1,05,8.19,184.894,M,18.960,M,,*4E\r\n$GNGSA,A,3,14,28,30,,,,,,,,,,9.58,8.19,4.97,1*03\r\n$GNGSA,A,3,79,88,,,,,,,,,,,9.58,8.19,4.97,2*02\r\n$GNGSA,A,3,,,,,,,,,,,,,9.58,8.19,4.97,3*0D\r\n$GNGSA,A,3,,,,,,,,,,,,,9.58,8.19,4.97,4*0A\r\n$GPGSV,2,1,05,07,17,202,04,14,56,311,29,19,08,277,04,28,47,315,22,1*61\r\n$GPGSV,2,2,05,30,33,242,33,1*56\r\n$GPGSV,1,1,02,14,56,311,16,30,33,242,26,6*60\r\n$GPGSV,1,1,01,08,29,078,,0*58\r\n$GLGSV,1,1,03,78,65,276,28,79,22,328,33,88,61,328,30,1*44\r\n$GLGSV,1,1,03,78,65,276,27,79,22,328,27,88,61,328,16,3*48\r\n$GLGSV,2,1,06,65,11,116,,71,06,027,,72,16,073,,77,37,182,,0*75\r\n$GLGSV,2,2,06,77,37,182,,81,27,263,,0*7B\r\n$GAGSV,1,1,00,0*74\r\n$GBGSV,1,1,00,0*77\r\n$GNGLL,3717.4892310,N,12708.8678799,E,065810.00,A,A*70\r\n$GNRMC,065811.00,A,3717.4891810,N,12708.8679408,E,0.114,,190421,,,A,V*1B\r\n$GNVTG,,T,,M,0.114,N,0.212,K,A*38\r\n$GNGGA,065811.00,3717.4891810,N,12708.8679408,E,1,05,5.94,184.866,M,18.960,M,,*48\r\n$GNGSA,A,3,14,28,30,,,,,,,,,,7.38,5.94,4.38,1*06\r\n$GNGSA,A,3,79,88,81,,,,,,,,,,7.38,5.94,4.38,2*0E\r\n$GNGSA,A,3,,,,,,,,,,,,,7.38,5.94,4.38,3*08\r\n$GNGSA,A,3,,,,,,,,,,,,,7.38,5.94,4.38,4*0F\r\n$GPGSV,2,1,05,07,17,202,06,14,56,311,29,19,08,277,07,28,47,315,22,1*60\r\n$GPGSV,2,2,05,30,33,242,33,1*56\r\n$GPGSV,1,1,02,14,56,311,16,30,33,242,26,6*60\r\n$GPGSV,1,1,01,08,29,078,,0*58\r\n$GLGSV,1,1,03,78,65,276,28,79,22,328,33,81,27,263,30,1*41\r\n$GLGSV,1,1,03,78,65,276,28,79,22,328,27,88,61,328,17,3*46\r\n$GLGSV,2,1,05,65,11,116,,71,06,027,,72,16,073,,77,37,182,,0*76\r\n$GLGSV,2,2,05,77,37,182,,0*43\r\n$GAGSV,1,1,00,0*74\r\n$GBGSV,1,1,00,0*77\r\n$GNGLL,3717.4891810,N,12708.8679408,E,065811.00,A,A*73\r\n$GNRMC,065812.00,A,3717.4891217,N,12708.8680135,E,0.074,,190421,,,A,V*1F\r\n$GNVTG,,T,,M,0.074,N,0.137,K,A*3B\r\n$GNGGA,065812.00,3717.4891217,N,12708.8680135,E,1,04,5.94,184.801,M,18.960,M,,*4B\r\n$GNGSA,A,3,14,28,30,,,,,,,,,,7.38,5.94,4.38,1*06\r\n$GNGSA,A,3,79,88,81,,,,,,,,,,7.38,5.94,4.38,2*0E\r\n$GNGSA,A,3,,,,,,,,,,,,,7.38,5.94,4.38,3*08\r\n$GNGSA,A,3,,,,,,,,,,,,,7.38,5.94,4.38,4*0F\r\n$GPGSV,2,1,05,07,17,202,08,14,56,311,29,19,08,277,08,28,47,315,22,1*61\r\n$GPGSV,2,2,05,30,33,242,33,1*56\r\n$GPGSV,1,1,02,14,56,311,16,30,33,242,26,6*60\r\n$GPGSV,1,1,01,08,29,078,,0*58\r\n$GLGSV,1,1,03,78,65,276,28,79,22,328,33,81,27,263,29,1*49\r\n$GLGSV,1,1,03,78,65,276,27,79,22,328,27,88,61,328,17,3*49\r\n$GLGSV,2,1,05,65,11,116,,71,06,027,,72,16,073,,77,37,182,,0*76\r\n$GLGSV,2,2,05,77,37,182,,0*43\r\n$GAGSV,1,1,00,0*74\r\n$GBGSV,1,1,00,0*77\r\n$GNGLL,3717.4891217,N,12708.8680135,E,065812.00,A,A*70\r\n$GNRMC,065813.00,A,3717.4889244,N,12708.8686433,E,0.036,,190421,,,A,V*12\r\n$GNVTG,,T,,M,0.036,N,0.066,K,A*38\r\n$GNGGA,065813.00,3717.4889244,N,12708.8686433,E,1,05,2.15,184.299,M,18.960,M,,*44\r\n$GNGSA,A,3,14,28,30,07,,,,,,,,,3.09,2.15,2.21,1*07\r\n$GNGSA,A,3,79,88,81,,,,,,,,,,3.09,2.15,2.21,2*08\r\n$GNGSA,A,3,,,,,,,,,,,,,3.09,2.15,2.21,3*0E\r\n$GNGSA,A,3,,,,,,,,,,,,,3.09,2.15,2.21,4*09\r\n$GPGSV,2,1,05,07,17,202,13,14,56,311,28,19,08,277,08,28,47,315,22,1*6A\r\n$GPGSV,2,2,05,30,33,242,33,1*56\r\n$GPGSV,1,1,02,14,56,311,16,30,33,242,26,6*60\r\n$GPGSV,1,1,01,08,29,078,,0*58\r\n$GLGSV,1,1,03,78,65,276,28,79,22,328,34,81,27,263,28,1*4F\r\n$GLGSV,1,1,04,65,11,116,19,78,65,276,27,79,22,328,27,88,61,328,19,3*7D\r\n$GLGSV,1,1,04,71,06,027,,72,16,073,,77,37,182,,87,39,031,,0*76\r\n$GAGSV,1,1,00,0*74\r\n$GBGSV,1,1,00,0*77\r\n$GNGLL,3717.4889244,N,12708.8686433,E,065813.00,A,A*7B\r\n$GNRMC,065814.00,A,3717.4888251,N,12708.8690068,E,0.088,,190421,,,A,V*18\r\n$GNVTG,,T,,M,0.088,N,0.163,K,A*39\r\n$GNGGA,065814.00,3717.4888251,N,12708.8690068,E,1,06,2.15,184.235,M,18.960,M,,*4E\r\n$GNGSA,A,3,14,28,30,07,,,,,,,,,3.09,2.15,2.21,1*07\r\n$GNGSA,A,3,79,88,81,,,,,,,,,,3.09,2.15,2.21,2*08\r\n$GNGSA,A,3,,,,,,,,,,,,,3.09,2.15,2.21,3*0E\r\n$GNGSA,A,3,,,,,,,,,,,,,3.09,2.15,2.21,4*09\r\n$GPGSV,2,1,05,07,17,202,08,14,56,311,29,19,08,277,10,28,47,315,22,1*68\r\n$GPGSV,2,2,05,30,33,242,33,1*56\r\n$GPGSV,1,1,02,14,56,311,16,30,33,242,26,6*60\r\n$GPGSV,1,1,02,08,29,078,,17,31,290,,0*64\r\n$GLGSV,1,1,03,78,65,276,28,79,22,328,33,81,27,263,28,1*48\r\n$GLGSV,1,1,04,65,11,116,18,78,65,276,28,79,22,328,27,88,61,328,19,3*73\r\n$GLGSV,1,1,04,71,06,027,,72,16,073,,77,37,182,,87,39,031,,0*76\r\n$GAGSV,1,1,00,0*74\r\n$GBGSV,1,1,00,0*77\r\n$GNGLL,3717.4888251,N,12708.8690068,E,065814.00,A,A*74\r\n$GNRMC,065815.00,A,3717.4887980,N,12708.8690028,E,0.032,,190421,,,A,V*14\r\n$GNVTG,,T,,M,0.032,N,0.059,K,A*30\r\n$GNGGA,065815.00,3717.4887980,N,12708.8690028,E,1,05,2.15,184.235,M,18.960,M,,*40\r\n$GNGSA,A,3,14,28,30,07,,,,,,,,,3.09,2.15,2.21,1*07\r\n$GNGSA,A,3,79,88,81,,,,,,,,,,3.09,2.15,2.21,2*08\r\n$GNGSA,A,3,,,,,,,,,,,,,3.09,2.15,2.21,3*0E\r\n$GNGSA,A,3,,,,,,,,,,,,,3.09,2.15,2.21,4*09\r\n$GPGSV,2,1,05,07,17,202,10,14,56,311,29,19,08,277,09,28,47,315,22,1*69\r\n$GPGSV,2,2,05,30,33,242,33,1*56\r\n$GPGSV,1,1,02,14,56,311,16,30,33,242,26,6*60\r\n$GPGSV,1,1,02,08,29,078,,17,31,290,,0*64\r\n$GLGSV,1,1,03,78,65,276,28,79,22,328,33,81,27,263,28,1*48\r\n$GLGSV,1,1,04,65,11,116,17,78,65,276,28,79,22,328,27,88,61,328,18,3*7D\r\n$GLGSV,1,1,04,71,06,027,,72,16,073,,77,37,182,,87,39,031,,0*76\r\n$GAGSV,1,1,00,0*74\r\n$GBGSV,1,1,00,0*77\r\n$GNGLL,3717.4887980,N,12708.8690028,E,065815.00,A,A*79\r\n$GNRMC,065816.00,A,3717.4886010,N,12708.8696115,E,0.037,,190421,,,A,V*1A\r\n$GNVTG,,T,,M,0.037,N,0.068,K,A*37\r\n$GNGGA,065816.00,3717.4886010,N,12708.8696115,E,1,05,2.93,183.723,M,18.960,M,,*40\r\n$GNGSA,A,3,14,28,30,07,,,,,,,,,3.67,2.93,2.21,1*01\r\n$GNGSA,A,3,79,88,,,,,,,,,,,3.67,2.93,2.21,2*07\r\n$GNGSA,A,3,,,,,,,,,,,,,3.67,2.93,2.21,3*08\r\n$GNGSA,A,3,,,,,,,,,,,,,3.67,2.93,2.21,4*0F\r\n$GPGSV,2,1,05,07,17,202,09,14,56,311,29,19,08,277,11,28,47,315,23,1*69\r\n$GPGSV,2,2,05,30,33,242,32,1*57\r\n$GPGSV,1,1,02,14,56,311,16,30,33,242,26,6*60\r\n$GPGSV,1,1,02,08,29,078,,17,31,290,,0*64\r\n$GLGSV,1,1,02,78,65,276,29,79,22,328,33,1*79\r\n$GLGSV,1,1,04,65,11,116,16,78,65,276,28,79,22,328,27,88,61,328,18,3*7C\r\n$GLGSV,2,1,05,71,06,027,,72,16,073,,77,37,182,,81,27,263,,0*78\r\n$GLGSV,2,2,05,81,27,263,,0*47\r\n$GAGSV,1,1,00,0*74\r\n$GBGSV,1,1,00,0*77\r\n$GNGLL,3717.4886010,N,12708.8696115,E,065816.00,A,A*72\r\n$GNRMC,065817.00,A,3717.4885963,N,12708.8695202,E,0.077,,190421,,,A,V*17\r\n$GNVTG,,T,,M,0.077,N,0.142,K,A*3A\r\n$GNGGA,065817.00,3717.4885963,N,12708.8695202,E,1,06,2.93,183.778,M,18.960,M,,*44\r\n$GNGSA,A,3,14,28,30,07,,,,,,,,,3.67,2.93,2.21,1*01\r\n$GNGSA,A,3,79,88,,,,,,,,,,,3.67,2.93,2.21,2*07\r\n$GNGSA,A,3,,,,,,,,,,,,,3.67,2.93,2.21,3*08\r\n$GNGSA,A,3,,,,,,,,,,,,,3.67,2.93,2.21,4*0F\r\n$GPGSV,2,1,05,07,17,202,13,14,56,311,29,19,08,277,07,28,47,315,23,1*65\r\n$GPGSV,2,2,05,30,33,242,32,1*57\r\n$GPGSV,1,1,02,14,56,311,16,30,33,242,25,6*63\r\n$GPGSV,1,1,02,08,29,078,,17,31,290,,0*64\r\n$GLGSV,1,1,03,78,65,276,29,79,22,328,33,81,27,263,28,1*49\r\n$GLGSV,1,1,04,65,11,116,16,78,65,276,28,79,22,328,27,88,61,328,19,3*7D\r\n$GLGSV,1,1,04,71,06,027,,72,16,073,,77,37,182,,87,39,031,,0*76\r\n$GAGSV,1,1,00,0*74\r\n$GBGSV,1,1,00,0*77\r\n$GNGLL,3717.4885963,N,12708.8695202,E,065817.00,A,A*7B\r\n$GNRMC,065818.00,A,3717.4886079,N,12708.8693102,E,0.157,,190421,,,A,V*1F\r\n$GNVTG,,T,,M,0.157,N,0.291,K,A*34\r\n$GNGGA,065818.00,3717.4886079,N,12708.8693102,E,1,05,2.93,183.836,M,18.960,M,,*49\r\n$GNGSA,A,3,14,28,30,07,,,,,,,,,3.67,2.93,2.22,1*02\r\n$GNGSA,A,3,79,88,,,,,,,,,,,3.67,2.93,2.22,2*04\r\n$GNGSA,A,3,,,,,,,,,,,,,3.67,2.93,2.22,3*0B\r\n$GNGSA,A,3,,,,,,,,,,,,,3.67,2.93,2.22,4*0C\r\n$GPGSV,2,1,05,07,17,202,12,14,56,311,29,19,08,277,09,28,47,315,24,1*6D\r\n$GPGSV,2,2,05,30,33,242,32,1*57\r\n$GPGSV,1,1,02,14,56,311,17,30,33,242,25,6*62\r\n$GPGSV,1,1,02,08,29,078,,17,31,290,,0*64\r\n$GLGSV,1,1,02,78,65,276,28,79,22,328,33,1*78\r\n$GLGSV,1,1,04,65,11,116,15,78,65,276,27,79,22,328,27,88,61,328,19,3*71\r\n$GLGSV,2,1,05,71,06,027,,72,16,073,,77,37,182,,81,27,263,,0*78\r\n$GLGSV,2,2,05,81,27,263,,0*47\r\n$GAGSV,1,1,00,0*74\r\n$GBGSV,1,1,00,0*77\r\n$GNGLL,3717.4886079,N,12708.8693102,E,065818.00,A,A*70\r\n$GNRMC,065819.00,A,3717.4883329,N,12708.8703071,E,0.022,,190421,,,A,V*13\r\n$GNVTG,,T,,M,0.022,N,0.040,K,A*39\r\n$GNGGA,065819.00,3717.4883329,N,12708.8703071,E,1,05,2.93,183.375,M,18.960,M,,*4A\r\n$GNGSA,A,3,14,28,30,07,,,,,,,,,3.67,2.93,2.22,1*02\r\n$GNGSA,A,3,79,88,,,,,,,,,,,3.67,2.93,2.22,2*04\r\n$GNGSA,A,3,,,,,,,,,,,,,3.67,2.93,2.22,3*0B\r\n$GNGSA,A,3,,,,,,,,,,,,,3.67,2.93,2.22,4*0C\r\n$GPGSV,2,1,05,07,17,202,11,14,56,311,28,19,08,277,09,28,47,315,22,1*69\r\n$GPGSV,2,2,05,30,33,242,32,1*57\r\n$GPGSV,1,1,02,14,56,311,17,30,33,242,25,6*62\r\n$GPGSV,1,1,02,08,29,078,,17,31,290,,0*64\r\n$GLGSV,1,1,02,78,65,276,27,79,22,328,31,1*75\r\n$GLGSV,1,1,04,65,11,116,14,78,65,276,27,79,22,328,27,88,61,328,18,3*71\r\n$GLGSV,2,1,05,71,06,027,,72,16,073,,77,37,182,,81,27,263,,0*78\r\n$GLGSV,2,2,05,81,27,263,,0*47\r\n$GAGSV,1,1,00,0*74\r\n$GBGSV,1,1,00,0*77\r\n$GNGLL,3717.4883329,N,12708.8703071,E,065819.00,A,A*7F\r\n$GNRMC,065820.00,A,3717.4883560,N,12708.8701080,E,0.114,,190421,,,A,V*1A\r\n$GNVTG,,T,,M,0.114,N,0.212,K,A*38\r\n$GNGGA,065820.00,3717.4883560,N,12708.8701080,E,1,06,2.93,183.552,M,18.960,M,,*47\r\n$GNGSA,A,3,14,28,30,07,,,,,,,,,3.67,2.93,2.22,1*02\r\n$GNGSA,A,3,79,88,,,,,,,,,,,3.67,2.93,2.22,2*04\r\n$GNGSA,A,3,,,,,,,,,,,,,3.67,2.93,2.22,3*0B\r\n$GNGSA,A,3,,,,,,,,,,,,,3.67,2.93,2.22,4*0C\r\n$GPGSV,2,1,05,07,17,202,09,14,56,311,27,19,08,277,09,28,47,315,20,1*6D\r\n$GPGSV,2,2,05,30,33,242,31,1*54\r\n$GPGSV,1,1,02,14,56,311,16,30,33,242,24,6*62\r\n$GPGSV,1,1,02,08,29,078,,17,31,290,,0*64\r\n$GLGSV,1,1,02,78,65,276,26,79,22,328,31,1*74\r\n$GLGSV,1,1,04,65,11,116,13,78,65,276,26,79,22,328,26,88,61,328,17,3*79\r\n$GLGSV,2,1,05,71,06,027,,72,16,073,,77,37,182,,81,27,263,,0*78\r\n$GLGSV,2,2,05,81,27,263,,0*47\r\n$GAGSV,1,1,00,0*74\r\n$GBGSV,1,1,00,0*77\r\n$GNGLL,3717.4883560,N,12708.8701080,E,065820.00,A,A*72\r\n$GNRMC,065821.00,A,3717.4883945,N,12708.8698217,E,0.086,,190421,,,A,V*17\r\n$GNVTG,,T,,M,0.086,N,0.160,K,A*34\r\n$GNGGA,065821.00,3717.4883945,N,12708.8698217,E,1,05,2.93,183.704,M,18.960,M,,*42\r\n$GNGSA,A,3,14,28,30,07,,,,,,,,,3.67,2.93,2.22,1*02\r\n$GNGSA,A,3,79,88,,,,,,,,,,,3.67,2.93,2.22,2*04\r\n$GNGSA,A,3,,,,,,,,,,,,,3.67,2.93,2.22,3*0B\r\n$GNGSA,A,3,,,,,,,,,,,,,3.67,2.93,2.22,4*0C\r\n$GPGSV,2,1,05,07,17,202,13,14,56,311,26,19,08,277,10,28,47,315,20,1*6F\r\n$GPGSV,2,2,05,30,33,242,31,1*54\r\n$GPGSV,1,1,02,14,56,311,17,30,33,242,24,6*63\r\n$GPGSV,1,1,02,08,29,078,,17,31,290,,0*64\r\n$GLGSV,1,1,02,78,65,276,26,79,22,328,31,1*74\r\n$GLGSV,1,1,04,65,11,116,09,78,65,276,26,79,22,328,25,88,61,328,16,3*70\r\n$GLGSV,2,1,05,71,06,027,,72,16,073,,77,37,182,,81,27,263,,0*78\r\n$GLGSV,2,2,05,81,27,263,,0*47\r\n$GAGSV,1,1,00,0*74\r\n$GBGSV,1,1,00,0*77\r\n$GNGLL,3717.4883945,N,12708.8698217,E,065821.00,A,A*75\r\n"
  out "after sting":string="$GNGGA,065821.00,3717.4883945,N,12708.8698217,E,1,05,2.93,183.704,M,18.960,M,,*42\r\n"
  in  "정지":bool
  # "GNSS 232"
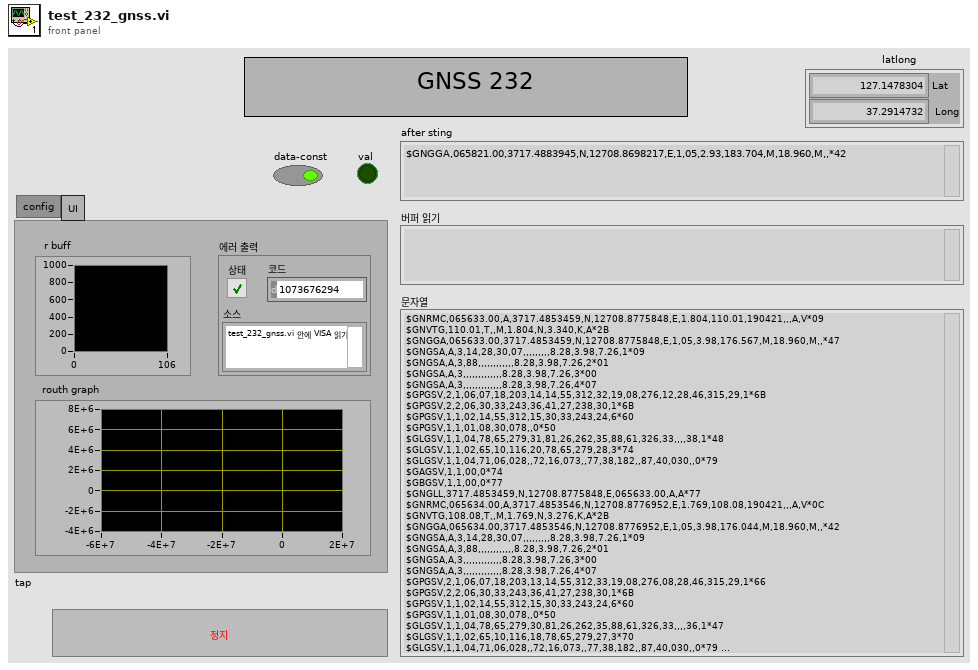
[diagram p1: front panel]
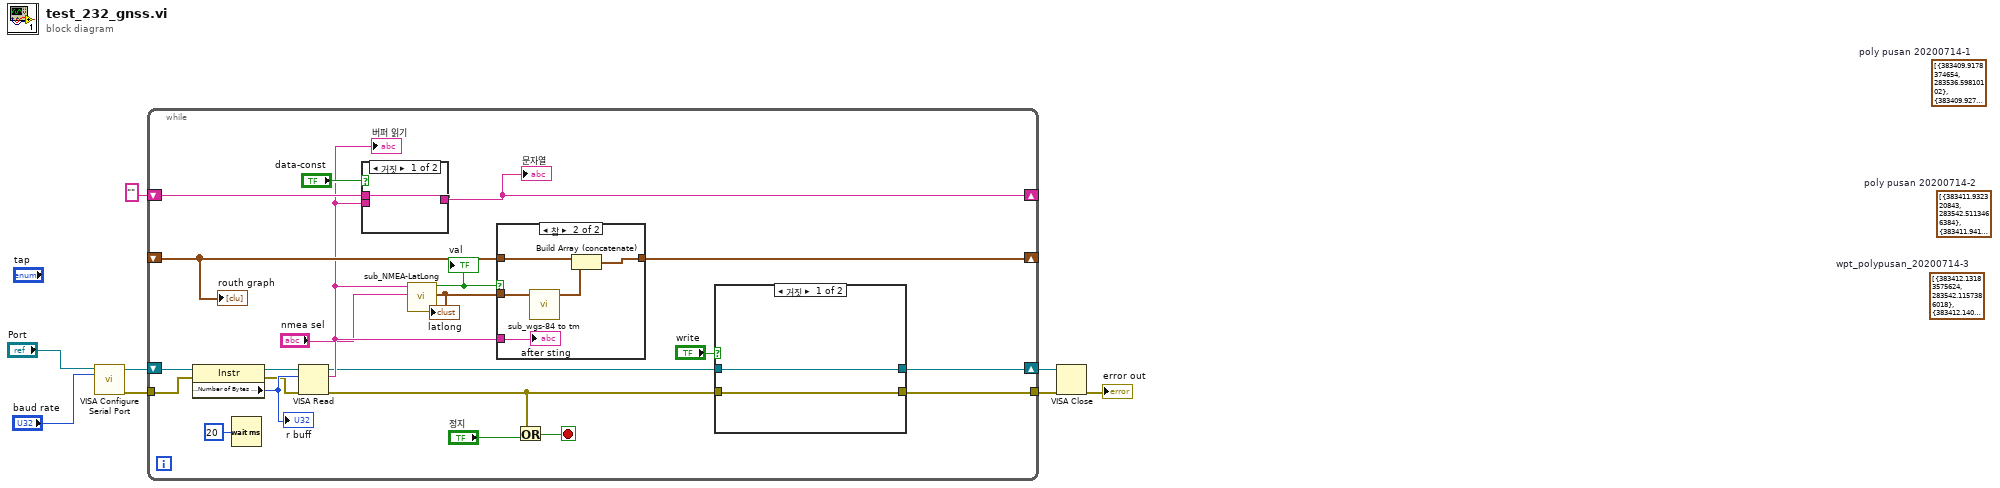
[diagram p0: block diagram]
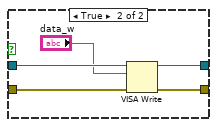
[diagram p2: hidden frame]
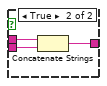
[diagram p4: hidden frame]
diagram:
  (unwired) cluster{"X":dbl, "Y":dbl}[] [{"X"=383412.13183575624, "Y"=283542.1157386018}, {"X"=383412.14072749903, "Y"=283542.12701954495}, {"X"=383412.14072749903, "Y"=283542.12701954495}, {"X"=383412.14072749903, "Y"=283542.12701954495}, {"X"=383412.1496192395, "Y"=283542.1383004872}, {"X"=383412.1496192395, "Y"=283542.1383004872}, {"X"=383412.1496192395, "Y"=283542.1383004872}, {"X"=383412.1496192395, "Y"=283542.1383004872}, {"X"=383412.1496192395, "Y"=283542.1383004872}, {"X"=383412.1496192395, "Y"=283542.1383004872}, {"X"=383412.1589596947, "Y"=283542.1273881729}, {"X"=383412.1589596947, "Y"=283542.1273881729}, {"X"=383412.1589596947, "Y"=283542.1273881729}, {"X"=383412.1680757925, "Y"=283542.12757248693}, {"X"=383412.1683001499, "Y"=283542.11647585774}, {"X"=383412.1774162478, "Y"=283542.11666017177}, {"X"=383412.1774162478, "Y"=283542.11666017177}, {"X"=383412.1774162478, "Y"=283542.11666017177}, {"X"=383412.18675670295, "Y"=283542.10574785754}, {"X"=383412.18675670295, "Y"=283542.10574785754}, {"X"=383412.1958728009, "Y"=283542.1059321715}, {"X"=383412.1960971583, "Y"=283542.0948355424}, {"X"=383412.20521325845, "Y"=283542.09501985647}, {"X"=383412.20521325845, "Y"=283542.09501985647}, {"X"=383412.214329354, "Y"=283542.09520417044}, {"X"=383412.214329354, "Y"=283542.09520417044}, {"X"=383412.2234454518, "Y"=283542.0953884845}, {"X"=383412.2234454518, "Y"=283542.0953884845}, {"X"=383412.2234454518, "Y"=283542.0953884845}, {"X"=383412.214329354, "Y"=283542.09520417044}, {"X"=383412.214329354, "Y"=283542.09520417044}, {"X"=383412.214329354, "Y"=283542.09520417044}, {"X"=383412.2145537114, "Y"=283542.08410754264}, {"X"=383412.20543761586, "Y"=283542.08392322867}, {"X"=383412.2056619733, "Y"=283542.0728265995}, {"X"=383412.19654587307, "Y"=283542.07264228543}, {"X"=383412.19677023054, "Y"=283542.0615456572}, {"X"=383412.0980636525, "Y"=283541.9818418036}, {"X"=383411.97245749284, "Y"=283541.87939175277}, {"X"=383411.8288434909, "Y"=283541.76547644875}, {"X"=383411.64966251695, "Y"=283541.6064373785}, {"X"=383411.4077906293, "Y"=283541.390624976}, {"X"=383411.0658659977, "Y"=283541.16168851225}, {"X"=383410.6785852051, "Y"=283540.920733869}, {"X"=383410.30953659787, "Y"=283540.6801478684}, {"X"=383409.922704477, "Y"=283540.41700000333}, {"X"=383409.49985664326, "Y"=283540.1309216538}, {"X"=383409.04943613, "Y"=283539.85538702144}, {"X"=383408.5990155877, "Y"=283539.5798524129}, {"X"=383408.15771112393, "Y"=283539.30450213735}, {"X"=383407.7252983808, "Y"=283539.0404328218}, {"X"=383407.30200171185, "Y"=283538.7765478377}, {"X"=383406.8962641739, "Y"=283538.54632137535}, {"X"=383406.4998670677, "Y"=283538.3051826139}, {"X"=383406.10369428596, "Y"=283538.05294724106}, {"X"=383405.6895136327, "Y"=283537.7892466443}, {"X"=383405.28444905346, "Y"=283537.52573037276}, {"X"=383404.870044003, "Y"=283537.2731264438}, {"X"=383404.4554145847, "Y"=283537.0316191623}, {"X"=383404.04100949224, "Y"=283536.77901527355}, {"X"=383403.6266043726, "Y"=283536.52641140413}, {"X"=383403.18529961235, "Y"=283536.2510613829}, {"X"=383402.7346543793, "Y"=283535.9866237099}, {"X"=383402.29312522465, "Y"=283535.72237036366}, {"X"=383401.85182039154, "Y"=283535.44702041155}, {"X"=383401.43763949943, "Y"=283535.18332001864}, {"X"=383401.0603716887, "Y"=283534.89816360164}, {"X"=383400.74758961983, "Y"=283534.58100742893}, {"X"=383400.4815097676, "Y"=283534.2092896391}, {"X"=383400.280140006, "Y"=283533.79447545746}, {"X"=383400.14348033105, "Y"=283533.33656487794}, {"X"=383400.07197944535, "Y"=283532.81336464395}, {"X"=383400.0834208813, "Y"=283532.24743661174}, {"X"=383400.18602339644, "Y"=283531.68335159513}, {"X"=383400.41512973054, "Y"=283531.17732994177}, {"X"=383400.72426198516, "Y"=283530.7728366644}, {"X"=383401.0771800759, "Y"=283530.4580379334}, {"X"=383401.45587610855, "Y"=283530.2214685208}, {"X"=383401.88792276254, "Y"=283530.0525847101}, {"X"=383402.30928290833, "Y"=283529.9611930121}, {"X"=383402.7477535631, "Y"=283529.9256530838}, {"X"=383403.16642158024, "Y"=283529.9674209622}, {"X"=383403.52904686355, "Y"=283530.07466280117}, {"X"=383403.90878262615, "Y"=283530.2377564051}, {"X"=383404.31496931607, "Y"=283530.44578945445}, {"X"=383404.7382664643, "Y"=283530.7096742769}, {"X"=383405.1704553586, "Y"=283530.9848400567}, {"X"=383405.5937524603, "Y"=283531.2487249207}, {"X"=383405.99926602206, "Y"=283531.4900479345}, {"X"=383406.3954391052, "Y"=283531.7422832877}, {"X"=383406.81828743755, "Y"=283532.02836147026}, {"X"=383407.25002750533, "Y"=283532.3257206095}, {"X"=383407.6726514358, "Y"=283532.6228954618}, {"X"=383408.0954996884, "Y"=283532.9089737058}, {"X"=383408.5456962394, "Y"=283533.19560490194}, {"X"=383408.98655230104, "Y"=283533.4931484379}, {"X"=383409.40962482896, "Y"=283533.7681301187}, {"X"=383409.81446512, "Y"=283534.0427432001}, {"X"=383410.2101892815, "Y"=283534.3171719865}, {"X"=383410.6150295247, "Y"=283534.5917851032}, {"X"=383411.02898584673, "Y"=283534.86658255244}, {"X"=383411.4431665024, "Y"=283535.1302833934}, {"X"=383411.8575714911, "Y"=283535.3828876251}, {"X"=383412.28975995193, "Y"=283535.65805376216}, {"X"=383412.7401805953, "Y"=283535.9335885495}, {"X"=383413.1632529006, "Y"=283536.20857041556}, {"X"=383413.5772090795, "Y"=283536.48336798773}, {"X"=383414.00028133026, "Y"=283536.75834989623}, {"X"=383414.47737710393, "Y"=283537.0677276065}, {"X"=383414.95424848073, "Y"=283537.38820197195}, {"X"=383415.36775582953, "Y"=283537.6851928882}, {"X"=383415.72634217737, "Y"=283537.9921745477}, {"X"=383416.0202183364, "Y"=283538.3422525123}, {"X"=383416.2673921541, "Y"=283538.74689204094}, {"X"=383416.4496314275, "Y"=283539.2057244933}, {"X"=383416.54870396585, "Y"=283539.7183812282}, {"X"=383416.5472750222, "Y"=283540.24010709027}, {"X"=383416.48270647053, "Y"=283540.7272528411}, {"X"=383416.3369904831, "Y"=283541.1683532132}, {"X"=383416.1096783414, "Y"=283541.5856014671}, {"X"=383415.8103348771, "Y"=283541.95698867145}, {"X"=383415.43006836623, "Y"=283542.2712338854}, {"X"=383414.9873353622, "Y"=283542.51760912524}, {"X"=383414.50993287616, "Y"=283542.67447409057}, {"X"=383414.0436657404, "Y"=283542.73165373795}, {"X"=383413.5880852258, "Y"=283542.7113413258}, {"X"=383413.1160673846, "Y"=283542.60188727773}, {"X"=383412.6638522345, "Y"=283542.41512548324}, {"X"=383412.2316641198, "Y"=283542.1399593133}, {"X"=383412.1058336066, "Y"=283542.04860588827}, {"X"=383412.09671750874, "Y"=283542.04842157435}, {"X"=383412.1058336066, "Y"=283542.04860588827}, {"X"=383412.1149497068, "Y"=283542.04879020224}, {"X"=383412.12406580243, "Y"=283542.04897451616}, {"X"=383412.13295754296, "Y"=283542.0602554593}, {"X"=383412.13295754296, "Y"=283542.0602554593}, {"X"=383412.14207364316, "Y"=283542.06043977325}, {"X"=383412.1511897411, "Y"=283542.06062408723}, {"X"=383412.160305839, "Y"=283542.0608084012}]  # wpt_polypusan_20200714-3
  (unwired) cluster{"X":dbl, "Y":dbl}[] [{"X"=383411.932320843, "Y"=283542.5113466384}, {"X"=383411.94143694045, "Y"=283542.5115309522}, {"X"=383411.9503286807, "Y"=283542.5228118937}, {"X"=383411.95944477816, "Y"=283542.5229962075}, {"X"=383411.96856087557, "Y"=283542.5231805213}, {"X"=383411.9683365184, "Y"=283542.53427715093}, {"X"=383411.9774526181, "Y"=283542.5344614648}, {"X"=383411.9865687132, "Y"=283542.53464577853}, {"X"=383411.9956848153, "Y"=283542.5348300925}, {"X"=383411.8696299463, "Y"=283542.4545732997}, {"X"=383411.6993407283, "Y"=283542.3068151703}, {"X"=383411.54683498706, "Y"=283542.18161892693}, {"X"=383411.37654576113, "Y"=283542.0338608031}, {"X"=383411.1517842929, "Y"=283541.87390017736}, {"X"=383410.8998988804, "Y"=283541.7022899903}, {"X"=383410.62978125946, "Y"=283541.5303111862}, {"X"=383410.3509962426, "Y"=283541.33595482114}, {"X"=383410.072211214, "Y"=283541.1415984661}, {"X"=383409.7754183256, "Y"=283540.9357768668}, {"X"=383409.4697336811, "Y"=283540.71867434034}, {"X"=383409.146265533, "Y"=283540.47900994436}, {"X"=383408.83146475896, "Y"=283540.26172312885}, {"X"=383408.5526796635, "Y"=283540.0673668221}, {"X"=383408.28256195365, "Y"=283539.8953880912}, {"X"=383408.0122198793, "Y"=283539.7345059978}, {"X"=383407.7872339495, "Y"=283539.5856420879}, {"X"=383407.6249389544, "Y"=283539.4935514922}, {"X"=383407.4177365061, "Y"=283539.36724946724}, {"X"=383407.18341010157, "Y"=283539.2292978924}, {"X"=383406.9399675942, "Y"=283539.0911620164}, {"X"=383406.6513932718, "Y"=283538.92991135013}, {"X"=383406.33591933665, "Y"=283538.74591451185}, {"X"=383405.98465403315, "Y"=283538.5278905661}, {"X"=383405.6333887108, "Y"=283538.3098666383}, {"X"=383405.2641155198, "Y"=283538.080377482}, {"X"=383404.8590509454, "Y"=283537.8168612309}, {"X"=383404.4450945958, "Y"=283537.54206406383}, {"X"=383404.04025432153, "Y"=283537.2674512232}, {"X"=383403.6443057818, "Y"=283537.00411933445}, {"X"=383403.2485815608, "Y"=283536.7296908353}, {"X"=383402.85263297544, "Y"=283536.4663589834}, {"X"=383402.4389008485, "Y"=283536.18046528485}, {"X"=383402.025168696, "Y"=283535.89457160764}, {"X"=383401.6474522479, "Y"=283535.6316084193}, {"X"=383401.2877436384, "Y"=283535.38011048}, {"X"=383400.94694025436, "Y"=283535.0956912774}, {"X"=383400.62571511255, "Y"=283534.74506092304}, {"X"=383400.3509678404, "Y"=283534.35096557817}, {"X"=383400.140930653, "Y"=283533.9137738416}, {"X"=383399.99582789536, "Y"=283533.42238907877}, {"X"=383399.9518996638, "Y"=283532.8886451223}, {"X"=383399.9995811818, "Y"=283532.33455092355}, {"X"=383400.1475398879, "Y"=283531.782484042}, {"X"=383400.4042188871, "Y"=283531.26591866364}, {"X"=383400.7318076984, "Y"=283530.8506973626}, {"X"=383401.120965875, "Y"=283530.54773247044}, {"X"=383401.56325033365, "Y"=283530.32354980666}, {"X"=383402.03998015146, "Y"=283530.1999740305}, {"X"=383402.5151395754, "Y"=283530.15407467587}, {"X"=383402.9796124794, "Y"=283530.1856674368}, {"X"=383403.4247314314, "Y"=283530.2723747546}, {"X"=383403.85004773084, "Y"=283530.4363898795}, {"X"=383404.2922501598, "Y"=283530.6673534074}, {"X"=383404.74311997613, "Y"=283530.92069452035}, {"X"=383405.16664144257, "Y"=283531.17348273523}, {"X"=383405.61751120875, "Y"=283531.42682389263}, {"X"=383406.08594012377, "Y"=283531.7138235732}, {"X"=383406.5452528999, "Y"=283532.00063897157}, {"X"=383407.04013267846, "Y"=283532.33257814153}, {"X"=383407.5619120408, "Y"=283532.6872635217}, {"X"=383408.092583116, "Y"=283533.0532298735}, {"X"=383408.5968032415, "Y"=283533.37425681524}, {"X"=383409.08279111754, "Y"=283533.69491516484}, {"X"=383409.5692276718, "Y"=283533.9933802838}, {"X"=383410.10057165544, "Y"=283534.3260568743}, {"X"=383410.6854904599, "Y"=283534.7153225135}, {"X"=383411.26106875925, "Y"=283535.11550050834}, {"X"=383411.8279796103, "Y"=283535.493300969}, {"X"=383412.34998296807, "Y"=283535.83689001354}, {"X"=383412.82707883895, "Y"=283536.14626763324}, {"X"=383413.3495308398, "Y"=283536.4676634827}, {"X"=383413.89021501347, "Y"=283536.7894279925}, {"X"=383414.3762025273, "Y"=283537.11008664395}, {"X"=383414.844182165, "Y"=283537.4192800597}, {"X"=383415.32082914957, "Y"=283537.7508510744}, {"X"=383415.7781220907, "Y"=283538.1375366228}, {"X"=383416.1426834359, "Y"=283538.6000554199}, {"X"=383416.40562146157, "Y"=283539.12712650327}, {"X"=383416.53981222806, "Y"=283539.7071002825}, {"X"=383416.57305278804, "Y"=283540.31833644706}, {"X"=383416.451319649, "Y"=283540.92643920117}, {"X"=383416.2213151491, "Y"=283541.47684699734}, {"X"=383415.8748206522, "Y"=283541.92498900933}, {"X"=383415.43006836623, "Y"=283542.2712338854}, {"X"=383414.93241441366, "Y"=283542.5275998535}, {"X"=383414.4092070801, "Y"=283542.694639868}, {"X"=383413.8978081814, "Y"=283542.7287046846}, {"X"=383413.33350757346, "Y"=283542.6728906116}, {"X"=383412.79879883706, "Y"=283542.50666323025}, {"X"=383412.3112410692, "Y"=283542.2636810541}, {"X"=383412.1309383268, "Y"=283542.1601251152}, {"X"=383412.1222709437, "Y"=283542.13774754526}, {"X"=383412.1222709437, "Y"=283542.13774754526}, {"X"=383412.1316113989, "Y"=283542.12683523097}, {"X"=383412.1316113989, "Y"=283542.12683523097}, {"X"=383412.1316113989, "Y"=283542.12683523097}, {"X"=383412.1316113989, "Y"=283542.12683523097}, {"X"=383412.1316113989, "Y"=283542.12683523097}, {"X"=383412.14072749903, "Y"=283542.12701954495}, {"X"=383412.14984359685, "Y"=283542.1272038589}]  # poly pusan 20200714-2
  (unwired) cluster{"X":dbl, "Y":dbl}[] [{"X"=383409.9178374654, "Y"=283536.59810102}, {"X"=383409.927177923, "Y"=283536.58718870144}, {"X"=383409.93651838053, "Y"=283536.57627638616}, {"X"=383409.9549749438, "Y"=283536.5655483811}, {"X"=383409.96431539906, "Y"=283536.55463606486}, {"X"=383409.973655859, "Y"=283536.5437237469}, {"X"=383409.98277195997, "Y"=283536.54390805843}, {"X"=383409.9469806094, "Y"=283536.50988092675}, {"X"=383409.93831321446, "Y"=283536.4875033598}, {"X"=383409.9385375687, "Y"=283536.4764067302}, {"X"=383409.9385375687, "Y"=283536.4764067302}, {"X"=383409.93876192294, "Y"=283536.4653101011}, {"X"=383409.8578387605, "Y"=283536.40816815686}, {"X"=383409.7769156017, "Y"=283536.35102621204}, {"X"=383409.7589077463, "Y"=283536.3395609602}, {"X"=383409.73200814123, "Y"=283536.3168147713}, {"X"=383409.5792779161, "Y"=283536.20271519583}, {"X"=383409.27336874546, "Y"=283535.99670931126}, {"X"=383408.841180219, "Y"=283535.72154332086}, {"X"=383408.3816433538, "Y"=283535.4458244228}, {"X"=383408.05727756815, "Y"=283535.25054659066}, {"X"=383407.9223308085, "Y"=283535.15900892194}, {"X"=383407.94056302006, "Y"=283535.15937754087}, {"X"=383408.09396634065, "Y"=283535.2401872}, {"X"=383408.3194010837, "Y"=283535.36685785564}, {"X"=383408.61776466237, "Y"=283535.4950029968}, {"X"=383409.05421591504, "Y"=283535.55933303706}, {"X"=383409.60140653874, "Y"=283535.55929506075}, {"X"=383410.21285860625, "Y"=283535.5383540437}, {"X"=383410.69646085746, "Y"=283535.52592932346}, {"X"=383410.96971964114, "Y"=283535.5425553223}, {"X"=383411.1155773138, "Y"=283535.5455043238}, {"X"=383411.3519229675, "Y"=283535.5835863414}, {"X"=383411.5695876939, "Y"=283535.64349299634}, {"X"=383411.6963157314, "Y"=283535.69045989437}, {"X"=383411.94954744837, "Y"=283535.7954903261}, {"X"=383412.0940589766, "Y"=283535.86501911347}, {"X"=383412.17520648835, "Y"=283535.9110644512}, {"X"=383412.2472378928, "Y"=283535.95692547486}, {"X"=383412.2743618502, "Y"=283535.9685750442}, {"X"=383412.2743618502, "Y"=283535.9685750442}, {"X"=383412.2741374931, "Y"=283535.9796716734}, {"X"=383412.2741374931, "Y"=283535.9796716734}, {"X"=383412.2741374931, "Y"=283535.9796716734}, {"X"=383412.2741374931, "Y"=283535.9796716734}, {"X"=383412.2741374931, "Y"=283535.9796716734}, {"X"=383412.2741374931, "Y"=283535.9796716734}, {"X"=383412.2741374931, "Y"=283535.9796716734}, {"X"=383412.2741374931, "Y"=283535.9796716734}, {"X"=383412.2743618502, "Y"=283535.9685750442}, {"X"=383412.26524574624, "Y"=283535.9683907304}, {"X"=383412.2650213891, "Y"=283535.9794873595}, {"X"=383412.2650213891, "Y"=283535.9794873595}, {"X"=383412.2559052828, "Y"=283535.97930304566}, {"X"=383412.291920987, "Y"=283536.0022335576}, {"X"=383412.53581222554, "Y"=283536.11817631975}, {"X"=383412.77970346273, "Y"=283536.2341190897}, {"X"=383412.987578986, "Y"=283536.3271313491}, {"X"=383413.19545451214, "Y"=283536.42014361545}, {"X"=383413.367089974, "Y"=283536.5013219984}, {"X"=383413.49336927186, "Y"=283536.5704821794}, {"X"=383413.5293849731, "Y"=283536.59341269743}, {"X"=383413.5385010765, "Y"=283536.5935970126}, {"X"=383413.5567332834, "Y"=283536.5939656429}, {"X"=383413.56584938685, "Y"=283536.59414995805}, {"X"=383413.5749654926, "Y"=283536.59433427325}, {"X"=383413.71013653226, "Y"=283536.6747754009}, {"X"=383414.22324801044, "Y"=283537.0070836166}, {"X"=383414.9242078476, "Y"=283537.5208085642}, {"X"=383415.63002084335, "Y"=283538.2455538307}, {"X"=383416.1836939611, "Y"=283539.2780556692}, {"X"=383416.2779721501, "Y"=283540.4788876928}, {"X"=383415.9344532047, "Y"=283541.68196908606}, {"X"=383415.1402897733, "Y"=283542.62061217}, {"X"=383414.0938751328, "Y"=283542.95469220664}, {"X"=383413.47308307973, "Y"=283542.9865452564}, {"X"=383413.3452333581, "Y"=283542.9950614707}, {"X"=383413.3267768075, "Y"=283543.0057894686}, {"X"=383413.3174363517, "Y"=283543.01670178166}, {"X"=383413.38102467154, "Y"=283543.0290886174}, {"X"=383413.9084121501, "Y"=283543.1063586886}, {"X"=383414.70860945265, "Y"=283543.2224481709}, {"X"=383414.95384662825, "Y"=283543.2718112374}, {"X"=383414.95362226735, "Y"=283543.2829078666}, {"X"=383414.9533979065, "Y"=283543.2940044949}, {"X"=383414.9531735456, "Y"=283543.3051011227}, {"X"=383414.9169335171, "Y"=283543.29326722753}, {"X"=383414.6076593038, "Y"=283543.25371057465}, {"X"=383413.9711030325, "Y"=283543.1631320421}, {"X"=383413.3634655521, "Y"=283542.9954301012}, {"X"=383412.93972051237, "Y"=283542.7537380956}, {"X"=383412.5989177596, "Y"=283542.4693184259}, {"X"=383412.09537136485, "Y"=283542.11500134604}, {"X"=383411.53690398356, "Y"=283541.77067504416}, {"X"=383411.0869323256, "Y"=283541.47294704843}, {"X"=383410.7814720845, "Y"=283541.2447478443}, {"X"=383410.583610174, "Y"=283541.1075334294}, {"X"=383410.466222666, "Y"=283541.04965422716}, {"X"=383410.4297582683, "Y"=283541.04891697824}, {"X"=383410.41130171315, "Y"=283541.059644982}, {"X"=383410.8434899318, "Y"=283541.33481106185}, {"X"=383411.3746090679, "Y"=283541.67858437833}, {"X"=383411.8963877096, "Y"=283542.03327004256}, {"X"=383412.49042201624, "Y"=283542.42272013833}, {"X"=383413.04044630117, "Y"=283542.7335723024}, {"X"=383413.4459591501, "Y"=283542.9748956804}, {"X"=383413.81545630284, "Y"=283543.1932885606}, {"X"=383414.26654959243, "Y"=283543.4355335569}, {"X"=383414.59158803057, "Y"=283543.59752174537}, {"X"=383414.6727354587, "Y"=283543.6435671087}, {"X"=383414.6725110981, "Y"=283543.65466373705}, {"X"=383414.663395004, "Y"=283543.6544794205}, {"X"=383414.5277753554, "Y"=283543.59623153013}, {"X"=383414.39215570525, "Y"=283543.53798364184}, {"X"=383414.1751642665, "Y"=283543.4447870245}, {"X"=383413.7863131391, "Y"=283543.2815086416}, {"X"=383413.42548336374, "Y"=283543.085493336}, {"X"=383413.1546927557, "Y"=283542.94680433837}, {"X"=383412.9650495782, "Y"=283542.854160697}, {"X"=383412.7938629567, "Y"=283542.75078906}, {"X"=383412.56865281187, "Y"=283542.6130216534}, {"X"=383412.41547401866, "Y"=283542.52111528144}, {"X"=383412.37056660216, "Y"=283542.48690382455}, {"X"=383412.36167486466, "Y"=283542.47562288266}, {"X"=383412.28120048554, "Y"=283542.39628765377}, {"X"=383412.2182852302, "Y"=283542.3506109417}, {"X"=383412.2091691326, "Y"=283542.3504266277}, {"X"=383412.2093934901, "Y"=283542.33932999894}, {"X"=383412.2093934901, "Y"=283542.33932999894}, {"X"=383412.2093934901, "Y"=283542.33932999894}, {"X"=383412.2093934901, "Y"=283542.33932999894}, {"X"=383412.2463065955, "Y"=283542.3178739988}, {"X"=383412.2554226954, "Y"=283542.31805831287}, {"X"=383412.2645387931, "Y"=283542.31824262696}, {"X"=383412.2738792506, "Y"=283542.3073303115}, {"X"=383412.1665052908, "Y"=283542.2052488859}, {"X"=383411.77922457363, "Y"=283541.9642941928}, {"X"=383411.38305209693, "Y"=283541.71205857664}, {"X"=383411.10381838854, "Y"=283541.5398954449}, {"X"=383410.8697164487, "Y"=283541.3908471426}, {"X"=383410.6447306024, "Y"=283541.2419831568}, {"X"=383410.41062864766, "Y"=283541.0929348684}, {"X"=383410.14940274344, "Y"=283540.9322370196}, {"X"=383409.9155251322, "Y"=283540.77209211467}, {"X"=383409.6903149036, "Y"=283540.6343247839}, {"X"=383409.43842942733, "Y"=283540.4627146399}, {"X"=383409.24056747806, "Y"=283540.3255002548}, {"X"=383409.17765219585, "Y"=283540.27982356516}, {"X"=383409.2585753234, "Y"=283540.3369655045}, {"X"=383409.5375847504, "Y"=283540.52022520616}, {"X"=383409.8617259532, "Y"=283540.7265997316}, {"X"=383410.20365063194, "Y"=283540.95553614816}, {"X"=383410.608939274, "Y"=283541.20795602264}, {"X"=383410.995546983, "Y"=283541.4822005473}, {"X"=383411.3283555053, "Y"=283541.7109526976}, {"X"=383411.68873666425, "Y"=283541.9291611722}, {"X"=383411.95862989506, "Y"=283542.1122366382}, {"X"=383412.12070044235, "Y"=283542.2154239456}, {"X"=383412.1567161209, "Y"=283542.2383544585}, {"X"=383412.1658322186, "Y"=283542.23853877245}, {"X"=383412.1658322186, "Y"=283542.23853877245}, {"X"=383412.1749483163, "Y"=283542.2387230865}, {"X"=383412.1749483163, "Y"=283542.2387230865}, {"X"=383412.2025209692, "Y"=283542.2281793989}, {"X"=383412.2025209692, "Y"=283542.2281793989}, {"X"=383412.2025209692, "Y"=283542.2281793989}, {"X"=383412.21163706464, "Y"=283542.22836371296}, {"X"=383412.21163706464, "Y"=283542.22836371296}, {"X"=383412.22052880493, "Y"=283542.2396446566}, {"X"=383412.22052880493, "Y"=283542.2396446566}, {"X"=383412.18496184365, "Y"=283542.1945208857}, {"X"=383412.09537136485, "Y"=283542.11500134604}, {"X"=383411.9788813051, "Y"=283542.0127356099}, {"X"=383411.8530507877, "Y"=283541.9213821895}, {"X"=383411.67274803354, "Y"=283541.8178262597}, {"X"=383411.46532133967, "Y"=283541.7026207666}, {"X"=383411.29413467535, "Y"=283541.59924916073}, {"X"=383411.1767471755, "Y"=283541.54136994836}, {"X"=383411.07759187114, "Y"=283541.48385936284}, {"X"=383410.9510882701, "Y"=283541.42579584295}, {"X"=383410.80702553515, "Y"=283541.33407381136}, {"X"=383410.6173823041, "Y"=283541.24143021955}, {"X"=383410.48198695586, "Y"=283541.1720857659}, {"X"=383410.4457469139, "Y"=283541.16025188734}, {"X"=383410.43663081515, "Y"=283541.1600675751}, {"X"=383410.3557076998, "Y"=283541.1029256232}, {"X"=383410.1934127563, "Y"=283541.0108349785}, {"X"=383410.0039938697, "Y"=283540.90709477285}, {"X"=383409.7696675421, "Y"=283540.769143129}, {"X"=383409.53511685575, "Y"=283540.6422881183}, {"X"=383409.3730462501, "Y"=283540.53910085984}, {"X"=383409.2380995876, "Y"=283540.44756316737}, {"X"=383409.04912938597, "Y"=283540.3216297263}, {"X"=383408.81480303186, "Y"=283540.1836781074}, {"X"=383408.55402578035, "Y"=283540.00078705046}, {"X"=383408.26590022095, "Y"=283539.817343072}, {"X"=383407.9686585453, "Y"=283539.63371479337}, {"X"=383407.67141686263, "Y"=283539.450086526}, {"X"=383407.3743995172, "Y"=283539.2553616379}, {"X"=383407.05025820807, "Y"=283539.0489872076}, {"X"=383406.71700078365, "Y"=283538.8424284801}, {"X"=383406.3926350932, "Y"=283538.64715070394}, {"X"=383406.04159413883, "Y"=283538.41803012847}, {"X"=383405.7174527709, "Y"=283538.2116557487}, {"X"=383405.4113192408, "Y"=283538.01674662315}, {"X"=383405.0869534989, "Y"=283537.8214688956}, {"X"=383404.7810442931, "Y"=283537.615463163}, {"X"=383404.4840268283, "Y"=283537.4207383768}, {"X"=383404.21413331095, "Y"=283537.2376631467}, {"X"=383403.9440154383, "Y"=283537.06568455126}, {"X"=383403.65588969685, "Y"=283536.8822407282}, {"X"=383403.36753959535, "Y"=283536.70989354217}, {"X"=383403.0525142093, "Y"=283536.5037035683}, {"X"=383402.692581331, "Y"=283536.26330219803}, {"X"=383402.3237566754, "Y"=283536.0116199123}, {"X"=383401.990947726, "Y"=283535.7828681109}, {"X"=383401.75729418325, "Y"=283535.61162680085}, {"X"=383401.6312391361, "Y"=283535.5313701584}, {"X"=383401.4962923195, "Y"=283535.4398325877}, {"X"=383401.2984301499, "Y"=283535.30261838617}, {"X"=383401.0827844499, "Y"=283535.1428423272}, {"X"=383400.8944870562, "Y"=283534.98361918115}, {"X"=383400.70641399856, "Y"=283534.8132994113}, {"X"=383400.5010060944, "Y"=283534.5982245295}, {"X"=383400.3060603416, "Y"=283534.3167541855}, {"X"=383400.13958460063, "Y"=283533.9803536106}, {"X"=383400.00157887576, "Y"=283533.5890228039}, {"X"=383399.91049971955, "Y"=283533.1320337348}, {"X"=383399.89302243193, "Y"=283532.64322919585}, {"X"=383399.93890921294, "Y"=283532.17790802126}, {"X"=383400.04703835654, "Y"=283531.79155335313}, {"X"=383400.18049675727, "Y"=283531.50562124373}, {"X"=383400.30304432334, "Y"=283531.3082778588}, {"X"=383400.38800574763, "Y"=283531.1656804091}, {"X"=383400.50053984235, "Y"=283531.0125392357}, {"X"=383400.68712452496, "Y"=283530.8053893417}, {"X"=383400.8917170911, "Y"=283530.60970468115}, {"X"=383401.1596737439, "Y"=283530.43750339915}, {"X"=383401.4545300481, "Y"=283530.2880482896}, {"X"=383401.78517776896, "Y"=283530.17262028495}, {"X"=383402.16984912794, "Y"=283530.09158799663}, {"X"=383402.58052275726, "Y"=283530.07768840576}, {"X"=383402.9811828962, "Y"=283530.1079910402}, {"X"=383403.37115650147, "Y"=283530.2157857858}, {"X"=383403.8138076402, "Y"=283530.42455603235}, {"X"=383404.3193741375, "Y"=283530.6790029523}, {"X"=383404.7793600638, "Y"=283530.93252837134}, {"X"=383405.14863357117, "Y"=283531.1620174932}, {"X"=383405.4187516078, "Y"=283531.3339961164}, {"X"=383405.5988302973, "Y"=283531.4486485354}, {"X"=383405.77868462657, "Y"=283531.5743975866}, {"X"=383405.95876330684, "Y"=283531.6890500145}, {"X"=383406.19264122855, "Y"=283531.8491948027}, {"X"=383406.51633412845, "Y"=283532.0777624464}, {"X"=383406.8495918177, "Y"=283532.2843211534}, {"X"=383407.1286015494, "Y"=283532.4675807652}, {"X"=383407.4076112677, "Y"=283532.650840386}, {"X"=383407.70485319116, "Y"=283532.83446863596}, {"X"=383408.00187074905, "Y"=283533.0291935228}, {"X"=383408.3353527256, "Y"=283533.2246556581}, {"X"=383408.66838598094, "Y"=283533.44231106626}, {"X"=383408.97474396054, "Y"=283533.6261236677}, {"X"=383409.27176146646, "Y"=283533.8208486002}, {"X"=383409.61368643295, "Y"=283534.04978498194}, {"X"=383410.0009675565, "Y"=283534.2907395623}, {"X"=383410.39736476535, "Y"=283534.5318784738}, {"X"=383410.76641363365, "Y"=283534.7724644647}, {"X"=383411.117454633, "Y"=283535.0015852203}, {"X"=383411.4778360758, "Y"=283535.2197936726}, {"X"=383411.8831249549, "Y"=283535.4722135931}, {"X"=383412.2695085299, "Y"=283535.75755479146}, {"X"=383412.6385573031, "Y"=283535.9981408621}, {"X"=383412.9624742541, "Y"=283536.21561212145}, {"X"=383413.2866155505, "Y"=283536.4219867639}, {"X"=383413.62876467826, "Y"=283536.6398266781}, {"X"=383413.9800298931, "Y"=283536.85785092146}, {"X"=383414.3404111968, "Y"=283537.0760594928}, {"X"=383414.6736685308, "Y"=283537.28261850367}, {"X"=383414.979801905, "Y"=283537.47752794967}, {"X"=383415.28571090545, "Y"=283537.6835340353}, {"X"=383415.5911711697, "Y"=283537.91173338844}, {"X"=383415.88616914465, "Y"=283538.20632820437}, {"X"=383416.1620374513, "Y"=283538.5449409112}, {"X"=383416.38231168006, "Y"=283538.92683423456}, {"X"=383416.54744055454, "Y"=283539.3298149099}, {"X"=383416.64808362443, "Y"=283539.764795244}, {"X"=383416.66623305104, "Y"=283540.22030997305}, {"X"=383416.6021132184, "Y"=283540.6852624638}, {"X"=383416.4381650218, "Y"=283541.1259941986}, {"X"=383416.22930943617, "Y"=283541.53251445986}, {"X"=383415.9393064278, "Y"=283541.89298934815}, {"X"=383415.58638820087, "Y"=283542.2077875092}, {"X"=383415.21680833364, "Y"=283542.4445406474}, {"X"=383414.83945855283, "Y"=283542.6145297139}, {"X"=383414.4547875691, "Y"=283542.6955614495}, {"X"=383414.0258822629, "Y"=283542.70909185003}, {"X"=383413.5434021757, "Y"=283542.6660332347}, {"X"=383413.0713843318, "Y"=283542.55657918955}, {"X"=383412.6456200371, "Y"=283542.41475685424}, {"X"=383412.2850145638, "Y"=283542.2076449687}, {"X"=383412.1767431755, "Y"=283542.1499500583}, {"X"=383412.1767431755, "Y"=283542.1499500583}, {"X"=383412.1767431755, "Y"=283542.1499500583}, {"X"=383412.17651881813, "Y"=283542.1610466851}, {"X"=383412.17651881813, "Y"=283542.1610466851}]  # poly pusan 20200714-1
  n1 = call-poly "VISA Configure Serial Port"("VISA resource name"="Port", "baud rate (9600)"="baud rate") -> ("VISA resource name out"=w7:refnum<visa-resource-name>, "error out"=w3:errorcluster)  [unwired: 12 in]
  n2 = while {
    shift-right: [w13] -> w8
    shift-left: w7 -> [w29]
    shift-right: [w22] -> _
    shift-left: "" -> [w27]
    shift-right: [w25] -> _
    shift-left: _ -> [w23]
    tunnel: w3 -> [w21]
    tunnel: [w14] -> w2
    stop <- w18 stop-if-true
    n3 = property class="Instr"(reference=w29, error in=w21) -> (reference out=w30:refnum<visa-resource-name>, error out=w20:errorcluster, "Serial Settings:Number of Bytes at Serial Port"=w26:u32)
    "r buff" <- w26
    n4 = Wait (ms)(milliseconds to wait=u32 20 ("대기 시간 (ms)")) -> ()  [unwired: 1 out]
    n5 = VISA Read(VISA resource name=w30, byte count=w26, error in (no error)=w20) -> (VISA resource name out=w15:refnum<visa-resource-name>, read buffer=w17:string, error out=w16:errorcluster)  [unwired: 1 out]
    "버퍼 읽기" <- w17
    n6 = case shown="거짓" "data-const" {
      tunnel: w27 -> [w44 w47]
      tunnel: [w44 w46] -> w22
      tunnel: w17 -> [_ w45]
      frame False {
      }
      frame True {
        n7 = Concatenate Strings(w47, w45) -> (w46:string)
      }
    }
    "문자열" <- w22
    n8 = call "sub_NMEA-LatLong.vi"("nmea sel"="nmea sel", "gnss str"=w17) -> ("latlong"=w10:cluster{"Lat":dbl, "Long":dbl}, "val"=w11:bool)  [unwired: 8 in]
    "val" <- w11
    "latlong" <- w10
    n9 = case shown="참" w11 {
      tunnel: [w38 w43] -> w25
      tunnel: w23 -> [w38 w42]
      tunnel: w17 -> [_ w40]
      tunnel: w10 -> [_ w39]
      frame False {
      }
      frame True {
        n10 = call "sub_wgs-84 to tm.vi"("in_lon-lat"=w39) -> ("TM"=w41:cluster{"Y(E)":dbl, "X(N)":dbl})  [unwired: 10 in]
        n11 = Build Array (concatenate)(w42, w41) -> (w43:cluster{"Y(E)":dbl, "X(N)":dbl}[])
        "after sting" <- w40
      }
    }
    n12 = Or(x=w16, y="정지") -> (x .or. y?=w18:bool)
    n13 = case shown="거짓" "write" {
      tunnel: w16 -> [w31 w37]
      tunnel: w15 -> [w32 w36]
      tunnel: [w31 w35] -> w14
      tunnel: [w32 w34] -> w13
      frame False {
      }
      frame True {
        n14 = VISA Write(VISA resource name=w36, write buffer="data_w", error in (no error)=w37) -> (VISA resource name out=w34:refnum<visa-resource-name>, error out=w35:errorcluster)  [unwired: 1 out]
      }
    }
    "routh graph" <- w23
  }
  n15 = VISA Close(VISA resource name=w8, error in (no error)=w2) -> (error out=→"error out":errorcluster)
